vi "Actor Core.vi"(8 "error in":errorcluster, 11 "DataLogger in":refnum<class "DataLogger.lvclass">) -> (0 "error out":errorcluster, 3 "Actor out":refnum<class "Actor.lvclass">)   [LabVIEW 2019, in "DataLogger.lvclass"]
doc: "(<B>Filename</B>: Actor Framework.lvlib:Actor.lvclass:Actor Core.vi)\n\nReceives messages to the actor, reacts to them, and initiates any error handling that may shut the actor down.\n\nDescendant classes may override this VI to append parallel tasks for the actor to complete while it handles messages. Overrides use the Call Parent Method node."
uses:
  DataLogger.lvclass
  <vilib>/ActorFramework/Actor/Actor.lvclass
  <vilib>/drjdpowell/SQLite Library/SQL Connection/Execute SQL (No results).vi
  <vilib>/drjdpowell/SQLite Library/SQL Connection/Connection.lvclass
  <vilib>/drjdpowell/SQLite Library/SQL Connection/Open (path).vi
  <vilib>/ActorFramework/Message Enqueuer/Message Enqueuer.lvclass
  <vilib>/vision/Image Controls.llb/IMAQ Image.ctl
  Common/Controls/AllPartInfo.ctl
  Controls/LocalData_DL.ctl
  <vilib>/Utility/file.llb/Write Delimited Spreadsheet (string).vi
  C:/Program Files/National Instruments/LabVIEW 2019/vi.lib/ActorFramework/Actor/Actor.lvclass
  Controls/LocalData_Measurements_DL.ctl
panel:
  in  "PartDetails":T1
  in  "Cluster":T2={"Core"={"Current VI Reference"=refnum, "Close Panel on Exit?"=FALSE}, "AllPartInfoArray"=[{"PartName"="", "NumberOfRacks"=0, "MeasurementIDsArray"=[], "MeasurementNamesArray"=[], "SpecValuesArray"=[]}], "PartDetails"={"PartName"="", "OperatorName"="", "Initialize"=TRUE, "MeasurementEnable/DisableArray"=[], "NumberOfMeasurements"=0}, "BatchID"="", "MeasurementInfo"={"MeasurementDate"="", "MeasurementTime"="", "MeasurementResult"="", "MeasurementValueArray"=[]}, "MachineStatus"="", "CurrentState"="", "StateMessage"="", "MeasurementDetails"={"Array(2D)"=[], "IndexCounter"=0}, "RecordsInExcelCounter"=0, "ExcelSheetCounterPerReel"=0, "ReelCounterPerPart"=0, "WriteMeasurementData"=FALSE, "MeasurementExcelPath"=path "", "StripPath"=FALSE, "MasterSampleInfo"={"MSPartName"="", "MSDate"="", "MSTime"="", "MSMeasurementValueArray"=[], "MSResult"="", "NumberOfMeasurements"=0}, "MasterSampleDetails"={"Array(2D)"=[], "IndexCounter"=0}, "Stamping Mc Details"={"Customer Name"="", "Location"="", "StampingMcID"=""}}
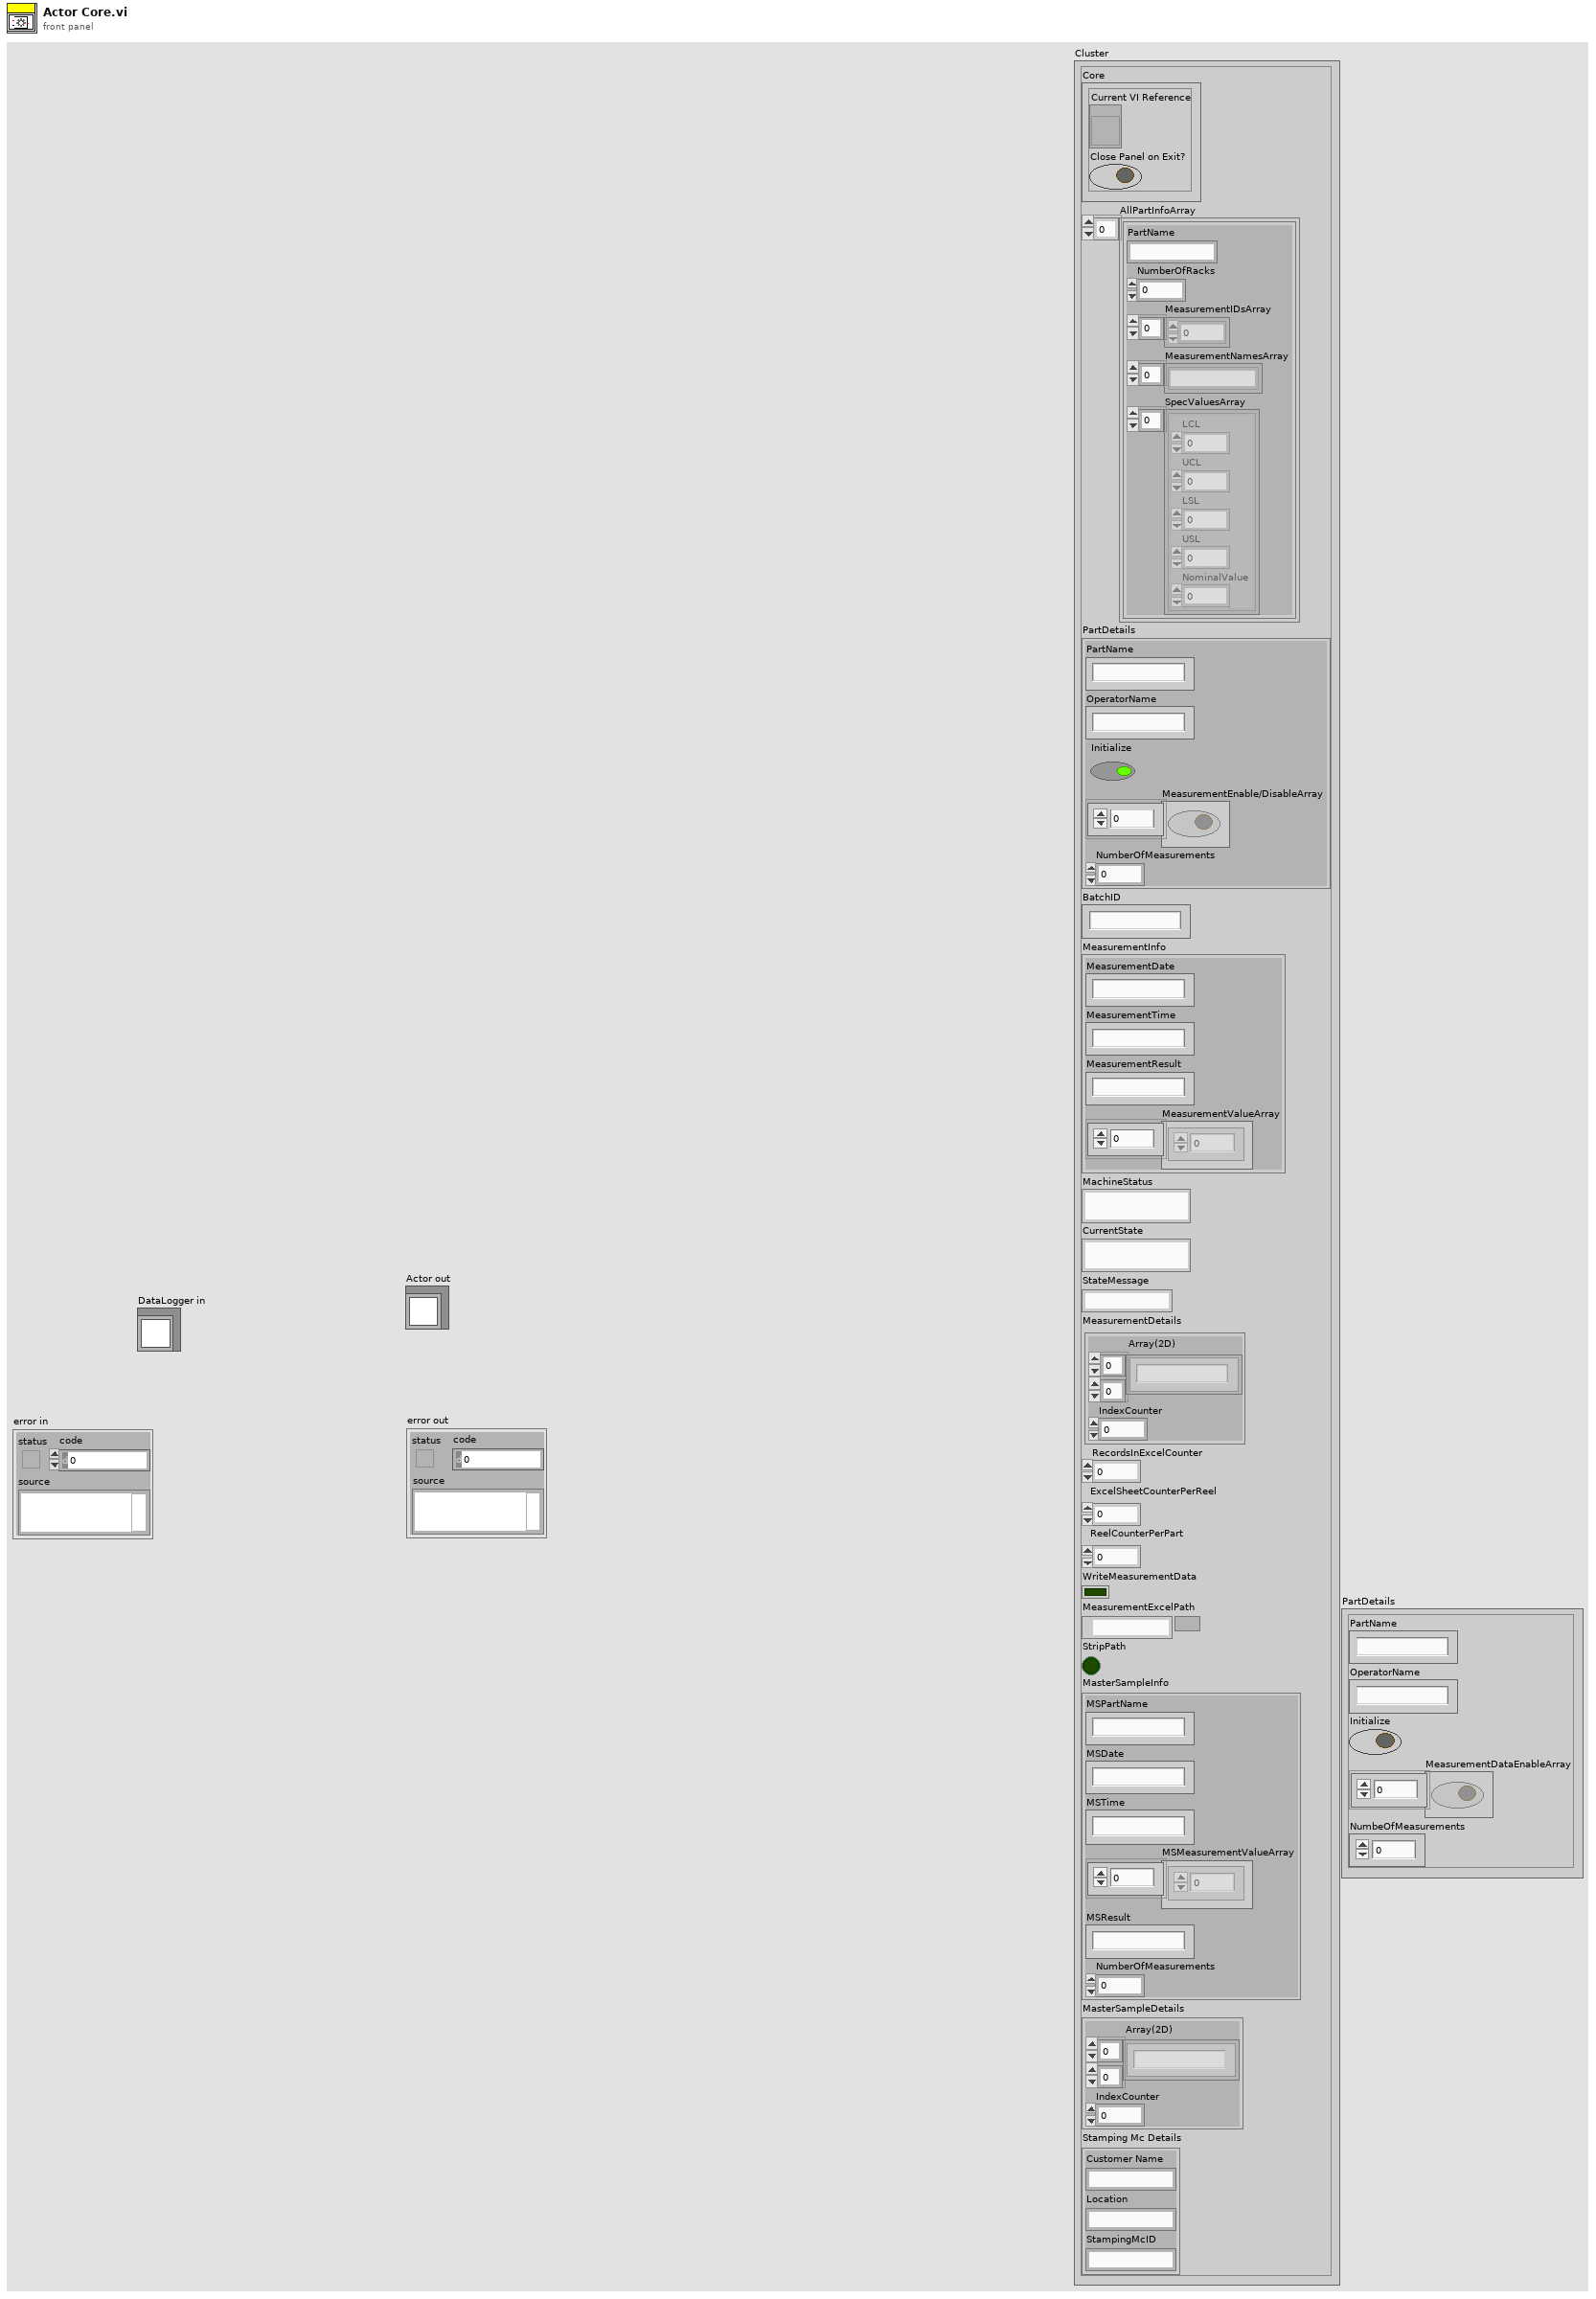
[diagram p1: front panel]
types:
  T1 = cluster{"PartName":string, "OperatorName":string, "Initialize":bool, "MeasurementDataEnableArray":bool[], "NumbeOfMeasurements":i32}
  T2 = typedef "DataLogger.lvclass/LocalData_Measurements_DL.ctl" = cluster{"Core":cluster{"Current VI Reference":refnum<vi>, "Close Panel on Exit?":bool}, "AllPartInfoArray":T3, "PartDetails":cluster{"PartName":string, "OperatorName":string, "Initialize":bool, "MeasurementEnable/DisableArray":bool[], "NumberOfMeasurements":i32}, "BatchID":string, "MeasurementInfo":cluster{"MeasurementDate":string, "MeasurementTime":string, "MeasurementResult":string, "MeasurementValueArray":dbl[]}, "MachineStatus":string, "CurrentState":string, "StateMessage":string, "MeasurementDetails":cluster{"Array(2D)":string[][], "IndexCounter":i32}, "RecordsInExcelCounter":i32, "ExcelSheetCounterPerReel":i32, "ReelCounterPerPart":i32, "WriteMeasurementData":bool, "MeasurementExcelPath":path, "StripPath":bool, "MasterSampleInfo":cluster{"MSPartName":string, "MSDate":string, "MSTime":string, "MSMeasurementValueArray":dbl[], "MSResult":string, "NumberOfMeasurements":i32}, "MasterSampleDetails":cluster{"Array(2D)":string[][], "IndexCounter":i32}, "Stamping Mc Details":cluster{"Customer Name":string, "Location":string, "StampingMcID":string}}
  T3 = typedef "AllPartInfo.ctl" = cluster{"PartName":string, "NumberOfRacks":u8, "MeasurementIDsArray":u16[], "MeasurementNamesArray":string[], "SpecValuesArray":cluster{"LCL":dbl, "UCL":dbl, "LSL":dbl, "USL":dbl, "NominalValue":dbl}[]}[]
  T4 = enum32{"invalid app kind", "Development System", "Run Time System", "Student Edition", "Embedded LabVIEW", "Evaluation", "Custom"}
  T5 = enum32{"Invalid", "Standard", "Closed", "Hidden", "Minimized", "Maximized"}
  T6 = cluster{"Current VI Reference":refnum<vi>, "Close Panel on Exit?":bool}
  T7 = cluster{"CreateNewEventsExcel":bool, "CreateNewFailExcel":bool, "CreateNewStatisticalExcel":bool, "CreateNewReelExcel":bool}
  T8 = cluster{"EventsSheetCounter":u32, "FailSheetCounter":u32, "StatisticalSheetCounter":u32, "ReelSheetCounter":u32}
  T9 = typedef "DataLogger.lvclass/LocalData_DL.ctl" = cluster{"Core":cluster{"Current VI Reference":refnum<vi>, "Close Panel on Exit?":bool}, "System Info":cluster{"System Name":string, "System ID":string, "Version":string, "Year":string, "Customer Details":cluster{"Customer Name":string, "Customer ID":string, "Location":string, "No of Shifts":u8, "Shift Details Array":cluster{"Name":string, "Timing":string}[]}, "Software Features":cluster{"IoT Enable":bool, "Datalogging Features":cluster{"Event Data":bool, "Measurement Data":bool, "Statistical Data":bool, "Reel Data":bool, "Failed Measurement Data":bool, "Failed Images":bool}, "IoT":cluster{"SMS Alert Enable":bool, "Email Alert Enable":bool}, "Popup Enable?":cluster{"Fail":bool, "Pause":bool, "Stop":bool}}}, "Part Info":cluster{"Part Name":string, "Rack ID":u8, "Initialize":bool, "StampingMc No":u64, "Operator Name":string, "ReelCount":u64, "TotalCount":u64, "Measurement Names Array":string[], "Measurement ID Array":u16[], "Spec Values Array":cluster{"LCL":dbl, "UCL":dbl, "LSL":dbl, "USL":dbl, "Nominal Value":dbl}[], "Camera Name Array":string[], "Measurement Enable/Disable Array":bool[], "Number of Measurements":i32}, "Fail Counter(For Event Details)":i32, "Event Details":cluster{"Event Name":string, "Event Time":string, "Event Reason":string, "Previous Event Name":string, "Previous Event Time":string}, "StatisticalInfo":string[][], "BatchInfo":cluster{"BatchPassCount":u64, "BatchFailCount":u64}, "Failure Details":cluster{"Fail Time Stamp":u64, "ControlPFArray":bool[], "SpecificationPFArray":dbl[], "Rack ID":u8, "Failed Image Array":T10[], "Fail Date":string, "Fail Time":string, "Fail Reason":string}, "SaveFailedImageCounter":i32, "AllPartInfoArray":T3, "Status":bool, "SpecValues(ForUpdate)":cluster{"LCL":dbl, "UCL":dbl, "LSL":dbl, "USL":dbl, "Nominal Value":dbl}, "AddSuccessfull":bool, "CurrentStateMessage":string, "IoTDetailsCounter":bool, "InitialUpdate":bool, "ResetUpdate":bool, "SetCounter":cluster{"MeasurementDetailsSetCounter":i32, "BatchDetailsSetCounter":i32, "FailureDetailsSetCounter":i32, "EventDetailsSetCounter":i32}, "IndexCounter":cluster{"MeasurementDetailsIndexCounter":i32, "BatchDetailsIndexCounter":i32, "FailureDetailsIndexCounter":i32, "EventDetailsIndexCounter":i32}, "Details2D":cluster{"MeasurementDetails(2D)":string[][], "BatchDetails(2D)":string[][], "FailureDetails(2D)":string[][], "EventDetails(2D)":string[][]}, "IDs":cluster{"Stamping McID":string, "Inspection McID":string, "BatchID":string, "FailID":string}, "Reel Info":cluster{"Reel No":u64, "Reel Start Time Stamp":u64}, "ExcelData":cluster{"StripPath":bool, "ReelCounterPerPart":i32, "FilePaths":cluster{"EventsFilePath":path, "FailFilePath":path, "ReelFilePath":path, "StatisticalFilePath":path}, "ExcelSheetCounterPerReel":cluster{"EventsSheetCounter":u32, "FailSheetCounter":u32, "StatisticalSheetCounter":u32, "ReelSheetCounter":u32}, "CreateNewExcel":cluster{"CreateNewEventsExcel":bool, "CreateNewFailExcel":bool, "CreateNewStatisticalExcel":bool, "CreateNewReelExcel":bool}, "RecordsInExcelCounter":cluster{"EventsRecordsCounter":u32, "FailRecordsCounter":u32, "ReelRecordsCounter":u32, "StatisticalRecordsCounter":u32}}, "SaveAck":cluster{"Loop1":bool, "Loop2":bool}, "Shift Statistical Info":cluster{"Shift Name":string, "Shift Timing":string, "Shift End Date":string, "Statistical Shift Data":cluster{"PartName":string, "MeasurementNames":string[], "Statistical Parameters":string[][]}[]}}
  T10 = typedef "IMAQ Image.ctl" = refnum<image>
  T11 = cluster{"Customer Name":string, "Customer ID":string, "Location":string, "No of Shifts":u8, "Shift Details Array":cluster{"Name":string, "Timing":string}[]}
  T12 = cluster{"IoT Enable":bool, "Datalogging Features":cluster{"Event Data":bool, "Measurement Data":bool, "Statistical Data":bool, "Reel Data":bool, "Failed Measurement Data":bool, "Failed Images":bool}, "IoT":cluster{"SMS Alert Enable":bool, "Email Alert Enable":bool}, "Popup Enable?":cluster{"Fail":bool, "Pause":bool, "Stop":bool}}
  T13 = cluster{"LCL":dbl, "UCL":dbl, "LSL":dbl, "USL":dbl, "Nominal Value":dbl}[]
  T14 = cluster{"PartName":string, "MeasurementNames":string[], "Statistical Parameters":string[][]}[]
  T15 = cluster{"EventsRecordCounter":u32, "FailRecordCounter":u32, "ReelRecordCounter":u32, "StatisticalRecordCounter":u32}
  T16 = cluster{"Acknowledgement":cluster{"Enqueuer":refnum<class "Message Enqueuer.lvclass">, "VIReference":refnum<vi>, "VIName":string}, "ErrorMessage":string}
  T17 = cluster{"Customer ID":string, "Customer Name":string, "Location":string, "No of Shifts":u8, "Inspection McID":string, "Shift Details Array":cluster{"Name":string, "Timing":string}[], "IoT Enable":bool, "SMS Alert Enable":bool, "Email Alert Enable":bool, "FailPopupEnable":bool, "PausePopupEnable":bool, "StopPopupEnable":bool}
  T18 = cluster{"LCL":dbl, "UCL":dbl, "LSL":dbl, "USL":dbl, "NominalValue":dbl}[]
  T19 = cluster{"Inspection McID":string, "PartName":string, "MeasurementNamesArray":string[], "SpecValuesArray":cluster{"LCL":dbl, "UCL":dbl, "LSL":dbl, "USL":dbl, "NominalValue":dbl}[]}
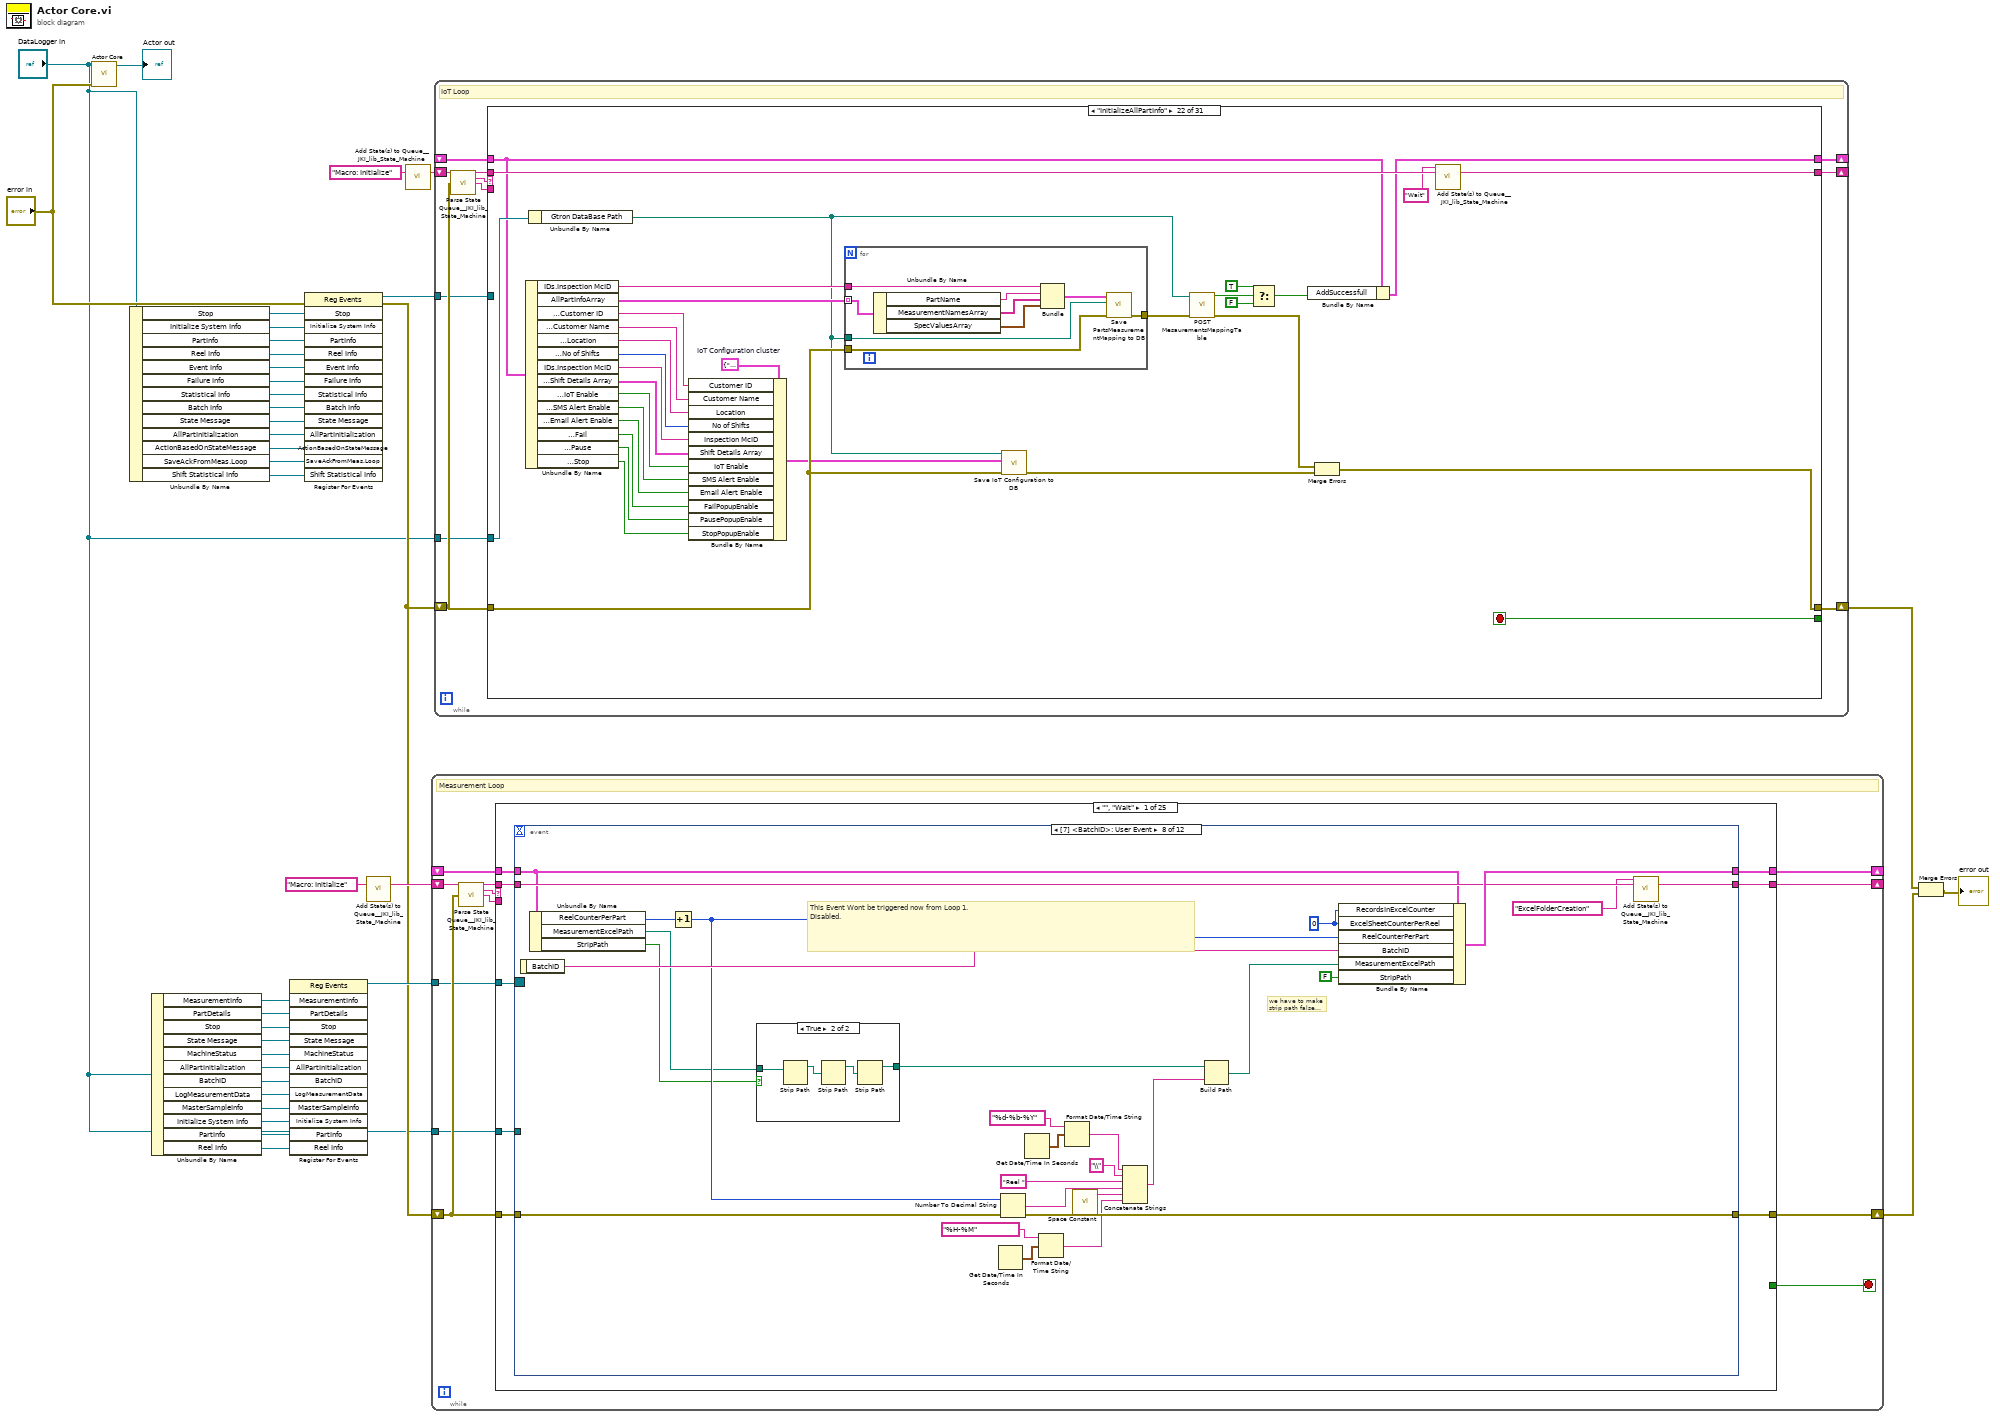
[diagram p0: block diagram]
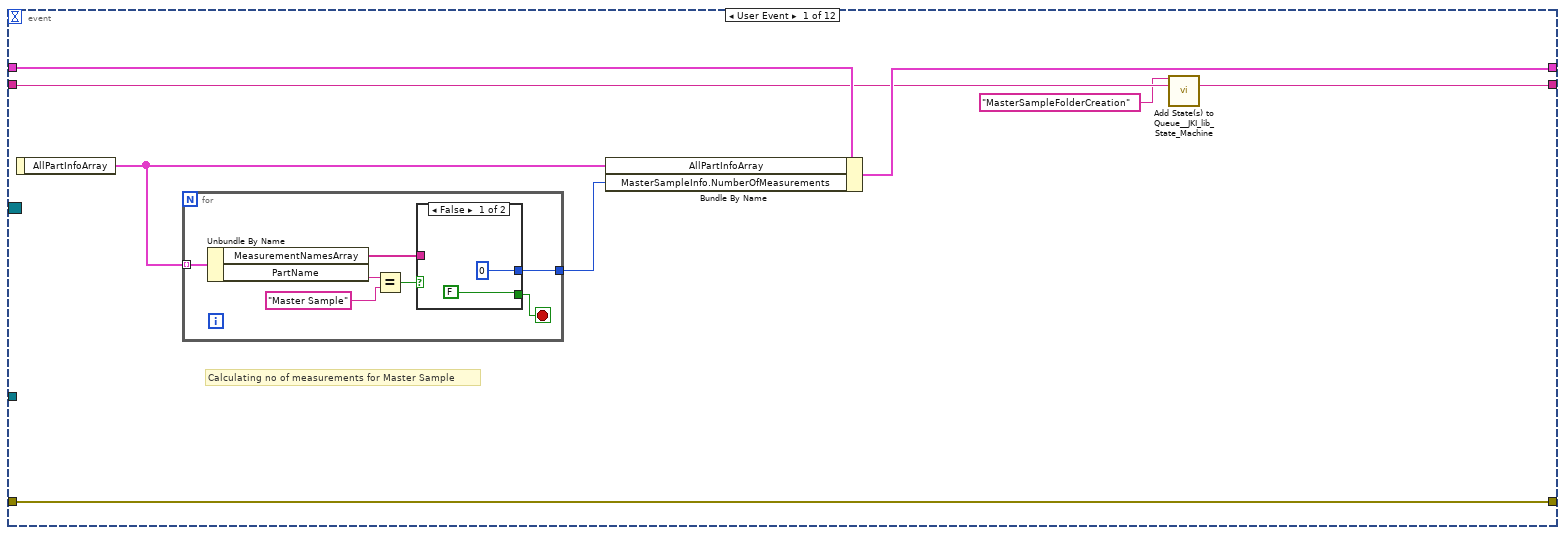
[diagram p2: hidden frame]
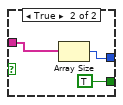
[diagram p3: hidden frame]
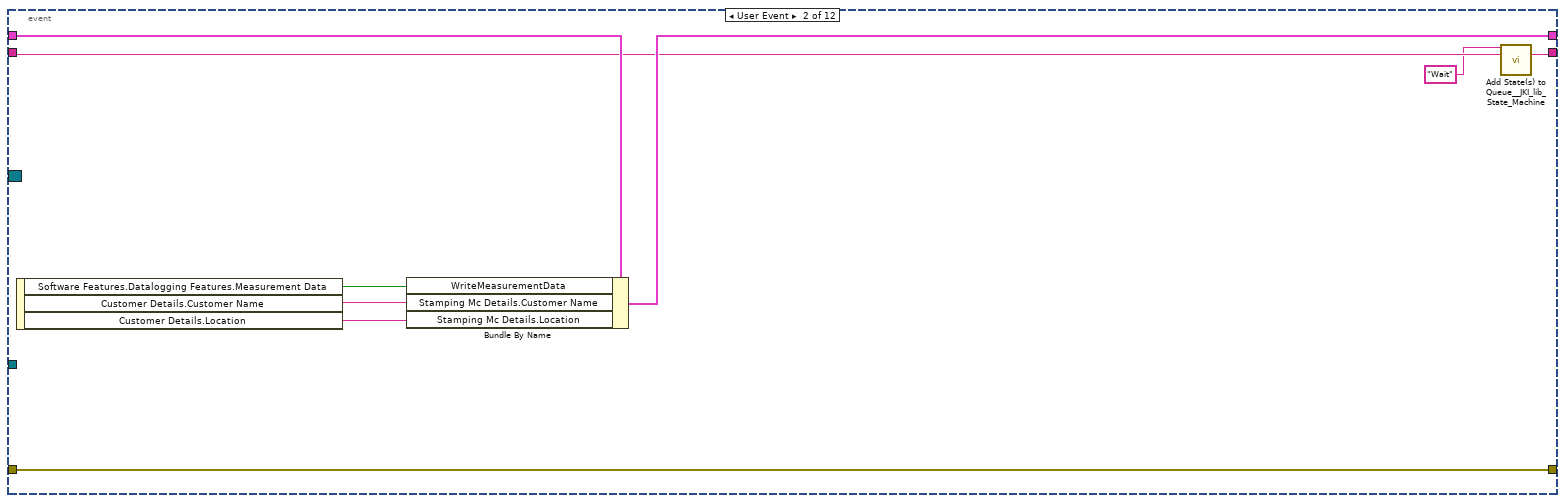
[diagram p4: hidden frame]
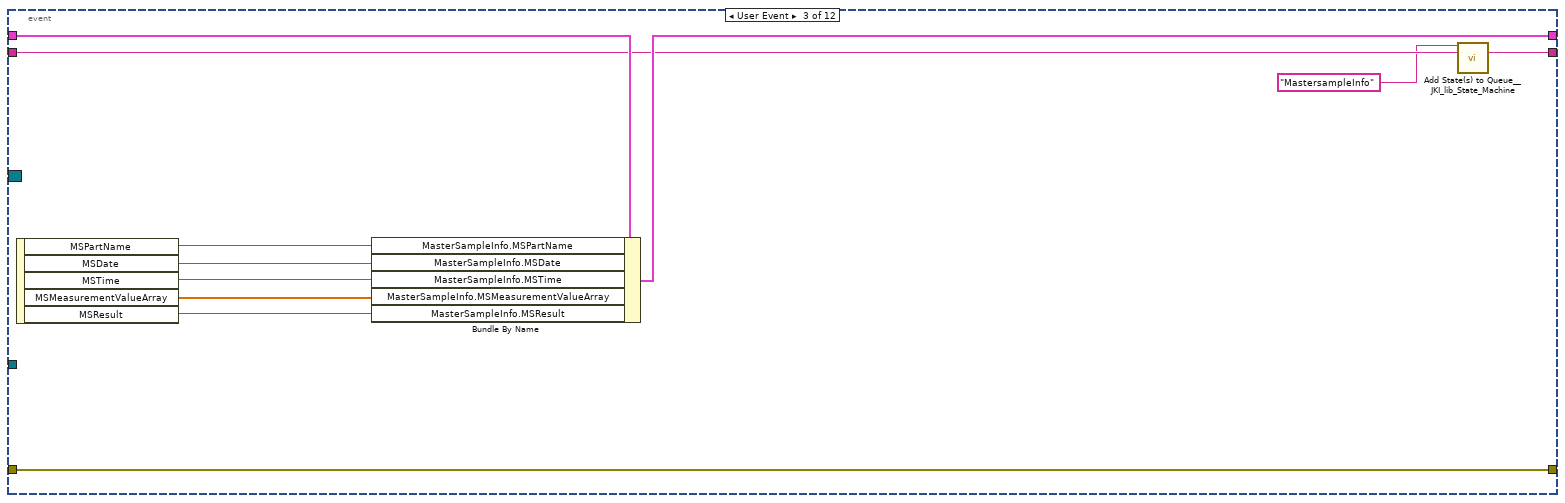
[diagram p5: hidden frame]
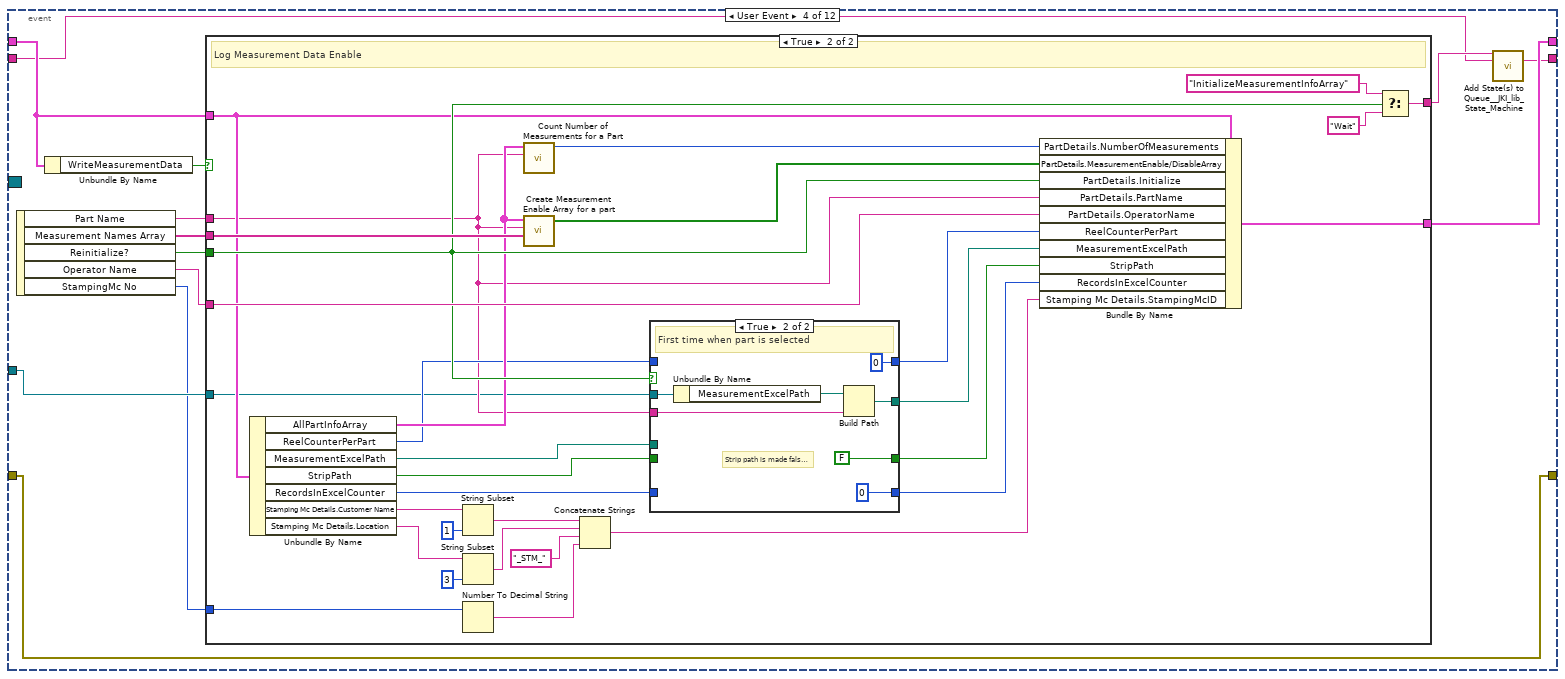
[diagram p6: hidden frame]
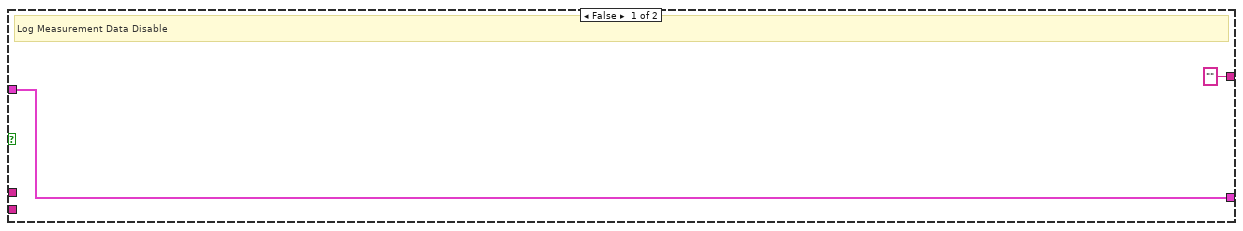
[diagram p7: hidden frame]
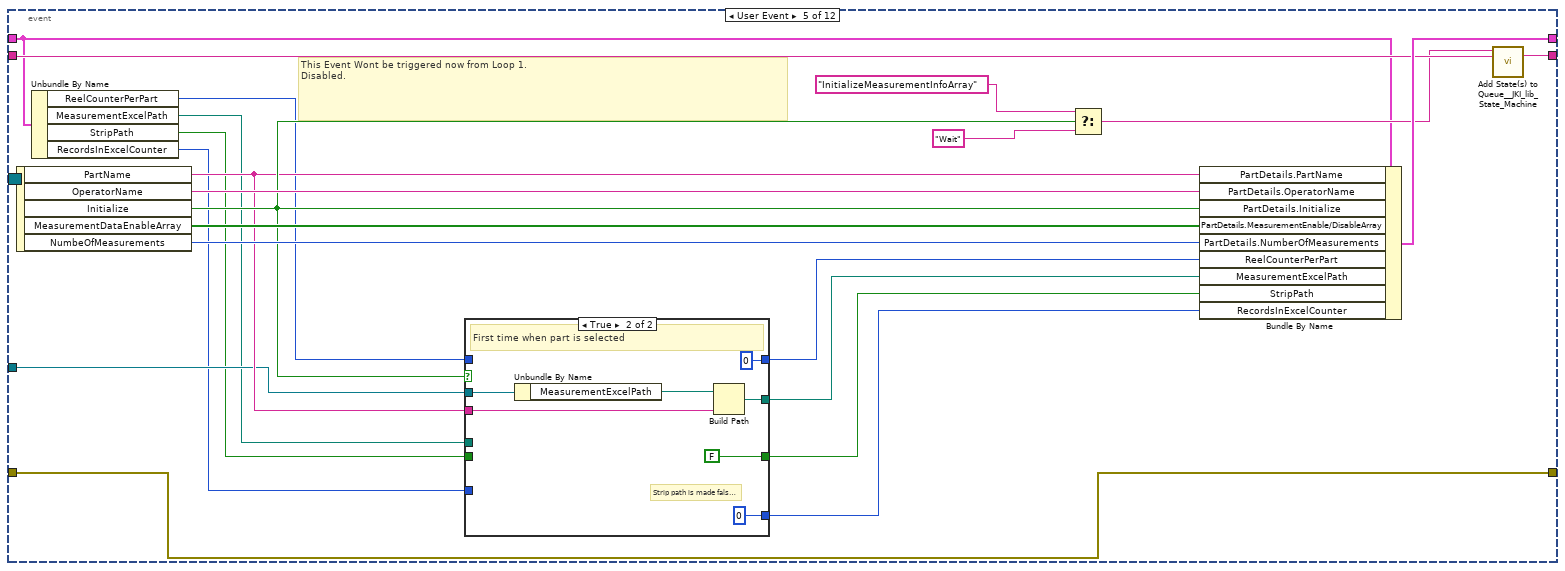
[diagram p9: hidden frame]
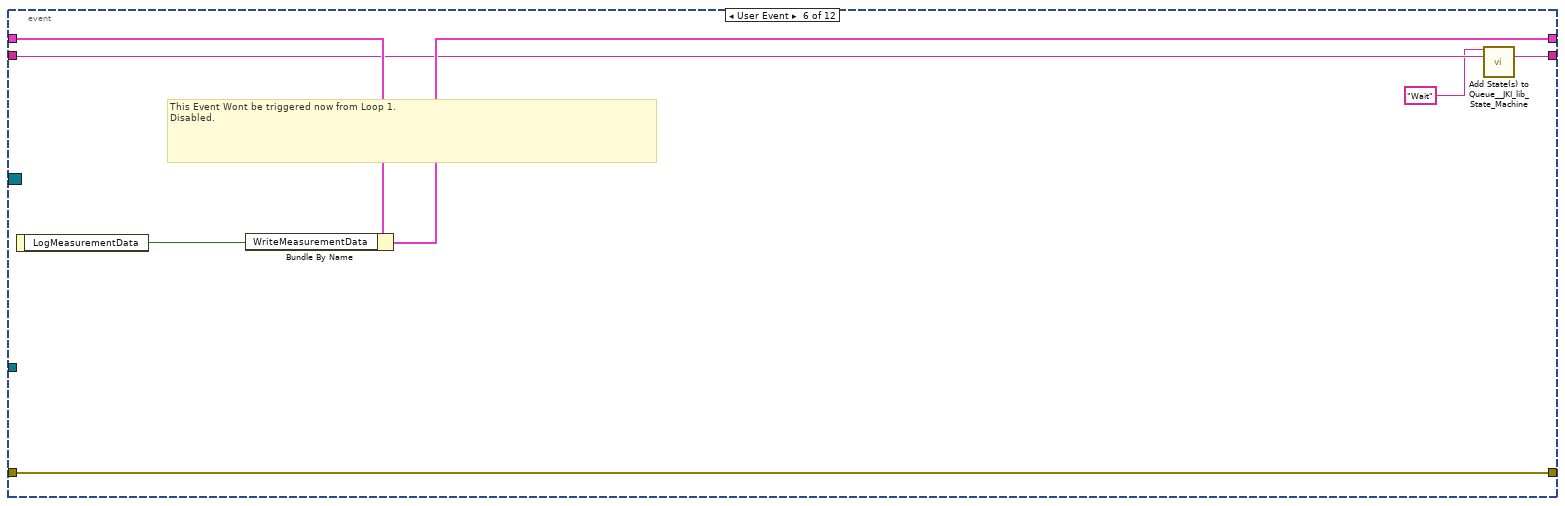
[diagram p11: hidden frame]
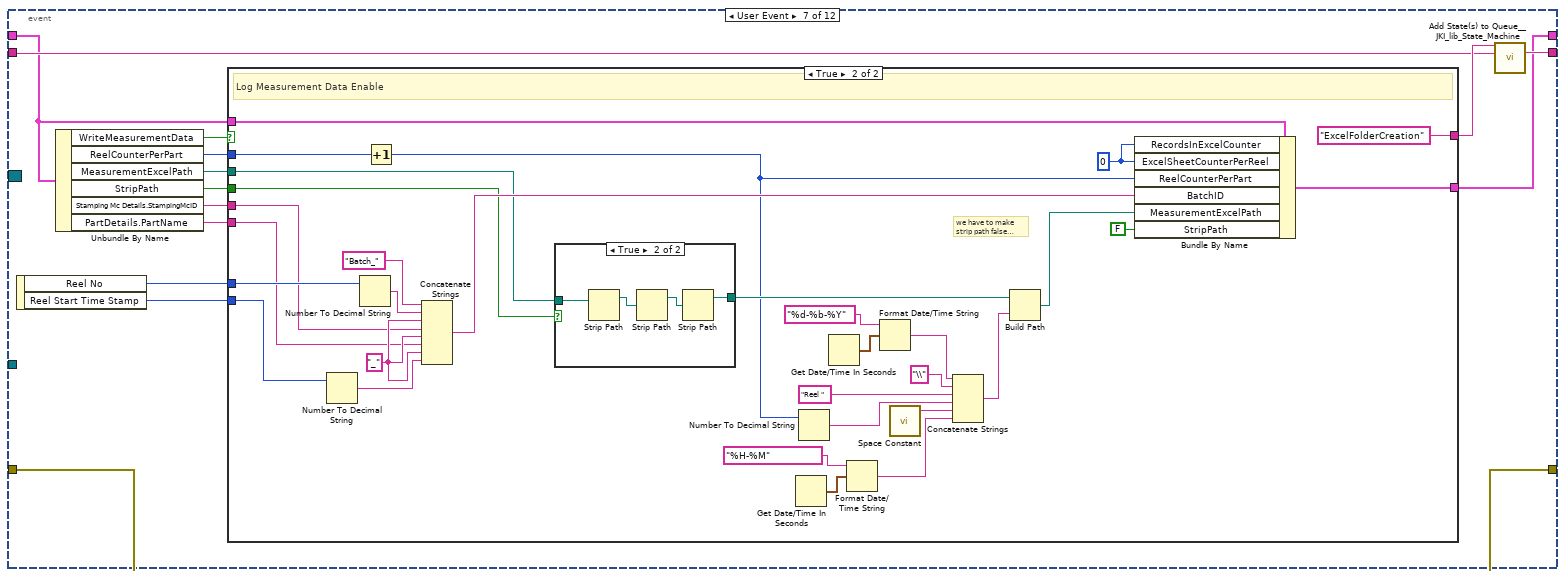
[diagram p12: hidden frame]
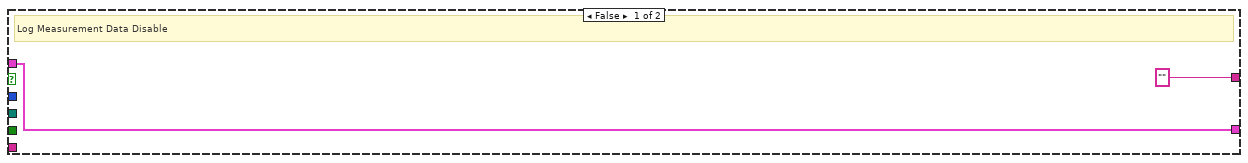
[diagram p13: hidden frame]
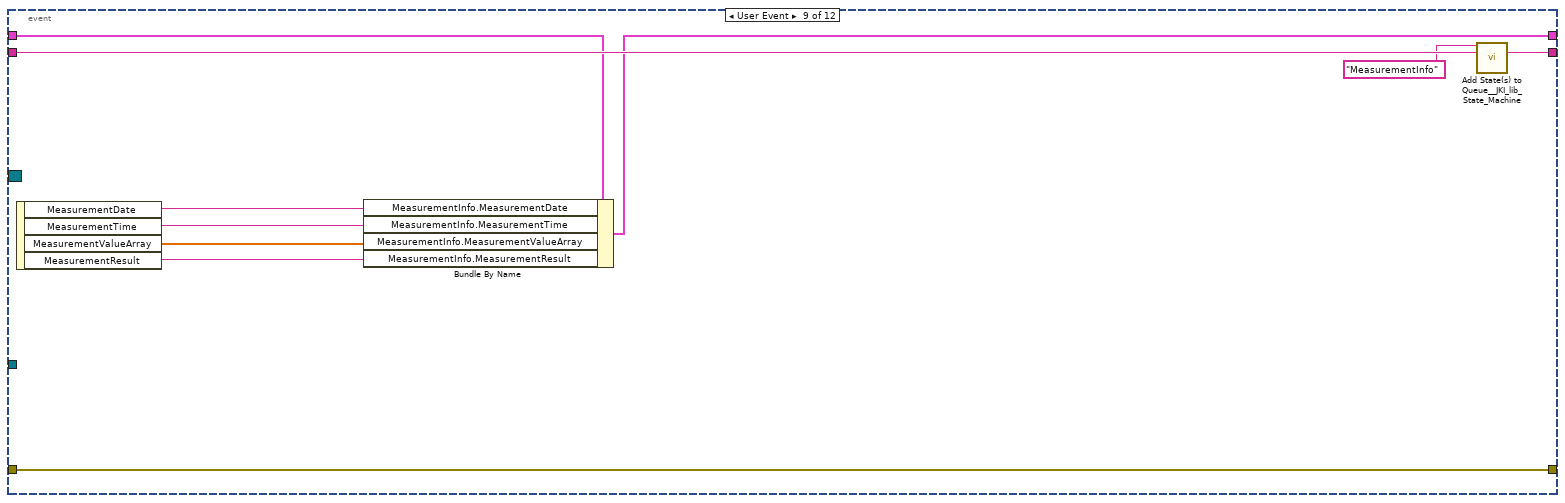
[diagram p16: hidden frame]
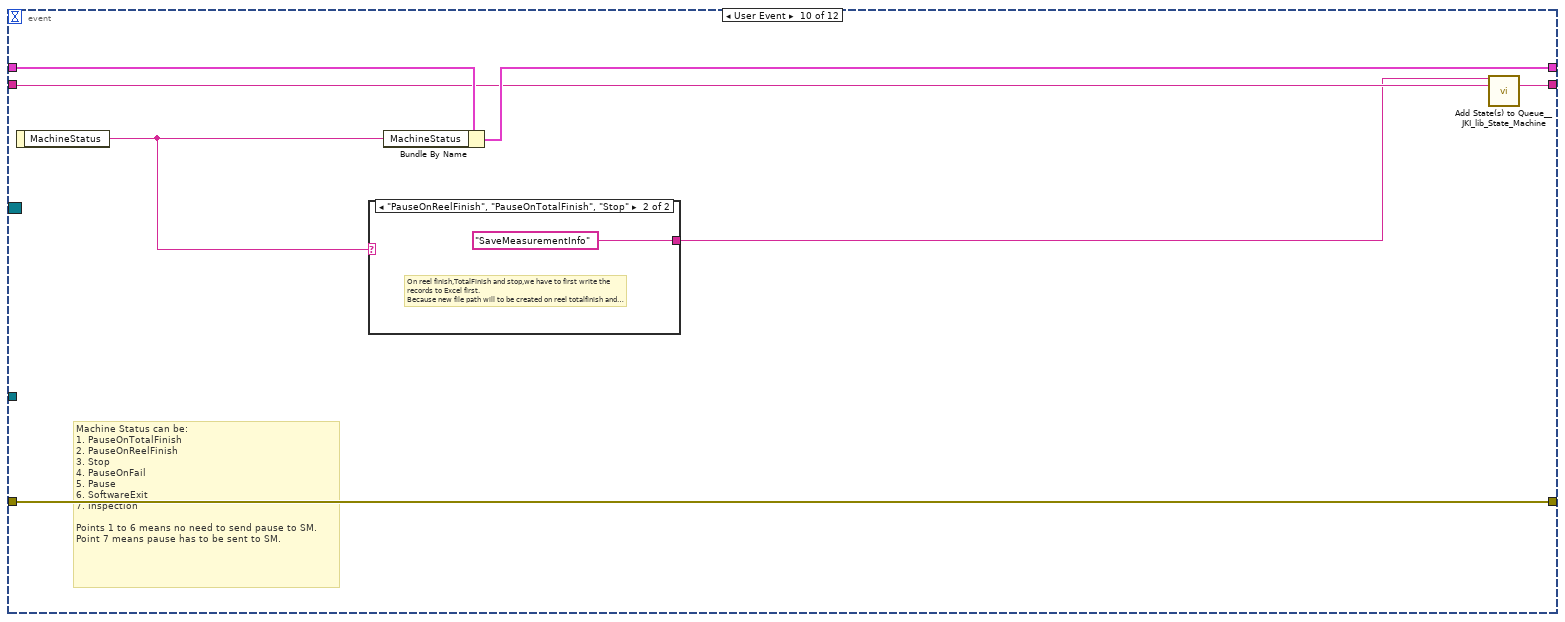
[diagram p17: hidden frame]
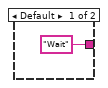
[diagram p18: hidden frame]
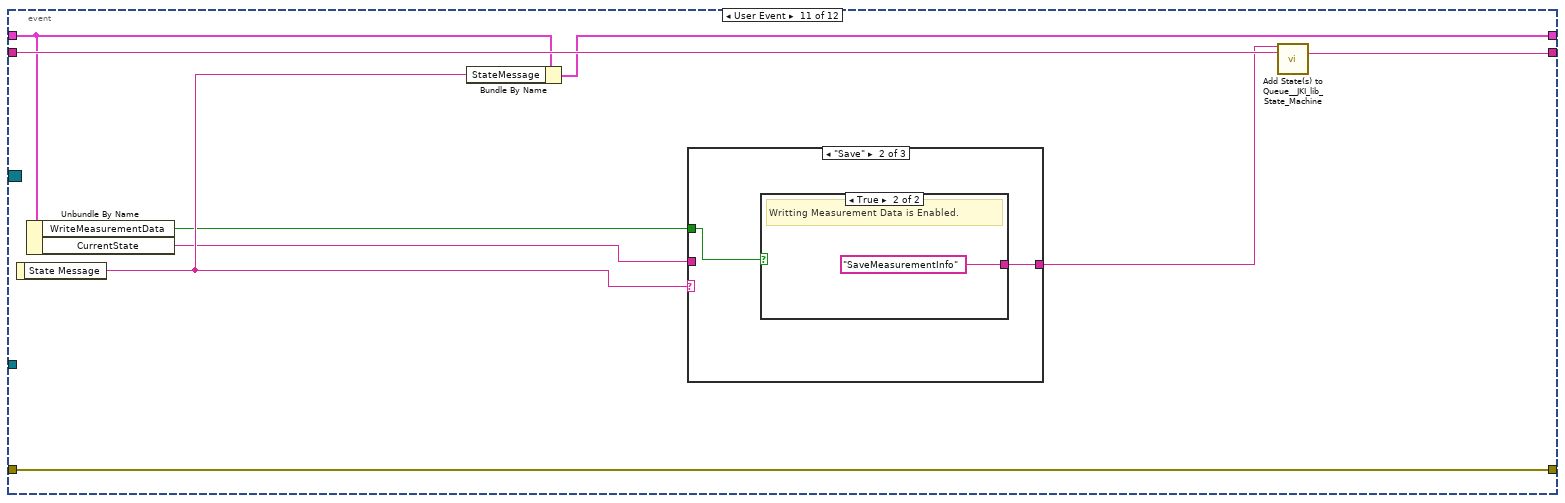
[diagram p19: hidden frame]
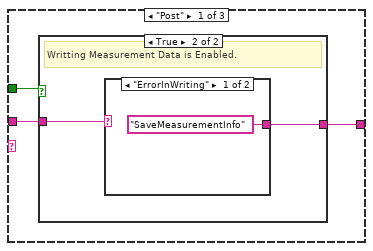
[diagram p20: hidden frame]
diagram:
  n1 = call-parent "Actor Core.vi"("error in"="error in", "Actor in"="DataLogger in") -> ("Actor out"=→"Actor out":refnum<class "Actor.lvclass">)  [unwired: 8 in, 1 out]
  n2 = Unbundle By Name("DataLogger in") -> ("Stop"=w35:refnum<user-event>, "Initialize System Info"=w33:refnum<user-event>, "PartInfo"=w32:refnum<user-event>, "Reel Info"=w31:refnum<user-event>, "Event Info"=w30:refnum<user-event>, "Failure Info"=w29:refnum<user-event>, "Statistical Info"=w28:refnum<user-event>, "Batch Info"=w27:refnum<user-event>, "State Message"=w26:refnum<user-event>, "AllPartInitialization"=w24:refnum<user-event>, "ActionBasedOnStateMessage"=w23:refnum<user-event>, "SaveAckFromMeas.Loop"=w7:refnum<user-event>, "Shift Statistical Info"=w4:refnum<user-event>)
  n3 = Unbundle By Name("DataLogger in") -> ("MeasurementInfo"=w20:refnum<user-event>, "PartDetails"=w18:refnum<user-event>, "Stop"=w13:refnum<user-event>, "State Message"=w12:refnum<user-event>, "MachineStatus"=w11:refnum<user-event>, "AllPartInitialization"=w10:refnum<user-event>, "BatchID"=w9:refnum<user-event>, "LogMeasurementData"=w6:refnum<user-event>, "MasterSampleInfo"=w5:refnum<user-event>, "Initialize System Info"=w3:refnum<user-event>, "PartInfo"=w2:refnum<user-event>, "Reel Info"=w1:refnum<user-event>)
  n4 = register-events(w20, w18, w13, w12, w11, w10, w9, w6, w5, w3, w2, w1) -> (reference out=w19:refnum<event-registration>)  [unwired: 2 in, 1 out]
  n5 = register-events(error in="error in", w35, w33, w32, w31, w30, w29, w28, w27, w26, w24, w23, w7, w4) -> (reference out=w34:refnum<event-registration>, error out=w17:errorcluster)  [unwired: 1 in]
  n6 = call <vilib>:"Add State(s) to Queue__JKI_lib_State_Machine.vi"("State(s) in (\"\")"="Macro: Initialize") -> ("States Out"=w22:string)  [unwired: 14 in]
  n7 = call <vilib>:"Add State(s) to Queue__JKI_lib_State_Machine.vi"("State(s) in (\"\")"="Macro: Initialize") -> ("States Out"=w37:string)  [unwired: 14 in]
  n8 = while "JKI - String-Based Queued State Machine (Basic) v1.0" {
    shift-right: [w43] -> _
    shift-left: _ -> [w42]
    shift-right: [w46] -> w14
    shift-left: w17 -> [w41]
    shift-right: [w45] -> _
    shift-left: w22 -> [w47]
    tunnel: w19 -> [w40]
    tunnel: "DataLogger in" -> [w39]
    stop <- w44 stop-if-true
    # "Measurement Loop"
    n9 = call <vilib>:"Parse State Queue__JKI_lib_State_Machine.vi"("State Queue"=w47, "Error In (no error)"=w41) -> ("Remaining States"=w49:string, "Current State"=w50:string, "Arguments"=w48:string)  [unwired: 11 in]
    n10 = case shown="\"\", \"Wait\"" w50 {
      selector: w50 -> [_ _ w329 _ _ _ _ _ _ _ _ _ _ _ _ _ _ _ _ _ _ _ _ _ _]
      tunnel: w49 -> [w58 w328 w333 w351 w356 w361 w365 w376 w406 w410 w414 w420 w431 w457 w462 w467 w471 w496 w510 w551 w555 w592 w620 w636 w694]
      tunnel: w48 -> [_ _ _ _ _ _ _ _ _ _ _ w415 w425 _ _ _ _ _ _ _ _ _ _ _ _]
      tunnel: w42 -> [w56 w325 w331 w342 w353 w359 w362 _ w402 w407 w412 w418 w427 w454 w459 w464 w468 w479 w512 w540 w552 w580 w614 w633 w688]
      tunnel: [w55 w326 w335 w348 errorcluster {"status"=FALSE, "code"=0, "source"=""} ("error out") w358 w363 w374 w384 w408 w411 w416 w428 w455 w460 w465 w469 w481 w508 w549 w553 w568 w618 w634 w682] -> w46
      tunnel: w41 -> [w54 w326 w334 w348 _ w358 w363 w374 w403 w408 w411 w417 w429 w455 w460 w465 w469 w482 w508 w549 w553 w588 w618 w634 w684]
      tunnel: [w57 w327 w332 w350 w355 w360 w364 w375 w405 w409 w413 w419 w430 w456 w461 w466 w470 w495 w513 w550 w554 w591 w619 w635 w693] -> w45
      tunnel: [_ _ _ _ _ TRUE _ _ _ _ _ _ _ _ _ _ _ _ _ _ _ _ _ _ _] -> w44
      tunnel: [w53 w325 w331 w349 w353 w359 w362 w371 w402 w407 w412 w418 w427 w454 w459 w464 w468 w478 w511 w539 w552 w579 w617 w632 w689] -> w43
      tunnel: w40 -> [w52 _ _ _ _ _ _ _ w385 _ _ _ _ _ _ _ _ _ _ _ _ _ _ _ _]
      tunnel: w39 -> [w51 _ _ _ _ _ _ _ w386 _ _ _ _ _ _ _ _ w487 _ w542 _ _ _ _ w683]
      frame "", "Wait" {
        n11 = event shown="[7] <BatchID>: User Event" {
          selector: w52 -> [_ _ _ _ _ _ _ _ _ _ _ _]
          dyn-events: _ -> [_ _ _ _ _ _ _ _ _ _ _ _]
          timeout: _ -> [_ _ _ _ _ _ _ _ _ _ _ _]
          tunnel: w58 -> [w63 w82 w89 w100 w172 w191 w202 w270 w287 w292 w305 w323]
          tunnel: [w64 w83 w90 w102 w173 w192 w201 w271 w288 w293 w306 w324] -> w57
          tunnel: w56 -> [w66 w86 w97 w106 w164 w194 w200 w267 w285 w295 w303 w320]
          tunnel: [w61 w87 w98 w111 w168 w195 w209 w268 w286 w291 w304 w321] -> w55
          tunnel: w54 -> [w61 w87 w98 w111 w168 w195 w209 w268 w286 w291 w304 w321]
          tunnel: [w65 w84 w91 w108 w177 w193 w199 w273 w284 w294 w302 w320] -> w53
          tunnel: w51 -> [_ _ _ w103 w165 _ _ _ _ _ _ _]
          event User Event {
            # "Calculating no of measurements for Master Sample"
            n12 = event-data() -> ("AllPartInfoArray"=w60:T3)  [unwired: 1 in]
            n13 = for {
              tunnel: w60 -> [w73] mode=indexing
              tunnel: [w69] -> w59
              stop <- w68 stop-if-true
              n14 = Unbundle By Name(w73) -> ("MeasurementNamesArray"=w70:string[], "PartName"=w72:string)
              n15 = Equal?(x=w72, y="Master Sample") -> (x = y?=w71:bool)
              n16 = case shown="False" w71 {
                tunnel: w70 -> [_ w78]
                tunnel: [0 w77] -> w69
                tunnel: [FALSE TRUE] -> w68
                frame False {
                }
                frame True {
                  n17 = Array Size(array=w78) -> (size(s)=w77:i32)
                }
              }
            }
            n18 = Bundle By Name(cluster=w66, "AllPartInfoArray"=w60, "MasterSampleInfo.NumberOfMeasurements"=w59) -> (w65:T2)
            n19 = call <vilib>:"Add State(s) to Queue__JKI_lib_State_Machine.vi"("State(s) in Front (\"\")"="MasterSampleFolderCreation" ("State(s) in Front (\"\")"), "State(s) in (\"\")"=w63) -> ("States Out"=w64:string)  [unwired: 13 in]
          }
          event User Event {
            n20 = event-data() -> ("Software Features.Datalogging Features.Measurement Data"=w85:bool, "Customer Details.Customer Name"=w79:string, "Customer Details.Location"=w80:string)  [unwired: 1 in]
            n21 = Bundle By Name(cluster=w86, "WriteMeasurementData"=w85, "Stamping Mc Details.Customer Name"=w79, "Stamping Mc Details.Location"=w80) -> (w84:T2)
            n22 = call <vilib>:"Add State(s) to Queue__JKI_lib_State_Machine.vi"("State(s) in Front (\"\")"="Wait" ("State(s) in Front (\"\")"), "State(s) in (\"\")"=w82) -> ("States Out"=w83:string)  [unwired: 13 in]
          }
          event User Event {
            n23 = event-data() -> ("MSPartName"=w92:string, "MSDate"=w93:string, "MSTime"=w94:string, "MSMeasurementValueArray"=w95:dbl[], "MSResult"=w96:string)  [unwired: 1 in]
            n24 = Bundle By Name(cluster=w97, "MasterSampleInfo.MSPartName"=w92, "MasterSampleInfo.MSDate"=w93, "MasterSampleInfo.MSTime"=w94, "MasterSampleInfo.MSMeasurementValueArray"=w95, "MasterSampleInfo.MSResult"=w96) -> (w91:T2)
            n25 = call <vilib>:"Add State(s) to Queue__JKI_lib_State_Machine.vi"("State(s) in Front (\"\")"="MastersampleInfo" ("State(s) in Front (\"\")"), "State(s) in (\"\")"=w89) -> ("States Out"=w90:string)  [unwired: 13 in]
          }
          event User Event {
            n26 = event-data() -> ("Part Name"=w110:string, "Measurement Names Array"=w109:string[], "Reinitialize?"=w107:bool, "Operator Name"=w104:string, "StampingMc No"=w99:u64)  [unwired: 1 in]
            n27 = Unbundle By Name(w106) -> ("WriteMeasurementData"=w105:bool)
            n28 = case shown="True" w105 {
              tunnel: w110 -> [_ w129]
              tunnel: w109 -> [_ w144]
              tunnel: [w113 w143] -> w108
              tunnel: ["" ("State(s) in Front (\"\")") w140] -> w101
              tunnel: w107 -> [_ w136]
              tunnel: w106 -> [w113 w135]
              tunnel: w104 -> [_ w137]
              tunnel: w103 -> [_ w125]
              tunnel: w99 -> [_ w117]
              frame False {
                # "Log Measurement Data Disable"
              }
              frame True {
                # "Log Measurement Data Enable"
                n29 = Unbundle By Name(w135) -> ("AllPartInfoArray"=w134:T3, "ReelCounterPerPart"=w133:i32, "MeasurementExcelPath"=w132:path, "StripPath"=w131:bool, "RecordsInExcelCounter"=w130:i32, "Stamping Mc Details.Customer Name"=w116:string, "Stamping Mc Details.Location"=w115:string)
                n30 = String Subset(string=w116, length (rest)=1 ("length (rest)")) -> (substring=w121:string)  [unwired: 1 in]
                n31 = String Subset(string=w115, length (rest)=3 ("length (rest)")) -> (substring=w120:string)  [unwired: 1 in]
                n32 = Number To Decimal String(number=w117) -> (decimal integer string=w118:string)  [unwired: 1 in]
                n33 = call "Count Number of Measurements for a Part.vi"("Part Name"=w129, "AllPartInfoArray"=w134) -> ("Number of Measurements"=w139:i32)  [unwired: 9 in]
                n34 = call "Create Measurement Enable Array for a part.vi"("Measurement Names Array"=w144, "Part Name"=w129, "AllPartInfoArray"=w134) -> ("Measurement Enable Array"=w138:bool[])  [unwired: 8 in]
                n35 = Concatenate Strings(w121, w120, "_STM_" ("string"), w118) -> (w114:string)
                n36 = case shown="True" w136 {
                  tunnel: w125 -> [_ w155]
                  tunnel: w129 -> [_ w154]
                  tunnel: [w147 w153] -> w127
                  tunnel: w133 -> [w148 _]
                  tunnel: [w148 0 ("ReelCounterPerPart")] -> w128
                  tunnel: w132 -> [w147 _]
                  tunnel: [w146 FALSE ("StripPath")] -> w126
                  tunnel: w131 -> [w146 _]
                  tunnel: w130 -> [w145 _]
                  tunnel: [w145 0 ("ReelCounterPerPart")] -> w124
                  frame False {
                    # "During update"
                  }
                  frame True {
                    # "Strip path is made false as file is being built from starting"
                    # "First time when part is selected"
                    n37 = Unbundle By Name(w155) -> ("MeasurementExcelPath"=w151:path)
                    n38 = Build Path(base path=w151, name or relative path=w154) -> (appended path=w153:path)
                  }
                }
                n39 = Bundle By Name(cluster=w135, "PartDetails.NumberOfMeasurements"=w139, "PartDetails.MeasurementEnable/DisableArray"=w138, "PartDetails.Initialize"=w136, "PartDetails.PartName"=w129, "PartDetails.OperatorName"=w137, "ReelCounterPerPart"=w128, "MeasurementExcelPath"=w127, "StripPath"=w126, "RecordsInExcelCounter"=w124, "Stamping Mc Details.StampingMcID"=w114) -> (w143:T2)
                n40 = Select(t="InitializeMeasurementInfoArray" ("State(s) in Front (\"\")"), s=w136, f="Wait" ("State(s) in Front (\"\")")) -> (s? t:f=w140:string)
              }
            }
            n41 = call <vilib>:"Add State(s) to Queue__JKI_lib_State_Machine.vi"("State(s) in Front (\"\")"=w101, "State(s) in (\"\")"=w100) -> ("States Out"=w102:string)  [unwired: 13 in]
          }
          event User Event {
            # "This Event Wont be triggered now from Loop 1.\nDisabled."
            n42 = event-data() -> ("PartName"=w166:string, "OperatorName"=w174:string, "Initialize"=w167:bool, "MeasurementDataEnableArray"=w175:bool[], "NumbeOfMeasurements"=w176:i32)  [unwired: 1 in]
            n43 = Unbundle By Name(w164) -> ("ReelCounterPerPart"=w163:i32, "MeasurementExcelPath"=w160:path, "StripPath"=w159:bool, "RecordsInExcelCounter"=w158:i32)
            n44 = case shown="True" w167 {
              tunnel: w165 -> [_ w188]
              tunnel: w166 -> [_ w187]
              tunnel: [w180 w186] -> w161
              tunnel: w163 -> [w181 _]
              tunnel: [w181 0 ("ReelCounterPerPart")] -> w162
              tunnel: w160 -> [w180 _]
              tunnel: [w179 FALSE ("StripPath")] -> w156
              tunnel: w159 -> [w179 _]
              tunnel: w158 -> [w178 _]
              tunnel: [w178 0 ("ReelCounterPerPart")] -> w157
              frame False {
                # "During update"
              }
              frame True {
                # "Strip path is made false as file is being built from starting"
                # "First time when part is selected"
                n45 = Unbundle By Name(w188) -> ("MeasurementExcelPath"=w184:path)
                n46 = Build Path(base path=w184, name or relative path=w187) -> (appended path=w186:path)
              }
            }
            n47 = Select(t="InitializeMeasurementInfoArray" ("State(s) in Front (\"\")"), s=w167, f="Wait" ("State(s) in Front (\"\")")) -> (s? t:f=w170:string)
            n48 = Bundle By Name(cluster=w164, "PartDetails.PartName"=w166, "PartDetails.OperatorName"=w174, "PartDetails.Initialize"=w167, "PartDetails.MeasurementEnable/DisableArray"=w175, "PartDetails.NumberOfMeasurements"=w176, "ReelCounterPerPart"=w162, "MeasurementExcelPath"=w161, "StripPath"=w156, "RecordsInExcelCounter"=w157) -> (w177:T2)
            n49 = call <vilib>:"Add State(s) to Queue__JKI_lib_State_Machine.vi"("State(s) in Front (\"\")"=w170, "State(s) in (\"\")"=w172) -> ("States Out"=w173:string)  [unwired: 13 in]
          }
          event User Event {
            # "This Event Wont be triggered now from Loop 1.\nDisabled."
            n50 = event-data() -> ("LogMeasurementData"=w189:bool)  [unwired: 1 in]
            n51 = Bundle By Name(cluster=w194, "WriteMeasurementData"=w189) -> (w193:T2)
            n52 = call <vilib>:"Add State(s) to Queue__JKI_lib_State_Machine.vi"("State(s) in Front (\"\")"="Wait" ("State(s) in Front (\"\")"), "State(s) in (\"\")"=w191) -> ("States Out"=w192:string)  [unwired: 13 in]
          }
          event User Event {
            n53 = event-data() -> ("Reel No"=w208:u64, "Reel Start Time Stamp"=w206:u64)  [unwired: 1 in]
            n54 = Unbundle By Name(w200) -> ("WriteMeasurementData"=w207:bool, "ReelCounterPerPart"=w196:i32, "MeasurementExcelPath"=w197:path, "StripPath"=w198:bool, "Stamping Mc Details.StampingMcID"=w204:string, "PartDetails.PartName"=w205:string)
            n55 = case shown="True" w207 {
              tunnel: w208 -> [_ w238]
              tunnel: w206 -> [_ w224]
              tunnel: w205 -> [_ w223]
              tunnel: w204 -> [_ w222]
              tunnel: ["" ("State(s) in (\"\")") "ExcelFolderCreation" ("State(s) in (\"\")")] -> w203
              tunnel: w200 -> [w210 w219]
              tunnel: [w210 w218] -> w199
              tunnel: w198 -> [_ w215]
              tunnel: w197 -> [_ w214]
              tunnel: w196 -> [_ w213]
              frame False {
                # "Log Measurement Data Disable"
              }
              frame True {
                w239 = 0 ("ExcelSheetCounterPerReel")
                w225 = "_" ("string")
                # "we have to make strip path false otherwise path will again be stripped(which we dont want)\nin ExcelFoldercreation state."
                # "Log Measurement Data Enable"
                n56 = Number To Decimal String(number=w224) -> (decimal integer string=w242:string)  [unwired: 1 in]
                n57 = Number To Decimal String(number=w238) -> (decimal integer string=w241:string)  [unwired: 1 in]
                n58 = Increment(x=w213) -> (x+1=w212:i32)
                n59 = Concatenate Strings("Batch_" ("string"), w241, w225, w222, w225, w223, w225, w242) -> (w221:string)
                n60 = case shown="True" w215 {
                  tunnel: w214 -> [w243 w247]
                  tunnel: [w243 w245] -> w216
                  frame False {
                  }
                  frame True {
                    n61 = Strip Path(path=w247) -> (stripped path=w246:path)  [unwired: 1 out]
                    n62 = Strip Path(path=w246) -> (stripped path=w244:path)  [unwired: 1 out]
                    n63 = Strip Path(path=w244) -> (stripped path=w245:path)  [unwired: 1 out]
                  }
                }
                n64 = Get Date/Time In Seconds() -> (seconds since 1Jan1904=w233:timestamp)
                n65 = Number To Decimal String(number=w212) -> (decimal integer string=w234:string)  [unwired: 1 in]
                n66 = Get Date/Time In Seconds() -> (seconds since 1Jan1904=w229:timestamp)
                n67 = Format Date/Time String(time format string (%c)="%H-%M", seconds (now)=w233) -> (date/time string=w230:string)  [unwired: 1 in]
                n68 = Format Date/Time String(time format string (%c)="%d-%b-%Y", seconds (now)=w229) -> (date/time string=w227:string)  [unwired: 1 in]
                n69 = call <vilib>:"Space Constant.vi"() -> ("String"=w231:string)
                n70 = Concatenate Strings(w227, "\\" ("string"), "Reel ", w234, w231, w230) -> (w236:string)
                n71 = Build Path(base path=w216, name or relative path=w236) -> (appended path=w217:path)
                n72 = Bundle By Name(cluster=w219, "RecordsInExcelCounter"=w239, "ExcelSheetCounterPerReel"=w239, "ReelCounterPerPart"=w212, "BatchID"=w221, "MeasurementExcelPath"=w217, "StripPath"=FALSE) -> (w218:T2)
              }
            }
            n73 = call <vilib>:"Add State(s) to Queue__JKI_lib_State_Machine.vi"("State(s) in Front (\"\")"=w203, "State(s) in (\"\")"=w202) -> ("States Out"=w201:string)  [unwired: 13 in]
          }
          event User Event {
            w249 = 0 ("ExcelSheetCounterPerReel")
            # "This Event Wont be triggered now from Loop 1.\nDisabled."
            # "we have to make strip path false otherwise path will again be stripped(which we dont want)\nin ExcelFoldercreation state."
            n74 = event-data() -> ("BatchID"=w272:string)  [unwired: 1 in]
            n75 = Unbundle By Name(w267) -> ("ReelCounterPerPart"=w266:i32, "MeasurementExcelPath"=w256:path, "StripPath"=w248:bool)
            n76 = Increment(x=w266) -> (x+1=w257:i32)
            n77 = case shown="True" w248 {
              tunnel: w256 -> [w274 w278]
              tunnel: [w274 w276] -> w255
              frame False {
              }
              frame True {
                n78 = Strip Path(path=w278) -> (stripped path=w277:path)  [unwired: 1 out]
                n79 = Strip Path(path=w277) -> (stripped path=w275:path)  [unwired: 1 out]
                n80 = Strip Path(path=w275) -> (stripped path=w276:path)  [unwired: 1 out]
              }
            }
            n81 = Get Date/Time In Seconds() -> (seconds since 1Jan1904=w262:timestamp)
            n82 = Number To Decimal String(number=w257) -> (decimal integer string=w263:string)  [unwired: 1 in]
            n83 = Get Date/Time In Seconds() -> (seconds since 1Jan1904=w254:timestamp)
            n84 = Format Date/Time String(time format string (%c)="%H-%M", seconds (now)=w262) -> (date/time string=w259:string)  [unwired: 1 in]
            n85 = Format Date/Time String(time format string (%c)="%d-%b-%Y", seconds (now)=w254) -> (date/time string=w252:string)  [unwired: 1 in]
            n86 = call <vilib>:"Space Constant.vi"() -> ("String"=w260:string)
            n87 = Concatenate Strings(w252, "\\" ("string"), "Reel ", w263, w260, w259) -> (w265:string)
            n88 = Build Path(base path=w255, name or relative path=w265) -> (appended path=w258:path)
            n89 = Bundle By Name(cluster=w267, "RecordsInExcelCounter"=w249, "ExcelSheetCounterPerReel"=w249, "ReelCounterPerPart"=w257, "BatchID"=w272, "MeasurementExcelPath"=w258, "StripPath"=FALSE) -> (w273:T2)
            n90 = call <vilib>:"Add State(s) to Queue__JKI_lib_State_Machine.vi"("State(s) in Front (\"\")"="ExcelFolderCreation" ("State(s) in (\"\")"), "State(s) in (\"\")"=w270) -> ("States Out"=w271:string)  [unwired: 13 in]
          }
          event User Event {
            n91 = event-data() -> ("MeasurementDate"=w281:string, "MeasurementTime"=w282:string, "MeasurementValueArray"=w280:dbl[], "MeasurementResult"=w283:string)  [unwired: 1 in]
            n92 = Bundle By Name(cluster=w285, "MeasurementInfo.MeasurementDate"=w281, "MeasurementInfo.MeasurementTime"=w282, "MeasurementInfo.MeasurementValueArray"=w280, "MeasurementInfo.MeasurementResult"=w283) -> (w284:T2)
            n93 = call <vilib>:"Add State(s) to Queue__JKI_lib_State_Machine.vi"("State(s) in Front (\"\")"="MeasurementInfo" ("State(s) in Front (\"\")"), "State(s) in (\"\")"=w287) -> ("States Out"=w288:string)  [unwired: 13 in]
          }
          event User Event {
            # "Machine Status can be:\n1. PauseOnTotalFinish\n2. PauseOnReelFinish\n3. Stop\n4. PauseOnFail\n5. Pause\n6. SoftwareExit\n7. Inspection\n\nPoints 1 to 6 means no need to send pause to SM.\nPoint 7 means pause has to be sent to SM."
            n94 = event-data() -> ("MachineStatus"=w290:string)  [unwired: 1 in]
            n95 = case shown="\"PauseOnReelFinish\", \"PauseOnTotalFinish\", \"Stop\"" w290 {
              tunnel: ["Wait" ("State(s) in Front (\"\")") "SaveMeasurementInfo" ("State(s) in Front (\"\")")] -> w289
              frame Default {
              }
              frame "PauseOnReelFinish", "PauseOnTotalFinish", "Stop" {
                # "On reel finish,TotalFinish and stop,we have to first write the records to Excel first.\nBecause new file path will to be created on reel totalfinish and stop inspection and old data will also be saved to the new path that will be created."
              }
            }
            n96 = Bundle By Name(cluster=w295, "MachineStatus"=w290) -> (w294:T2)
            n97 = call <vilib>:"Add State(s) to Queue__JKI_lib_State_Machine.vi"("State(s) in Front (\"\")"=w289, "State(s) in (\"\")"=w292) -> ("States Out"=w293:string)  [unwired: 13 in]
          }
          event User Event {
            n98 = event-data() -> ("State Message"=w300:string)  [unwired: 1 in]
            n99 = Unbundle By Name(w303) -> ("WriteMeasurementData"=w298:bool, "CurrentState"=w299:string)
            n100 = Bundle By Name(cluster=w303, "StateMessage"=w300) -> (w302:T2)
            n101 = case shown="\"Save\"" w300 {
              tunnel: [w309 w316 "Wait"] -> w301
              tunnel: w299 -> [w308 _ _]
              tunnel: w298 -> [w307 w315 _]
              frame "Post" {
                n102 = case shown="True" w307 {
                  tunnel: ["Wait" w312] -> w309
                  tunnel: w308 -> [_ w311]
                  frame False {
                    # "Writting Measurement Data is Disabled."
                  }
                  frame True {
                    # "Writting Measurement Data is Enabled."
                    n103 = case shown="\"ErrorInWriting\"" w311 {
                      tunnel: ["SaveMeasurementInfo" "Wait"] -> w312
                      frame "ErrorInWriting" {
                      }
                      frame "NoErrorInWriting", Default {
                      }
                    }
                  }
                }
              }
              frame "Save" {
                n104 = case shown="True" w315 {
                  tunnel: ["Wait" "SaveMeasurementInfo"] -> w316
                  frame False {
                    # "Writting Measurement Data is Disabled."
                  }
                  frame True {
                    # "Writting Measurement Data is Enabled."
                  }
                }
              }
              frame "Stop Post", Default {
              }
            }
            n105 = call <vilib>:"Add State(s) to Queue__JKI_lib_State_Machine.vi"("State(s) in Front (\"\")"=w301, "State(s) in (\"\")"=w305) -> ("States Out"=w306:string)  [unwired: 13 in]
          }
          event User Event {
            n106 = event-data() -> ()  [unwired: 1 in, 1 out]
            n107 = call <vilib>:"Add State(s) to Queue__JKI_lib_State_Machine.vi"("State(s) in Front (\"\")"="Macro: Exit", "State(s) in (\"\")"=w323) -> ("States Out"=w324:string)  [unwired: 13 in]
          }
        }
      }
      frame "---------- Core ----------" {
        # "Do not put any code in this frame.\n(it is a separator no-op)"
        n108 = call <vilib>:"Add State(s) to Queue__JKI_lib_State_Machine.vi"("State(s) in (\"\")"=w328) -> ("States Out"=w327:string)  [unwired: 14 in]
      }
      frame Default {
        w338 = 42 items=["No error", "Argument error", "Memory is full", "Out of zone", "End of file", "File already open", "Generic file I/O error", "File not found", "File permission error", "Disk is full", "Duplicate path", "Too many files open", "System feature not enabled", "Resource file not found", "Cannot add resource", "Resource not found", "Image not found", "Image memory error", "Pen does not exist", "Config type invalid", "Config token not found", "Config parse error", "Config memory error", "Bad external code format", "Bad external code offset", "External code not present", "Null window", "Destroy window error", "Null menu", "Print aborted", "Bad print record", "Print driver error", "Windows error during printing", "Memory error during printing", "Print dialog error", "Generic print error", "Invalid device refnum", "Device not found", "Device parameter error", "Device unit error", "Cannot open device", "Device call aborted", "Generic error", "Cancelled by user", "Object ID too low", "Object ID too high", "Object not in heap", "Unknown heap", "Unknown object (invalid DefProc)", "Unknown object (DefProc not in table)", "Message out of range", "Invalid (null) method", "Unknown message", "Manager call not supported", "Bad address", "Network operation in progress", "Network operation timed out", "Connection is busy", "Network attribute not supported", "Network error", "Address in use", "System out of memory", "Connection aborted", "Connection refused", "Not connected", "Already connected", "Connection closed", "Initialization error (interapplication manager)", "Bad occurrence", "Wait on unbound occurrence handler", "Occurrence queue overflow", "Datalog type conflict", "Unused", "Unrecognized type (interapplication manager)", "Memory corrupt", "Failed to make temporary DLL", "Old CIN version", "Drag socket not found", "Failed to load drop-object", "Failed to register OLE object", "Failed to release OLE object", "Format specifier type mismatch", "Unknown format specifier", "Too few format specifiers", "Too many format specifiers", "Scan failed", "Newer CIN version", "Error converting to variant", "Runtime menu error", "Password tampered", "Variant attribute not found", "Incompatible variant data type", "Event data is not available", "Event Store is not present", "Occurrence is not found", "Event Queue is not created", "Event info is not available", "Refnum passed is NULL", "Error retrieving Class GUID", "Error retrieving CoClass GUID", "Error retrieving TypeLib GUID.", "Bad built application magic bytes.", "Specific driver is different from the specific driver associated with the Logical Name.", "There is no session opened to the class driver.", "Max Error", "MAX - Error with config objects", "MAX - Error loading configuration", "MAX - Group not supported"]
        # "Current State"
        # "Do not delete, rename, or modify this frame.\n(this is used to capture unhandled states and typos)"
        # "Handle mistyped state name (developer tool)"
        n109 = Format Into String(format string="Software Exception: Unhandled State \"%s\"." ("message"), error in=w334, w329) -> (resulting string=w337:string, error out=w336:errorcluster)  [unwired: 1 in]
        n110 = call <vilib>:"Error Cluster From Error Code.vi"("show call chain? (False)"=TRUE, "error in (no error)"=w336, "error message (\"\")"=w337, "error code (0)"=w338) -> ("error out"=w335:errorcluster)  [unwired: 5 in]
        n111 = call <vilib>:"Add State(s) to Queue__JKI_lib_State_Machine.vi"("State(s) in (\"\")"=w333) -> ("States Out"=w332:string)  [unwired: 14 in]
      }
      frame "Initialize Core Data" {
        # "Do not delete, rename, or modify this frame.\n(this is used to determine panel behavior on exit)"
        # "originally closed?"
        # "exe?"
        # "If panel starts closed or is an EXE, then close it when we exit"
        n112 = property class="VI"() -> ("Front Panel.Open"=w347:bool)  [unwired: 2 in, 2 out]
        n113 = property class="App"() -> ("App.Kind"=w346:T4)  [unwired: 2 in, 2 out]
        n114 = control-ref of="Current VI Reference"() -> (w340:refnum<vi>)
        n115 = Not(x=w347) -> (.not. x?=w344:bool)
        n116 = Equal?(x=w346, y=T4."Run Time System" ("Application:Kind")) -> (x = y?=w343:bool)
        n117 = Or(x=w344, y=w343) -> (x .or. y?=w341:bool)
        n118 = Bundle By Name(cluster=w342, "Core.Current VI Reference"=w340, "Core.Close Panel on Exit?"=w341) -> (w349:T2)
        n119 = call <vilib>:"Add State(s) to Queue__JKI_lib_State_Machine.vi"("State(s) in (\"\")"=w351) -> ("States Out"=w350:string)  [unwired: 14 in]
      }
      frame "Error Handler" {
        # "Handle any errors here.\nYou can also output any states to clean-up after errors occur"
        # "Clear error"
        n120 = call <vilib>:"Add State(s) to Queue__JKI_lib_State_Machine.vi"("State(s) in Front (\"\")"="/* Post Error States", "State(s) in (\"\")"=w356) -> ("States Out"=w355:string)  [unwired: 13 in]
      }
      frame "Exit" {
        n121 = call <vilib>:"Add State(s) to Queue__JKI_lib_State_Machine.vi"("State(s) in (\"\")"=w361) -> ("States Out"=w360:string)  [unwired: 14 in]
      }
      frame "---------- Data ----------" {
        # "Do not put any code in this frame.\n(It is a separator no-op. You can make a copy of this frame to create a new Data frame)"
        n122 = call <vilib>:"Add State(s) to Queue__JKI_lib_State_Machine.vi"("State(s) in (\"\")"=w365) -> ("States Out"=w364:string)  [unwired: 14 in]
      }
      frame "Data: Initialize" {
        w366 = FALSE  # StripPath
        w367 = 0  # ReelCounterPerPart
        w368 = 1  # ExcelSheetCounterPerReel
        w369 = 0  # RecordsInExcelCounter
        w370 = FALSE  # WriteMeasurementData
        w372 = T6 {"Current VI Reference"=refnum, "Close Panel on Exit?"=FALSE}  # Core
        # "StripPath :\nThis boolean tells us whether a path is already built or not.\nIt can either be true or false\nTrue: A portion of the already built path has to be stripped to make the new current path.\nFalse: No path is existing.So no part of the path has to be stripped to make the new current path."
        # "Counts the no of reel inspected per part\nGets reinitialized to 0 on part details when initialize is true."
        # "Counts the no of sheets created for one reel"
        # "Counts the no of records that are there in one excel"
        # "Tells whether Measurement data to be logged or not"
        # "Initialize the shift-register data, here.\n(data names are defined by what you wire into the bundle function)"
        n123 = call <vilib>:"Add State(s) to Queue__JKI_lib_State_Machine.vi"("State(s) in (\"\")"=w376) -> ("States Out"=w375:string)  [unwired: 14 in]
        n124 = Bundle By Name(cluster="Cluster", "Core"=w372, "WriteMeasurementData"=w370, "RecordsInExcelCounter"=w369, "ExcelSheetCounterPerReel"=w368, "ReelCounterPerPart"=w367, "StripPath"=w366) -> (w371:T2)
      }
      frame "Data: Cleanup" {
        # "Cleanup any data and references, here.\n(this is called automatically, by the Macro: Exit)"
        n125 = Unbundle By Name(w402) -> ("Core.Current VI Reference"=w404:refnum<vi>)
        n126 = Close Reference(reference=w404, error in (no error)=w403) -> (error out=w387:errorcluster)
        n127 = Unbundle By Name(w386) -> ("MasterSampleInfo"=w377:refnum<user-event>, "MeasurementInfo"=w383:refnum<user-event>, "PartDetails"=w382:refnum<user-event>, "Stop"=w399:refnum<user-event>, "State Message"=w398:refnum<user-event>, "MachineStatus"=w397:refnum<user-event>, "AllPartInitialization"=w396:refnum<user-event>, "BatchID"=w395:refnum<user-event>, "LogMeasurementData"=w394:refnum<user-event>)
        n128 = Flush Event Queue(0:w385, 3:w387) -> (8:w400:refnum<event-registration>, 11:w401:errorcluster)  [unwired: 4 in, 1 out]
        n129 = call <vilib>:"Add State(s) to Queue__JKI_lib_State_Machine.vi"("State(s) in (\"\")"=w406) -> ("States Out"=w405:string)  [unwired: 14 in]
        n130 = Unregister For Events(event registration refnum=w400, error in=w401) -> (error out=w378:errorcluster)
        n131 = Destroy User Event(user event=w377, error in=w378) -> (error out=w379:errorcluster)
        n132 = Destroy User Event(user event=w383, error in=w378) -> (error out=w381:errorcluster)
        n133 = Destroy User Event(user event=w382, error in=w378) -> (error out=w380:errorcluster)
        n134 = Destroy User Event(user event=w399, error in=w378) -> (error out=w393:errorcluster)
        n135 = Destroy User Event(user event=w398, error in=w378) -> (error out=w392:errorcluster)
        n136 = Destroy User Event(user event=w397, error in=w378) -> (error out=w391:errorcluster)
        n137 = Destroy User Event(user event=w396, error in=w378) -> (error out=w390:errorcluster)
        n138 = Destroy User Event(user event=w395, error in=w378) -> (error out=w389:errorcluster)
        n139 = Destroy User Event(user event=w394, error in=w378) -> (error out=w388:errorcluster)
        n140 = Merge Errors(w379, w381, w380, w393, w392, w391, w390, w389, w388) -> (w384:errorcluster)
      }
      frame "---------- UI ----------" {
        # "Do not put any code in this frame.\n(It is a separator no-op. You can make a copy of this frame to create a new UI frame)"
        n141 = call <vilib>:"Add State(s) to Queue__JKI_lib_State_Machine.vi"("State(s) in (\"\")"=w410) -> ("States Out"=w409:string)  [unwired: 14 in]
      }
      frame "UI: Initialize" {
        # "Initialize the User Interface, here.\n(this is called automatically, by the Macro: Init)"
        n142 = call <vilib>:"Add State(s) to Queue__JKI_lib_State_Machine.vi"("State(s) in (\"\")"=w414) -> ("States Out"=w413:string)  [unwired: 14 in]
      }
      frame "UI: Cursor Set" {
        # "Argument"
        # "Set and Unset Cursor Busy.\n(Usage: \"UI: Cursor Set >> Busy|Idle\")"
        n143 = case shown="\"Idle\", Default" w415 {
          tunnel: w417 -> [w422 w424]
          tunnel: [w421 w423] -> w416
          frame "Idle", Default {
            n144 = call <vilib>:"Unset Busy.vi"("error in (no error)"=w422) -> ("error out"=w421:errorcluster)  [unwired: 10 in]
          }
          frame "Busy" {
            n145 = call <vilib>:"Set Busy.vi"("error in (no error)"=w424) -> ("error out"=w423:errorcluster)  [unwired: 9 in, 1 out]
          }
        }
        n146 = call <vilib>:"Add State(s) to Queue__JKI_lib_State_Machine.vi"("State(s) in (\"\")"=w420) -> ("States Out"=w419:string)  [unwired: 14 in]
      }
      frame "UI: Front Panel State" {
        # "Argument"
        # "Set Front Panel Open or Closed\n(Usage: \"UI: Front Panel State >> Open|Close\")"
        n147 = Unbundle By Name(w427) -> ("Core.Current VI Reference"=w426:refnum<vi>)
        n148 = case shown="\"Open\", Default" w425 {
          tunnel: w429 -> [w435 w448]
          tunnel: [w437 w449] -> w428
          tunnel: w426 -> [w436 w446]
          frame "Open", Default {
            n149 = property class="VI"(reference=w436, error in=w435) -> (reference out=w433:refnum<vi>, error out=w434:errorcluster, "Front Panel.Open"=w432:bool)
            n150 = case shown="False" w432 {
              tunnel: [w440 w443] -> w437
              tunnel: w434 -> [w439 w443]
              tunnel: w433 -> [w438 _]
              frame False {
                n151 = invoke class="VI" method="FP.Open"(reference=w438, error in=w439, "Activate"=TRUE, "State"=T5."Standard") -> (error out=w440:errorcluster)  [unwired: 1 in, 4 out]
              }
              frame True {
              }
            }
          }
          frame "Close" {
            n152 = property class="VI"(reference=w446, error in=w448) -> (reference out=w445:refnum<vi>, error out=w447:errorcluster, "Front Panel.Open"=w444:bool)
            n153 = case shown="True" w444 {
              tunnel: [w450 w453] -> w449
              tunnel: w447 -> [w450 w452]
              tunnel: w445 -> [_ w451]
              frame False {
              }
              frame True {
                n154 = invoke class="VI" method="FP.Close"(reference=w451, error in=w452) -> (error out=w453:errorcluster)  [unwired: 1 in, 2 out]
              }
            }
          }
        }
        n155 = call <vilib>:"Add State(s) to Queue__JKI_lib_State_Machine.vi"("State(s) in (\"\")"=w431) -> ("States Out"=w430:string)  [unwired: 14 in]
      }
      frame "---------- Macro ----------" {
        # "Do not put any code in this frame.\n(It is a separator no-op. You can make a copy of this frame to create a new Macro frame)"
        n156 = call <vilib>:"Add State(s) to Queue__JKI_lib_State_Machine.vi"("State(s) in (\"\")"=w457) -> ("States Out"=w456:string)  [unwired: 14 in]
      }
      frame "Macro: Initialize" {
        # "Initialization Macro\n(This is called once, when the VI starts)"
        n157 = call <vilib>:"Add State(s) to Queue__JKI_lib_State_Machine.vi"("State(s) in Front (\"\")"="Data: Initialize\nInitialize Core Data\nUI: Initialize", "State(s) in (\"\")"=w462) -> ("States Out"=w461:string)  [unwired: 13 in]
      }
      frame "Macro: Exit" {
        # "Exit Macro\n(This is called once, when the VI exits)"
        n158 = call <vilib>:"Add State(s) to Queue__JKI_lib_State_Machine.vi"("State(s) in Front (\"\")"="Data: Cleanup\nExit", "State(s) in (\"\")"=w467) -> ("States Out"=w466:string)  [unwired: 13 in]
      }
      frame "---------- Master Sample----------" {
        # "Template Separator\n(You can make a copy of, or modify, this frame)"
        n159 = call <vilib>:"Add State(s) to Queue__JKI_lib_State_Machine.vi"("State(s) in (\"\")"=w471) -> ("States Out"=w470:string)  [unwired: 14 in]
      }
      frame "MasterSampleFolderCreation" {
        n160 = Unbundle By Name(w487) -> ("MasterSampleExcelPath"=w484:path)
        n161 = Unbundle By Name(w479) -> ("MasterSampleInfo.NumberOfMeasurements"=w472:i32, "AllPartInfoArray"=w480:T3)
        n162 = Strip Path(path=w484) -> (stripped path=w483:path)  [unwired: 1 out]
        n163 = call <vilib>:"Check if File or Folder Exists.vi"("error in (no error)"=w482, "path"=w483) -> ("error out"=w492:errorcluster, "file or folder exists?"=w494:bool, "dup path"=w493:path)  [unwired: 7 in]
        n164 = case shown="False" w494 {
          tunnel: w493 -> [_ w507]
          tunnel: [w504 w506] -> w491
          tunnel: w492 -> [w504 w505]
          frame True {
          }
          frame False {
            n165 = Create Folder(path (use dialog)=w507, error in=w505) -> (error out=w506:errorcluster)  [unwired: 1 in, 2 out]
          }
        }
        n166 = call "ExcelLabelCreation.vi"("NumberOfMeasurements"=w472, "AllPartInfoArray"=w480, "TableName"="MasterSample") -> ("Labels"=w486:string[][])  [unwired: 7 in, 1 out]
        n167 = call <vilib>:"Check if File or Folder Exists.vi"("error in (no error)"=w491, "path"=w484) -> ("error out"=w489:errorcluster, "file or folder exists?"=w488:bool, "dup path"=w490:path)  [unwired: 7 in]
        n168 = case shown="False" w488 {
          tunnel: [w501 w503] -> w481
          tunnel: w489 -> [w500 w503]
          tunnel: w490 -> [w499 _]
          tunnel: w486 -> [w497 _]
          frame False {
            n169 = call-poly <vilib>:"Write Delimited Spreadsheet.vi"("file path (dialog if empty)"=w499, "2D data"=w497, "append to file? (new file:F)"=TRUE ("append to file? (F)"), "error in (no error)"=w500, "delimiter (\\t)"=",\t" ("delimiter (\\t)")) -> ("error out"=w501:errorcluster)  [unwired: 9 in, 1 out]
          }
          frame True {
          }
        }
        n170 = Add(x=w472, y=4) -> (x+y=w475:i32)
        n171 = Initialize Array("", 10 ("dimension size"), w475) -> (w473:string[][])
        n172 = Bundle By Name(cluster=w479, "MasterSampleDetails.Array(2D)"=w473) -> (w478:T2)
        n173 = call <vilib>:"Add State(s) to Queue__JKI_lib_State_Machine.vi"("State(s) in (\"\")"=w496) -> ("States Out"=w495:string)  [unwired: 14 in]
      }
      frame "MastersampleInfo" {
        n174 = in-place {
          n175 = in-place-cluster #1(w512) -> ("MasterSampleInfo.MSPartName"=w514:string, "MasterSampleInfo.MSDate"=w515:string, "MasterSampleInfo.MSTime"=w516:string, "MasterSampleInfo.MSMeasurementValueArray"=w517:dbl[], "MasterSampleInfo.MSResult"=w518:string, "MasterSampleDetails.IndexCounter"=w520:i32, "MasterSampleDetails.Array(2D)"=w522:string[][])
          n176 = Replace Array Subset(array=w522, new element #1=w514, index (row) #1=w520, index (col) #1=0 ("index (col)"), new element #2=w515, index (row) #2=w520, index (col) #2=1 ("index (col)"), new element #3=w516, index (row) #3=w520, index (col) #3=2 ("index (col)")) -> (w526:string[][])
          n177 = for {
            shift-right: [w534] -> w524
            shift-left: w526 -> [w537]
            shift-right: [w536] -> w523
            shift-left: 3 ("index (col)") -> [w535]
            tunnel: w517 -> [w530] mode=indexing
            tunnel: w520 -> [w531]
            n178 = Increment(x=w535) -> (x+1=w536:i32)
            n179 = Number To Fractional String(number=w530, precision (6)=3 ("disabled index (col)")) -> (F-format string=w533:string)  [unwired: 2 in]
            n180 = Replace Array Subset(array=w537, new element=w533, index (row)=w531, index (col)=w535) -> (w534:string[][])
          }
          n181 = Replace Array Subset(array=w524, new element=w518, index (row)=w520, index (col)=w523) -> (w519:string[][])
          n182 = Increment(x=w520) -> (x+1=w521:i32)
          n183 = in-place-cluster #1("MasterSampleInfo.MSPartName"=w514, "MasterSampleInfo.MSDate"=w515, "MasterSampleInfo.MSTime"=w516, "MasterSampleInfo.MSMeasurementValueArray"=w517, "MasterSampleInfo.MSResult"=w518, "MasterSampleDetails.IndexCounter"=w521, "MasterSampleDetails.Array(2D)"=w519) -> (w511:T2)
        }
        n184 = call <vilib>:"Add State(s) to Queue__JKI_lib_State_Machine.vi"("State(s) in Front (\"\")"="SaveMasterSampleInfo" ("State(s) in Front (\"\")"), "State(s) in (\"\")"=w510) -> ("States Out"=w513:string)  [unwired: 13 in]
      }
      frame "SaveMasterSampleInfo" {
        n185 = Unbundle By Name(w542) -> ("MasterSampleExcelPath"=w541:path)
        n186 = Unbundle By Name(w540) -> ("MasterSampleDetails.Array(2D)"=w545:string[][], "MasterSampleDetails.IndexCounter"=w544:i32)  [unwired: 1 out]
        n187 = Array Subset(array=w545, index (row)=0 ("index"), length (row)=w544) -> (w543:string[][])  [unwired: 2 in]
        n188 = call-poly <vilib>:"Write Delimited Spreadsheet.vi"("file path (dialog if empty)"=w541, "2D data"=w543, "append to file? (new file:F)"=TRUE ("append to file? (F)"), "delimiter (\\t)"="," ("delimiter (\\t)")) -> ()  [unwired: 10 in, 2 out]
        n189 = Bundle By Name(cluster=w540, "MasterSampleDetails.IndexCounter"=0) -> (w539:T2)
        n190 = call <vilib>:"Add State(s) to Queue__JKI_lib_State_Machine.vi"("State(s) in (\"\")"=w551) -> ("States Out"=w550:string)  [unwired: 14 in]
      }
      frame "----------All Measurement----------" {
        n191 = call <vilib>:"Add State(s) to Queue__JKI_lib_State_Machine.vi"("State(s) in (\"\")"=w555) -> ("States Out"=w554:string)  [unwired: 14 in]
      }
      frame "ExcelFolderCreation" {
        # "Reinitialized to 0"
        # "Strip path is made true implies that now a path exists.Now if a new path is to be \nbuilt,some portion of the already existing file path has to be stripped."
        # "File path for excel inside folders"
        n192 = Unbundle By Name(w580) -> ("PartDetails.NumberOfMeasurements"=w556:i32, "AllPartInfoArray"=w558:T3, "PartDetails.PartName"=w557:string, "StripPath"=w565:bool, "MeasurementExcelPath"=w564:path, "ExcelSheetCounterPerReel"=w577:i32)
        n193 = case shown="True" w565 {
          tunnel: w564 -> [w593 w595]
          tunnel: [w593 w594] -> w563
          frame False {
          }
          frame True {
            n194 = Strip Path(path=w595) -> (stripped path=w594:path)  [unwired: 1 out]
          }
        }
        n195 = call "ExcelLabelCreation.vi"("NumberOfMeasurements"=w556, "Part Name"=w557, "AllPartInfoArray"=w558, "TableName"="Measurement") -> ("Labels"=w560:string[][])  [unwired: 6 in, 1 out]
        n196 = Increment(x=w577) -> (x+1=w576:i32)
        n197 = call <vilib>:"Check if File or Folder Exists.vi"("error in (no error)"=w588, "path"=w563) -> ("error out"=w587:errorcluster, "file or folder exists?"=w590:bool, "dup path"=w589:path)  [unwired: 7 in]
        n198 = Strip Path(path=w563) -> (stripped path=w585:path, name=w582:string)
        n199 = case shown="False" w590 {
          tunnel: w589 -> [_ w608]
          tunnel: [w605 w607] -> w574
          tunnel: w587 -> [w605 w606]
          frame True {
          }
          frame False {
            n200 = Create Folder(path (use dialog)=w608, error in=w606) -> (error out=w607:errorcluster)  [unwired: 1 in, 2 out]
          }
        }
        n201 = Strip Path(path=w585) -> (stripped path=w586:path, name=w583:string)
        n202 = Number To Decimal String(number=w576) -> (decimal integer string=w578:string)  [unwired: 1 in]
        n203 = Strip Path(path=w586) -> (name=w584:string)  [unwired: 1 out]
        n204 = call <vilib>:"Space Constant.vi"() -> ("String"=w561:string)
        n205 = Concatenate Strings(w584, w561, w583, w561, w582, w561, "(Sheet " ("string"), w578, ").csv" ("string")) -> (w573:string)
        n206 = Build Path(base path=w563, name or relative path=w573) -> (appended path=w572:path)
        n207 = call <vilib>:"Check if File or Folder Exists.vi"("error in (no error)"=w574, "path"=w572) -> ("error out"=w570:errorcluster, "file or folder exists?"=w569:bool, "dup path"=w571:path)  [unwired: 7 in]
        n208 = case shown="False" w569 {
          tunnel: [w601 w604] -> w568
          tunnel: w570 -> [w600 w604]
          tunnel: w571 -> [w599 w603]
          tunnel: [w597 w603] -> w567
          tunnel: w560 -> [w596 _]
          frame False {
            n209 = call-poly <vilib>:"Write Delimited Spreadsheet.vi"("file path (dialog if empty)"=w599, "2D data"=w596, "append to file? (new file:F)"=TRUE ("append to file? (F)"), "error in (no error)"=w600, "delimiter (\\t)"=",\t" ("delimiter (\\t)")) -> ("new file path (Not A Path if cancelled)"=w597:path, "error out"=w601:errorcluster)  [unwired: 9 in]
          }
          frame True {
          }
        }
        n210 = Bundle By Name(cluster=w580, "StripPath"=TRUE, "MeasurementExcelPath"=w567, "ExcelSheetCounterPerReel"=w576, "RecordsInExcelCounter"=0) -> (w579:T2)
        n211 = call <vilib>:"Add State(s) to Queue__JKI_lib_State_Machine.vi"("State(s) in (\"\")"=w592) -> ("States Out"=w591:string)  [unwired: 14 in]
      }
      frame "InitializeMeasurementInfoArray" {
        n212 = Unbundle By Name(w614) -> ("PartDetails.NumberOfMeasurements"=w613:i32)
        n213 = Add(x=w613, y=6) -> (x+y=w612:i32)
        n214 = Initialize Array("", 1000 ("dimension size"), w612) -> (w610:string[][])
        n215 = Bundle By Name(cluster=w614, "MeasurementDetails.Array(2D)"=w610) -> (w617:T2)
        n216 = call <vilib>:"Add State(s) to Queue__JKI_lib_State_Machine.vi"("State(s) in Front (\"\")"="Wait" ("State(s) in Front (\"\")"), "State(s) in (\"\")"=w620) -> ("States Out"=w619:string)  [unwired: 13 in]
      }
      frame "MeasurementInfo" {
        n217 = in-place {
          n218 = in-place-cluster #2(w633) -> ("PartDetails.PartName"=w658:string, "BatchID"=w656:string, "PartDetails.OperatorName"=w655:string, "MeasurementInfo.MeasurementDate"=w653:string, "MeasurementInfo.MeasurementTime"=w650:string, "PartDetails.MeasurementEnable/DisableArray"=w647:bool[], "MeasurementInfo.MeasurementValueArray"=w645:dbl[], "MeasurementInfo.MeasurementResult"=w639:string, "RecordsInExcelCounter"=w638:i32, "MeasurementDetails.IndexCounter"=w641:i32, "MeasurementDetails.Array(2D)"=w659:string[][])
          n219 = Replace Array Subset(array=w659, new element #1=w658, index (row) #1=w641, index (col) #1=0 ("index (col)"), new element #2=w656, index (row) #2=w641, index (col) #2=1 ("index (col)"), new element #3=w655, index (row) #3=w641, index (col) #3=2 ("index (col)"), new element #4=w653, index (row) #4=w641, index (col) #4=3 ("index (col)"), new element #5=w650, index (row) #5=w641, index (col) #5=4 ("index (col)")) -> (w649:string[][])
          n220 = for {
            shift-right: [w666] -> w644
            shift-left: w649 -> [w670]
            tunnel: w641 -> [w669]
            shift-right: [w668] -> w640
            shift-left: 5 ("index (col)") -> [w667]
            tunnel: w647 -> [w665] mode=indexing
            shift-right: [w662] -> _
            shift-left: 0 ("index (col)") -> [w664]
            tunnel: w645 -> [w663]
            n221 = case shown="True" w665 {
              tunnel: w664 -> [w672 w677]
              tunnel: w663 -> [_ w678]
              tunnel: [w672 w676] -> w662
              tunnel: ["Disabled" w673] -> w661
              frame False {
              }
              frame True {
                n222 = Index Array(array=w678, index=w677) -> (element=w675:dbl)
                n223 = Increment(x=w677) -> (x+1=w676:i32)
                n224 = Number To Fractional String(number=w675, precision (6)=3 ("disabled index (col)")) -> (F-format string=w673:string)  [unwired: 2 in]
              }
            }
            n225 = Increment(x=w667) -> (x+1=w668:i32)
            n226 = Replace Array Subset(array=w670, new element=w661, index (row)=w669, index (col)=w667) -> (w666:string[][])
          }
          n227 = Increment(x=w638) -> (x+1=w637:i32)
          n228 = Replace Array Subset(array=w644, new element=w639, index (row)=w641, index (col)=w640) -> (w643:string[][])
          n229 = Increment(x=w641) -> (x+1=w642:i32)
          n230 = in-place-cluster #2("PartDetails.PartName"=w658, "BatchID"=w656, "PartDetails.OperatorName"=w655, "MeasurementInfo.MeasurementDate"=w653, "MeasurementInfo.MeasurementTime"=w650, "PartDetails.MeasurementEnable/DisableArray"=w647, "MeasurementInfo.MeasurementValueArray"=w645, "MeasurementInfo.MeasurementResult"=w639, "RecordsInExcelCounter"=w637, "MeasurementDetails.IndexCounter"=w642, "MeasurementDetails.Array(2D)"=w643) -> (w632:T2)
        }
        n231 = Unbundle By Name(w632) -> ("RecordsInExcelCounter"=w625:i32, "MeasurementDetails.IndexCounter"=w631:i32)
        n232 = Equal?(x=w631, y=100) -> (x = y?=w629:bool)
        n233 = Less?(x=w625, y=10001) -> (x < y?=w623:bool)
        n234 = Select(t="SaveMeasurementInfo", s=w623, f="ExcelFolderCreation\nSaveMeasurementInfo") -> (s? t:f=w626:string)
        n235 = Select(t=w626, s=w629, f="Wait") -> (s? t:f=w628:string)
        n236 = call <vilib>:"Add State(s) to Queue__JKI_lib_State_Machine.vi"("State(s) in Front (\"\")"=w628, "State(s) in (\"\")"=w636) -> ("States Out"=w635:string)  [unwired: 13 in]
      }
      frame "SaveMeasurementInfo" {
        n237 = Unbundle By Name(w688) -> ("MeasurementExcelPath"=w679:path, "StateMessage"=w680:string, "MachineStatus"=w685:string, "MeasurementDetails.Array(2D)"=w691:string[][], "MeasurementDetails.IndexCounter"=w690:i32, "WriteMeasurementData"=w692:bool)
        n238 = case shown="True" w692 {
          tunnel: w691 -> [_ w709]
          tunnel: w690 -> [_ w699]
          tunnel: [0 ("IndexCounter") w708] -> w687
          tunnel: ["NoErrorInWriting" w707] -> w686
          tunnel: w685 -> [_ w706]
          tunnel: w684 -> [w695 w705]
          tunnel: w683 -> [_ w704]
          tunnel: [w695 w703] -> w682
          tunnel: w680 -> [_ w702]
          tunnel: w679 -> [_ w701]
          frame False {
            # "Don't Write Measurement Data"
          }
          frame True {
            # "Write Measurement Data"
            n239 = Equal?(x=w699, y=0) -> (x = y?=w700:bool)
            n240 = case shown="False" w700 {
              tunnel: w709 -> [w722 _]
              tunnel: w699 -> [w720 _]
              tunnel: [w719 0 ("IndexCounter")] -> w708
              tunnel: [w718 "NoErrorInWriting"] -> w707
              tunnel: w706 -> [w717 _]
              tunnel: w705 -> [w716 w764]
              tunnel: w704 -> [w715 w765]
              tunnel: [w714 w763] -> w703
              tunnel: w702 -> [w713 w766]
              tunnel: w701 -> [w712 _]
              frame False {
                # "Data available for writting"
                n241 = Array Subset(array=w722, index (row)=0 ("index"), length (row)=w720) -> (w723:string[][])  [unwired: 2 in]
                n242 = call-poly <vilib>:"Write Delimited Spreadsheet.vi"("file path (dialog if empty)"=w712, "2D data"=w723, "append to file? (new file:F)"=TRUE ("append to file? (F)"), "error in (no error)"=w716, "delimiter (\\t)"="," ("delimiter (\\t)")) -> ("error out"=w721:errorcluster)  [unwired: 9 in, 1 out]
                n243 = case shown="No Error" w721 {
                  selector: w721 -> [w726 _]
                  tunnel: [0 ("IndexCounter") w741] -> w719
                  tunnel: w720 -> [_ w741]
                  tunnel: ["NoErrorInWriting" "ErrorInWriting"] -> w718
                  tunnel: w717 -> [_ w739]
                  tunnel: w715 -> [w727 w738]
                  tunnel: [w725 w737] -> w714
                  tunnel: w713 -> [w728 _]
                  frame No Error {
                    n244 = case shown="\"Save\"" w728 {
                      tunnel: w727 -> [_ w735]
                      tunnel: w726 -> [w731 w734]
                      tunnel: [w731 w733] -> w725
                      frame Default {
                      }
                      frame "Save" {
                        n245 = Unbundle By Name(w735) -> ("SaveAckFromMeas.Loop"=w736:refnum<user-event>)
                        n246 = Generate User Event(user event=w736, event data cluster=TRUE ("event data"), error in=w734) -> (error out=w733:errorcluster)  [unwired: 1 in, 1 out]
                      }
                    }
                  }
                  frame Error {
                    n247 = case shown="Default" w739 {
                      tunnel: w738 -> [w746 w761]
                      tunnel: [w747 w759] -> w737
                      frame "Inspection" {
                        n248 = flat-sequence {
                          tunnel: [w751] -> w745
                          tunnel: w746 -> [w751]
                          tunnel: [w750] -> w743
                          tunnel: w745 -> [w754]
                          tunnel: [w754] -> w744
                          tunnel: w743 -> [w753]
                          tunnel: [w753] -> w742
                          tunnel: [w757] -> w747
                          tunnel: w744 -> [w756]
                          tunnel: w742 -> [w755]
                          frame #0 {
                            n249 = call "Output_DL.vi"("Private Data"=w751, "error in (no error)"=errorcluster {"status"=FALSE, "code"=0, "source"=""}, "State"="Pause") -> ("error out"=w750:errorcluster)  [unwired: 8 in]
                          }
                          frame #1 {
                            n250 = Wait (ms)(milliseconds to wait=u32 100) -> ()  [unwired: 1 out]
                          }
                          frame #2 {
                            n251 = call "Output_DL.vi"("Private Data"=w756, "error in (no error)"=w755, "State"="ErrorPopUp") -> ("error out"=w757:errorcluster)  [unwired: 8 in]
                          }
                        }
                      }
                      frame Default {
                        n252 = call "Output_DL.vi"("Private Data"=w761, "error in (no error)"=errorcluster {"status"=FALSE, "code"=0, "source"=""}, "State"="ErrorPopUp") -> ("error out"=w759:errorcluster)  [unwired: 8 in]
                      }
                    }
                  }
                }
              }
              frame True {
                # "No data available to write"
                n253 = case shown="\"Save\"" w766 {
                  tunnel: w765 -> [_ w773]
                  tunnel: w764 -> [w769 w772]
                  tunnel: [w769 w771] -> w763
                  frame Default {
                  }
                  frame "Save" {
                    n254 = Unbundle By Name(w773) -> ("SaveAckFromMeas.Loop"=w774:refnum<user-event>)
                    n255 = Generate User Event(user event=w774, event data cluster=TRUE ("event data"), error in=w772) -> (error out=w771:errorcluster)  [unwired: 1 in, 1 out]
                  }
                }
              }
            }
          }
        }
        n256 = Bundle By Name(cluster=w688, "CurrentState"=w686, "MeasurementDetails.IndexCounter"=w687) -> (w689:T2)
        n257 = call <vilib>:"Add State(s) to Queue__JKI_lib_State_Machine.vi"("State(s) in Front (\"\")"="Wait", "State(s) in (\"\")"=w694) -> ("States Out"=w693:string)  [unwired: 13 in]
      }
    }
  }
  n258 = while "JKI - String-Based Queued State Machine (Basic) v1.0" {
    shift-right: [w775] -> _
    shift-left: _ -> [w780]
    shift-right: [w776] -> w16
    shift-left: w17 -> [w779]
    shift-right: [w782] -> _
    shift-left: w37 -> [w783]
    tunnel: "DataLogger in" -> [w778]
    tunnel: w34 -> [w777]
    stop <- w781 stop-if-true
    # "IoT Loop"
    n259 = call <vilib>:"Parse State Queue__JKI_lib_State_Machine.vi"("State Queue"=w783, "Error In (no error)"=w779) -> ("Remaining States"=w785:string, "Current State"=w786:string, "Arguments"=w784:string)  [unwired: 11 in]
    n260 = case shown="\"InitializeAllPartInfo\"" w786 {
      selector: w786 -> [_ _ w1050 _ _ _ _ _ _ _ _ _ _ _ _ _ _ _ _ _ _ _ _ _ _ _ _ _ _ _ _]
      tunnel: w785 -> [w794 w1048 w1053 w1071 w1076 w1081 w1085 w1103 w1133 w1137 w1141 w1148 w1174 w1180 w1190 w1194 w1207 w1222 w1277 w1282 w1295 w1327 w1360 w1396 w1454 w1572 w1756 w1771 w1825 w1911 w1939]
      tunnel: w784 -> [_ _ _ _ _ _ _ _ _ _ _ w1142 _ _ _ _ _ _ _ w1289 _ _ _ _ _ _ _ _ _ _ _]
      tunnel: w780 -> [w792 w1045 w1049 w1063 w1072 w1077 w1082 _ w1130 w1134 w1138 w1144 w1171 w1175 w1187 w1191 w1205 w1214 w1225 w1287 w1292 w1318 w1358 w1394 w1452 w1570 w1754 w1769 w1814 w1906 w1924]
      tunnel: w779 -> [w790 w1046 w1054 w1069 _ w1079 w1083 w1101 w1131 w1135 w1139 w1146 w1172 w1178 w1188 w1192 w1201 w1219 w1226 w1285 w1294 w1321 w1340 w1395 w1453 w1571 w1734 w1770 w1827 w1909 w1936]
      tunnel: [w793 w1047 w1052 w1070 w1075 w1080 w1084 w1102 w1132 w1136 w1140 w1147 w1173 w1179 w1189 w1193 w1206 w1221 w1276 w1283 w1296 w1328 w1361 w1397 w1455 w1573 w1757 w1772 w1848 w1912 w1940] -> w782
      tunnel: [_ _ _ _ _ TRUE _ _ _ _ _ _ _ _ _ _ _ _ _ _ _ _ _ _ _ _ _ _ _ _ _] -> w781
      tunnel: w778 -> [w788 _ _ _ _ _ _ _ w1125 _ _ _ _ _ _ _ w1203 _ w1274 w1288 _ w1323 w1341 _ _ _ w1755 _ w1828 w1905 w1928]
      tunnel: w777 -> [w789 _ _ _ _ _ _ _ w1127 _ _ _ _ _ _ _ _ _ _ _ _ _ _ _ _ _ _ _ _ _ _]
      tunnel: [w791 w1046 w1055 w1069 errorcluster {"status"=FALSE, "code"=0, "source"=""} ("error out") w1079 w1083 w1101 w1108 w1135 w1139 w1145 w1172 w1178 w1188 w1192 w1200 w1219 w1244 w1284 w1291 w1319 w1339 w1395 w1453 w1571 w1735 w1770 w1815 w1908 w1929] -> w776
      tunnel: [w787 w1045 w1049 w1060 w1072 w1077 w1082 w1095 w1130 w1134 w1138 w1144 w1171 w1175 w1187 w1191 w1205 w1213 w1225 w1286 w1293 w1316 w1342 w1390 w1447 w1565 w1754 w1765 w1813 w1907 w1923] -> w775
      frame "", "Wait" {
        n261 = event shown="[3] <Reel Info>: User Event" {
          selector: w789 -> [_ _ _ _ _ _ _ _ _ w971 _ _ _]
          dyn-events: _ -> [_ _ _ _ _ _ _ _ _ _ _ _ _]
          timeout: _ -> [_ _ _ _ _ _ _ _ _ _ _ _ _]
          tunnel: w794 -> [w812 w831 w871 w903 w926 w939 w947 w954 w966 w978 w1018 w1022 w1042]
          tunnel: [w813 w830 w872 w904 w925 w940 w946 w955 w967 w979 w1019 w1024 w1043] -> w793
          tunnel: w792 -> [w816 w829 w870 w895 w921 w938 w945 w953 w964 w969 w1016 w1029 w1044]
          tunnel: [w795 w828 w875 w889 w928 w942 w949 w957 w958 w972 w1017 w1027 w1040] -> w791
          tunnel: w790 -> [w796 w828 w875 w890 w928 w942 w949 w957 w958 w973 w1017 w1026 w1040]
          tunnel: [w814 w825 w846 w888 w920 w934 w944 w950 w963 w970 w1016 w1028 w1044] -> w787
          tunnel: w788 -> [w798 _ _ w891 _ _ _ _ _ w974 _ w1025 _]
          event User Event {
            w804 = "_" ("string")
            # "Create new excel for only events boolean will be true.\nOther booleans will be false.\nIt is considered only  if IoT is disabled."
            # "Creates EventPath"
            # "Creating Inspection McID"
            # "Initialize System Info"
            n262 = event-data() -> ("Customer Details"=w815:T11, "Software Features"=w805:T12, "System Name"=w811:string, "Version"=w810:string, "Customer Details.Customer Name"=w809:string, "System ID"=w808:string, "Year"=w807:string, "Software Features.IoT Enable"=w803:bool, "Software Features.Datalogging Features.Measurement Data"=w797:bool)  [unwired: 1 in]
            n263 = disable-structure shown="Enabled" {
              disable-tunnel: w798 -> [w820 _]
              disable-tunnel: w797 -> [w819 _]
              disable-tunnel: w796 -> [w818 w822]
              disable-tunnel: [w817 w822] -> w795
              frame Disabled {
                n264 = Unbundle By Name(w820) -> ("LogMeasurementData"=w821:refnum<user-event>)
                n265 = Generate User Event(user event=w821, event data cluster=w819, error in=w818) -> (error out=w817:errorcluster)  [unwired: 1 in, 1 out]
              }
              frame Enabled {
              }
            }
            n266 = Concatenate Strings(w811, w804, w810, w804, w809, w804, w808, w804, w807) -> (w806:string)
            n267 = Select(t="DBTableCreation" ("State(s) in Front (\"\")"), s=w803, f="FilePathCreation>>EventPath\nExcelFolderCreation" ("State(s) in Front (\"\")")) -> (s? t:f=w801:string)
            n268 = Bundle By Name(cluster=w816, "System Info.Customer Details"=w815, "System Info.Software Features"=w805, "IDs.Inspection McID"=w806, "ExcelData.CreateNewExcel"=T7 {"CreateNewEventsExcel"=TRUE, "CreateNewFailExcel"=FALSE, "CreateNewStatisticalExcel"=FALSE, "CreateNewReelExcel"=FALSE}) -> (w814:T9)
            n269 = call <vilib>:"Add State(s) to Queue__JKI_lib_State_Machine.vi"("State(s) in Front (\"\")"=w801, "State(s) in (\"\")"=w812) -> ("States Out"=w813:string)  [unwired: 13 in]
          }
          event User Event {
            # "Removig master sample from AllPartInfo"
            # "All Part Initialization"
            n270 = event-data() -> ("AllPartInfoArray"=w824:T3)  [unwired: 1 in]
            n271 = for {
              tunnel: w824 -> [w833] mode=indexing
              tunnel: [w833] -> w823 mode=indexing if=w832
              n272 = Unbundle By Name(w833) -> ("PartName"=w835:string)
              n273 = Not Equal?(x=w835, y="Master Sample") -> (x != y?=w832:bool)
            }
            n274 = Bundle By Name(cluster=w829, "AllPartInfoArray"=w823) -> (w825:T9)
            n275 = Unbundle By Name(w825) -> ("System Info.Software Features.IoT Enable"=w827:bool)
            n276 = case shown="False" w827 {
              tunnel: ["Wait" ("State(s) in Front (\"\")") "InitializeAllPartInfo" ("State(s) in Front (\"\")")] -> w826
              frame False {
              }
              frame True {
              }
            }
            n277 = call <vilib>:"Add State(s) to Queue__JKI_lib_State_Machine.vi"("State(s) in Front (\"\")"=w826, "State(s) in (\"\")"=w831) -> ("States Out"=w830:string)  [unwired: 13 in]
          }
          event User Event {
            # "Strip path is made false as file is being built from starting"
            # "Reinitialize will be True during first time PartInfo.\nFrom next time onwards it will come as False(PartInfo sent during update)."
            # "Creating the StampingMcID"
            # "Initialize Part Info."
            n278 = event-data() -> ("StampingMc No"=w852:u64, "Part Name"=w874:string, "Reinitialize?"=w843:bool, "Operator Name"=w873:string, "TotalCount"=w861:u64, "ReelCount"=w848:u64, "Measurement Names Array"=w858:string[], "Measurement ID Array"=w859:u16[], "Spec Values Array"=w860:T13, "Camera Name Array"=w857:string[])  [unwired: 1 in]
            n279 = Unbundle By Name(w870) -> ("System Info.Software Features.IoT Enable"=w845:bool, "System Info.Customer Details.Customer Name"=w869:string, "System Info.Customer Details.Location"=w867:string, "ExcelData.StripPath"=w842:bool, "ExcelData.ReelCounterPerPart"=w839:i32)
            n280 = String Subset(string=w869, length (rest)=1 ("length (rest)")) -> (substring=w865:string)  [unwired: 1 in]
            n281 = String Subset(string=w867, length (rest)=3 ("length (rest)")) -> (substring=w864:string)  [unwired: 1 in]
            n282 = Number To Decimal String(number=w852) -> (decimal integer string=w862:string)  [unwired: 1 in]
            n283 = Concatenate Strings(w865, w864, "_STM_" ("string"), w862) -> (w856:string)
            n284 = Select(t=FALSE, s=w843, f=TRUE) -> (s? t:f=w849:bool)
            n285 = Select(t=FALSE, s=w843, f=w842) -> (s? t:f=w844:bool)
            n286 = Select(t=0 ("ExcelData.ReelCounterPerPart"), s=w843, f=w839) -> (s? t:f=w838:i32)
            n287 = Select(t=TRUE, s=w843, f=FALSE) -> (s? t:f=w853:bool)
            n288 = Bundle By Name(cluster=w870, "IDs.Stamping McID"=w856, "Part Info.Part Name"=w874, "Part Info.Initialize"=w843, "InitialUpdate"=w853, "ResetUpdate"=w849, "Part Info.Operator Name"=w873, "Part Info.TotalCount"=w861, "Part Info.ReelCount"=w848, "Part Info.Measurement Names Array"=w858, "Part Info.Measurement ID Array"=w859, "Part Info.Spec Values Array"=w860, "Part Info.Camera Name Array"=w857, "ExcelData.StripPath"=w844, "ExcelData.ReelCounterPerPart"=w838) -> (w846:T9)
            n289 = case shown="False" w845 {
              tunnel: [w879 "InitializeMeasAndFailArray" ("State(s) in Front (\"\")")] -> w847
              tunnel: w843 -> [w876 _]
              frame False {
                n290 = Select(t="FilePathCreation>>PartInfo\nInitializeMeasAndFailArray" ("State(s) in Front (\"\")"), s=w876, f="InitializeMeasAndFailArray" ("State(s) in Front (\"\")")) -> (s? t:f=w879:string)
              }
              frame True {
              }
            }
            n291 = call <vilib>:"Add State(s) to Queue__JKI_lib_State_Machine.vi"("State(s) in Front (\"\")"=w847, "State(s) in (\"\")"=w871) -> ("States Out"=w872:string)  [unwired: 13 in]
          }
          event User Event {
            # "For Fail,Statistical and reel, create new excel boolean should be true.\nFor events boolean will be false beacause we are creating events part from other place."
            # "Reinitialize all Excel counters to 0"
            # "Reel Info"
            n292 = event-data() -> ("Reel No"=w892:u64, "Reel Start Time Stamp"=w893:u64)  [unwired: 1 in]
            n293 = Unbundle By Name(w895) -> ("System Info.Software Features.IoT Enable"=w886:bool, "ExcelData.ReelCounterPerPart"=w884:i32, "Part Info.Part Name"=w898:string, "IDs.Stamping McID"=w900:string, "System Info.Software Features.Datalogging Features.Measurement Data"=w882:bool)
            n294 = Increment(x=w884) -> (x+1=w883:i32)
            n295 = Number To Decimal String(number=w892) -> (decimal integer string=w901:string)  [unwired: 1 in]
            n296 = Number To Decimal String(number=w893) -> (decimal integer string=w896:string)  [unwired: 1 in]
            n297 = Concatenate Strings("Batch_" ("string"), w901, "_" ("string"), w900, "_" ("string"), w898, "_" ("string"), w896) -> (w887:string)
            n298 = disable-structure shown="Disabled" {
              disable-tunnel: w891 -> [w910 _]
              disable-tunnel: w890 -> [w909 w917]
              disable-tunnel: [w908 w917] -> w889
              disable-tunnel: w887 -> [w907 _]
              disable-tunnel: w882 -> [w906 _]
              frame Disabled {
                n299 = case shown="True" w906 {
                  tunnel: w910 -> [_ w916]
                  tunnel: w909 -> [w911 w914]
                  tunnel: [w911 w913] -> w908
                  tunnel: w907 -> [_ w912]
                  frame False {
                    # "Writting Measurement Data is Disabled."
                  }
                  frame True {
                    # "Writting Measurement Data is Enabled."
                    n300 = Unbundle By Name(w916) -> ("BatchID"=w915:refnum<user-event>)
                    n301 = Generate User Event(user event=w915, event data cluster=w912, error in=w914) -> (error out=w913:errorcluster)  [unwired: 1 in, 1 out]
                  }
                }
              }
              frame Enabled {
              }
            }
            n302 = Bundle By Name(cluster=w895, "ExcelData.ReelCounterPerPart"=w883, "Reel Info.Reel No"=w892, "IDs.BatchID"=w887, "Reel Info.Reel Start Time Stamp"=w893, "ExcelData.ExcelSheetCounterPerReel"=T8 {"EventsSheetCounter"=0, "FailSheetCounter"=0, "StatisticalSheetCounter"=0, "ReelSheetCounter"=0}, "ExcelData.CreateNewExcel"=T7 {"CreateNewEventsExcel"=FALSE, "CreateNewFailExcel"=TRUE, "CreateNewStatisticalExcel"=TRUE, "CreateNewReelExcel"=TRUE}) -> (w888:T9)
            n303 = case shown="False" w886 {
              tunnel: ["FilePathCreation>>ReelInfo\nExcelFolderCreation" "Wait"] -> w905
              frame False {
              }
              frame True {
              }
            }
            n304 = call <vilib>:"Add State(s) to Queue__JKI_lib_State_Machine.vi"("State(s) in Front (\"\")"=w905, "State(s) in (\"\")"=w903) -> ("States Out"=w904:string)  [unwired: 13 in]
          }
          event User Event {
            # "Event Info"
            n305 = event-data() -> ("Event Name"=w924:string, "Event Time"=w923:string, "Event Reason"=w922:string)  [unwired: 1 in]
            n306 = Bundle By Name(cluster=w921, "Event Details.Event Name"=w924, "Event Details.Event Time"=w923, "Event Details.Event Reason"=w922) -> (w920:T9)
            n307 = call <vilib>:"Add State(s) to Queue__JKI_lib_State_Machine.vi"("State(s) in Front (\"\")"="Event Info", "State(s) in (\"\")"=w926) -> ("States Out"=w925:string)  [unwired: 13 in]
          }
          event User Event {
            # "Failure Info"
            n308 = event-data() -> ("FailTimeStamp"=w935:u64, "ControlPFArray"=w932:bool[], "SpecificationPFArray"=w936:dbl[], "RackID"=w937:u8, "FailedImageArray"=w933:T10[], "Fail Date"=w931:string, "Fail Time"=w930:string, "Fail Reason"=w929:string)  [unwired: 1 in]
            n309 = Bundle By Name(cluster=w938, "Failure Details.Fail Time Stamp"=w935, "Failure Details.ControlPFArray"=w932, "Failure Details.SpecificationPFArray"=w936, "Failure Details.Rack ID"=w937, "Failure Details.Failed Image Array"=w933, "Failure Details.Fail Date"=w931, "Failure Details.Fail Time"=w930, "Failure Details.Fail Reason"=w929) -> (w934:T9)
            n310 = call <vilib>:"Add State(s) to Queue__JKI_lib_State_Machine.vi"("State(s) in Front (\"\")"="Failure Info", "State(s) in (\"\")"=w939) -> ("States Out"=w940:string)  [unwired: 13 in]
          }
          event User Event {
            # "Statistical Info"
            n311 = event-data() -> ("Statistical Info Array"=w943:string[][])  [unwired: 1 in]
            n312 = Bundle By Name(cluster=w945, "StatisticalInfo"=w943) -> (w944:T9)
            n313 = call <vilib>:"Add State(s) to Queue__JKI_lib_State_Machine.vi"("State(s) in Front (\"\")"="MeasurementInfo", "State(s) in (\"\")"=w947) -> ("States Out"=w946:string)  [unwired: 13 in]
          }
          event User Event {
            # "Batch Info"
            n314 = event-data() -> ("Batch Pass Count"=w952:u64, "Batch Fail Count"=w951:u64)  [unwired: 1 in]
            n315 = Bundle By Name(cluster=w953, "BatchInfo.BatchPassCount"=w952, "BatchInfo.BatchFailCount"=w951) -> (w950:T9)
            n316 = call <vilib>:"Add State(s) to Queue__JKI_lib_State_Machine.vi"("State(s) in Front (\"\")"="BatchInfo", "State(s) in (\"\")"=w954) -> ("States Out"=w955:string)  [unwired: 13 in]
          }
          event User Event {
            n317 = event-data() -> ("Shift Name"=w961:string, "Shift Timing"=w962:string, "Shift End Date"=w960:string, "Statistical Shift Data"=w959:T14)  [unwired: 1 in]
            n318 = Bundle By Name(cluster=w964, "Shift Statistical Info.Shift Name"=w961, "Shift Statistical Info.Shift Timing"=w962, "Shift Statistical Info.Shift End Date"=w960, "Shift Statistical Info.Statistical Shift Data"=w959) -> (w963:T9)
            n319 = call <vilib>:"Add State(s) to Queue__JKI_lib_State_Machine.vi"("State(s) in Front (\"\")"="ShiftStatisticalInfo" ("State(s) in Front (\"\")"), "State(s) in (\"\")"=w966) -> ("States Out"=w967:string)  [unwired: 13 in]
          }
          event User Event {
            # "State Message"
            n320 = event-data() -> ("State Message"=w977:string)  [unwired: 1 in]
            n321 = Unbundle By Name(w969) -> ("System Info.Software Features.IoT Enable"=w968:bool)
            n322 = case shown="\"Save\"" w977 {
              tunnel: ["Post" "Save" "StopPost"] -> w976
              tunnel: w974 -> [w984 w993 _]
              tunnel: w973 -> [w982 w988 w1012]
              tunnel: [w981 w990 w1012] -> w972
              tunnel: w971 -> [_ _ _]
              tunnel: w968 -> [_ w986 _]
              frame "Post" {
                n323 = Unbundle By Name(w984) -> ("ActionBasedOnStateMessage"=w983:refnum<user-event>)
                n324 = Generate User Event(user event=w983, event data cluster="" ("event data"), error in=w982) -> (error out=w981:errorcluster)  [unwired: 1 in, 1 out]
              }
              frame "Save" {
                n325 = Unbundle By Name(w993) -> ("Gtron DataBase Path"=w989:path, "ActionBasedOnStateMessage"=w994:refnum<user-event>)
                n326 = case shown="True" w986 {
                  tunnel: w989 -> [_ w1002]
                  tunnel: w988 -> [w996 w1000]
                  tunnel: [w996 w997] -> w987
                  frame False {
                    # "IoT Disable"
                  }
                  frame True {
                    # "deletes all records in the PartsMeasurementMappingTable.Data might be present if internet is not there."
                    # "IoT Enable"
                    n327 = call-poly <vilib>:"Open.vi"("error in (no error)"=w1000, "db file"=w1002) -> ("error out"=w1003:errorcluster, "SQLite Connection"=w1004:refnum<class "Connection.lvclass">)  [unwired: 8 in]
                    n328 = call-poly <vilib>:"Open.vi"("error in (no error)"=w1000, "db file"=w1002) -> ("error out"=w1007:errorcluster, "SQLite Connection"=w1008:refnum<class "Connection.lvclass">)  [unwired: 8 in]
                    n329 = call-poly <vilib>:"Execute SQL (Poly).vi"("error in (no error)"=w1003, "SQL"="delete from IoTConfigDetails", "SQLite Connection in"=w1004) -> ("error out"=w1006:errorcluster, "SQLite Connection"=w1005:refnum<class "Connection.lvclass">)  [unwired: 7 in]
                    n330 = call-poly <vilib>:"Execute SQL (Poly).vi"("error in (no error)"=w1007, "SQL"="delete from PartsMeasurementMapping", "SQLite Connection in"=w1008) -> ("error out"=w1010:errorcluster, "SQLite Connection"=w1009:refnum<class "Connection.lvclass">)  [unwired: 7 in]
                    n331 = call-dynamic "Close.vi"("error in (no error)"=w1006, "SQLite Connection in"=w1005) -> ("error out"=w999:errorcluster)  [unwired: 9 in]
                    n332 = call-dynamic "Close.vi"("error in (no error)"=w1010, "SQLite Connection in"=w1009) -> ("error out"=w998:errorcluster)  [unwired: 9 in]
                    n333 = Merge Errors(w999, w998) -> (w997:errorcluster)
                  }
                }
                n334 = Generate User Event(user event=w994, event data cluster="" ("event data"), error in=w988) -> (error out=w991:errorcluster)  [unwired: 1 in, 1 out]
                n335 = Merge Errors(w987, w991) -> (w990:errorcluster)
              }
              frame "Stop Post", Default {
              }
            }
            n336 = Bundle By Name(cluster=w969, "CurrentStateMessage"=w976) -> (w970:T9)
            n337 = call <vilib>:"Add State(s) to Queue__JKI_lib_State_Machine.vi"("State(s) in Front (\"\")"="Wait" ("State(s) in Front (\"\")"), "State(s) in (\"\")"=w978) -> ("States Out"=w979:string)  [unwired: 13 in]
          }
          event User Event {
            # "Action based on State Message"
            n338 = event-data() -> ()  [unwired: 1 in, 1 out]
            n339 = Unbundle By Name(w1016) -> ("CurrentStateMessage"=w1015:string)
            n340 = case shown="Default" w1015 {
              tunnel: ["ActionBasedOnStateMessage" "Wait"] -> w1014
              frame Default {
              }
              frame "StopPost" {
              }
            }
            n341 = call <vilib>:"Add State(s) to Queue__JKI_lib_State_Machine.vi"("State(s) in Front (\"\")"=w1014, "State(s) in (\"\")"=w1018) -> ("States Out"=w1019:string)  [unwired: 13 in]
          }
          event User Event {
            n342 = event-data() -> ()  [unwired: 1 in, 1 out]
            n343 = Unbundle By Name(w1029) -> ("SaveAck.Loop1"=w1030:bool)
            n344 = case shown="True" w1030 {
              tunnel: w1026 -> [w1031 w1038]
              tunnel: [w1033 w1036] -> w1028
              tunnel: w1025 -> [_ w1035]
              tunnel: w1029 -> [w1034 w1036]
              tunnel: [w1031 w1037] -> w1027
              frame False {
                n345 = Bundle By Name(cluster=w1034, "SaveAck.Loop2"=TRUE ("SaveAck")) -> (w1033:T9)
              }
              frame True {
                n346 = call "Output_DL.vi"("Private Data"=w1035, "error in (no error)"=w1038, "State"="SaveACK") -> ("error out"=w1037:errorcluster)  [unwired: 8 in]
              }
            }
            n347 = call <vilib>:"Add State(s) to Queue__JKI_lib_State_Machine.vi"("State(s) in Front (\"\")"="Wait", "State(s) in (\"\")"=w1022) -> ("States Out"=w1024:string)  [unwired: 13 in]
          }
          event User Event {
            # "Stop DL"
            n348 = event-data() -> ()  [unwired: 1 in, 1 out]
            n349 = call <vilib>:"Add State(s) to Queue__JKI_lib_State_Machine.vi"("State(s) in Front (\"\")"="Macro: Exit", "State(s) in (\"\")"=w1042) -> ("States Out"=w1043:string)  [unwired: 13 in]
          }
        }
      }
      frame "---------- Core ----------" {
        n350 = call <vilib>:"Add State(s) to Queue__JKI_lib_State_Machine.vi"("State(s) in (\"\")"=w1048) -> ("States Out"=w1047:string)  [unwired: 14 in]
      }
      frame Default {
        w1058 = 42 items=["No error", "Argument error", "Memory is full", "Out of zone", "End of file", "File already open", "Generic file I/O error", "File not found", "File permission error", "Disk is full", "Duplicate path", "Too many files open", "System feature not enabled", "Resource file not found", "Cannot add resource", "Resource not found", "Image not found", "Image memory error", "Pen does not exist", "Config type invalid", "Config token not found", "Config parse error", "Config memory error", "Bad external code format", "Bad external code offset", "External code not present", "Null window", "Destroy window error", "Null menu", "Print aborted", "Bad print record", "Print driver error", "Windows error during printing", "Memory error during printing", "Print dialog error", "Generic print error", "Invalid device refnum", "Device not found", "Device parameter error", "Device unit error", "Cannot open device", "Device call aborted", "Generic error", "Cancelled by user", "Object ID too low", "Object ID too high", "Object not in heap", "Unknown heap", "Unknown object (invalid DefProc)", "Unknown object (DefProc not in table)", "Message out of range", "Invalid (null) method", "Unknown message", "Manager call not supported", "Bad address", "Network operation in progress", "Network operation timed out", "Connection is busy", "Network attribute not supported", "Network error", "Address in use", "System out of memory", "Connection aborted", "Connection refused", "Not connected", "Already connected", "Connection closed", "Initialization error (interapplication manager)", "Bad occurrence", "Wait on unbound occurrence handler", "Occurrence queue overflow", "Datalog type conflict", "Unused", "Unrecognized type (interapplication manager)", "Memory corrupt", "Failed to make temporary DLL", "Old CIN version", "Drag socket not found", "Failed to load drop-object", "Failed to register OLE object", "Failed to release OLE object", "Format specifier type mismatch", "Unknown format specifier", "Too few format specifiers", "Too many format specifiers", "Scan failed", "Newer CIN version", "Error converting to variant", "Runtime menu error", "Password tampered", "Variant attribute not found", "Incompatible variant data type", "Event data is not available", "Event Store is not present", "Occurrence is not found", "Event Queue is not created", "Event info is not available", "Refnum passed is NULL", "Error retrieving Class GUID", "Error retrieving CoClass GUID", "Error retrieving TypeLib GUID.", "Bad built application magic bytes.", "Specific driver is different from the specific driver associated with the Logical Name.", "There is no session opened to the class driver.", "Max Error", "MAX - Error with config objects", "MAX - Error loading configuration", "MAX - Group not supported"]
        # "Current State"
        # "Do not delete, rename, or modify this frame.\n(this is used to capture unhandled states and typos)"
        # "Handle mistyped state name (developer tool)"
        n351 = Format Into String(format string="Software Exception: Unhandled State \"%s\"." ("message"), error in=w1054, w1050) -> (resulting string=w1057:string, error out=w1056:errorcluster)  [unwired: 1 in]
        n352 = call <vilib>:"Error Cluster From Error Code.vi"("show call chain? (False)"=TRUE, "error in (no error)"=w1056, "error message (\"\")"=w1057, "error code (0)"=w1058) -> ("error out"=w1055:errorcluster)  [unwired: 5 in]
        n353 = call <vilib>:"Add State(s) to Queue__JKI_lib_State_Machine.vi"("State(s) in (\"\")"=w1053) -> ("States Out"=w1052:string)  [unwired: 14 in]
      }
      frame "Initialize Core Data" {
        # "Do not delete, rename, or modify this frame.\n(this is used to determine panel behavior on exit)"
        # "originally closed?"
        # "exe?"
        # "If panel starts closed or is an EXE, then close it when we exit"
        n354 = property class="VI"() -> ("Front Panel.Open"=w1068:bool)  [unwired: 2 in, 2 out]
        n355 = Not(x=w1068) -> (.not. x?=w1065:bool)
        n356 = property class="App"() -> ("App.Kind"=w1067:T4)  [unwired: 2 in, 2 out]
        n357 = Equal?(x=w1067, y=T4."Run Time System" ("Application:Kind")) -> (x = y?=w1064:bool)
        n358 = control-ref of="Current VI Reference"() -> (w1061:refnum<vi>)
        n359 = Or(x=w1065, y=w1064) -> (x .or. y?=w1062:bool)
        n360 = Bundle By Name(cluster=w1063, "Core.Current VI Reference"=w1061, "Core.Close Panel on Exit?"=w1062) -> (w1060:T9)
        n361 = call <vilib>:"Add State(s) to Queue__JKI_lib_State_Machine.vi"("State(s) in (\"\")"=w1071) -> ("States Out"=w1070:string)  [unwired: 14 in]
      }
      frame "Error Handler" {
        n362 = call <vilib>:"Add State(s) to Queue__JKI_lib_State_Machine.vi"("State(s) in Front (\"\")"="/* Post Error States", "State(s) in (\"\")"=w1076) -> ("States Out"=w1075:string)  [unwired: 13 in]
      }
      frame "Exit" {
        n363 = call <vilib>:"Add State(s) to Queue__JKI_lib_State_Machine.vi"("State(s) in (\"\")"=w1081) -> ("States Out"=w1080:string)  [unwired: 14 in]
      }
      frame "---------- Data ----------" {
        n364 = call <vilib>:"Add State(s) to Queue__JKI_lib_State_Machine.vi"("State(s) in (\"\")"=w1085) -> ("States Out"=w1084:string)  [unwired: 14 in]
      }
      frame "Data: Initialize" {
        w1087 = T15 {"EventsRecordCounter"=0, "FailRecordCounter"=0, "ReelRecordCounter"=0, "StatisticalRecordCounter"=0}  # RecordsInExcelCounter
        w1088 = T7 {"CreateNewEventsExcel"=FALSE, "CreateNewFailExcel"=FALSE, "CreateNewStatisticalExcel"=FALSE, "CreateNewReelExcel"=FALSE}  # CreateNewExcel
        w1089 = T8 {"EventsSheetCounter"=0, "FailSheetCounter"=0, "StatisticalSheetCounter"=0, "ReelSheetCounter"=0}  # ExcelSheetCounterPerReel
        w1090 = 0  # ReelCounterPerPart
        w1091 = FALSE  # StripPath
        w1092 = bool[] []  # Measurement Enable/Disable Array
        w1096 = 0  # SaveFailedImageCounter
        w1097 = FALSE  # ResetUpdate
        w1099 = TRUE  # InitialUpdate
        w1100 = TRUE  # IoTDetailsCounter
        w1098 = FALSE  # AddSuccessfull
        w1094 = TRUE  # Initialize
        # "Loop 1:Main IoT loop.\nLoop 2:Measurement Loop.\nDuring software exit,save will be sent to both the DL loops.\nNow when anyone of the SaveAck(either from loop 1 or 2) comes first,at that time make SaveAck boolean true.Now when the other SaveAck comes(either from loop 1 or 2),\nsend SaveAck to StateMachine."
        # "Counts the no of records that are there in one excel"
        # "For example:\nStatisticalExcel is completely filled.So a new statistical excel has to be created.We will make CreateNewStatisticalExcel as true.CreateNewExcel(Events,Fail<reel) will be false.So when we go to  \nExcelFolderCreation state,we check that which CreateNewExcel(Reel,Fail,Reel,Statistical) booean is/are true.On that basis we will create new excel.\nReinitialize all to"
        # "Counts the no of sheets created for one reel"
        # "Counts the no of reel inspected per part\nGets reinitialized to 0 on part details when initialize is true."
        # "StripPath :\nThis boolean tells us whether a path is already built or not.\nIt can either be true or false\nTrue: A portion of the already built path has to be stripped to make the new current path.\nFalse: No path is existing.So no part of the path has to be stripped to make the new current path."
        # "Measurement Enable/Disable array contains which all\nmeasurements of the selected part is/are enabled and which all is/are disabled.\nTrue=Meas. Enabled for the selected part.\nFalse=Meas. Disabled for the selected part."
        # "true=Successfull\nfalse=Not..."
        # "True=Not updated initially\nFalse=Updated"
        # "True=Post.\nFalse=Already Posted."
        # "False=Add\nTrue=Added"
        # "1=SaveImages(Images are there to be saved.This counter is made 1 from FailureInfo State.)\n0=Images not available."
        n365 = Bundle By Name(cluster=T9 {"Core"={"Current VI Reference"=refnum, "Close Panel on Exit?"=FALSE}, "System Info"={"System Name"="", "System ID"="", "Version"="", "Year"="", "Customer Details"={"Customer Name"="", "Customer ID"="", "Location"="", "No of Shifts"=0, "Shift Details Array"=[]}, "Software Features"={"IoT Enable"=FALSE, "Datalogging Features"={"Event Data"=FALSE, "Measurement Data"=FALSE, "Statistical Data"=FALSE, "Reel Data"=FALSE, "Failed Measurement Data"=FALSE, "Failed Images"=FALSE}, "IoT"={"SMS Alert Enable"=FALSE, "Email Alert Enable"=FALSE}, "Popup Enable?"={"Fail"=FALSE, "Pause"=FALSE, "Stop"=FALSE}}}, "Part Info"={"Part Name"="", "Rack ID"=0, "Initialize"=FALSE, "StampingMc No"=0, "Operator Name"="", "ReelCount"=0, "TotalCount"=0, "Measurement Names Array"=[], "Measurement ID Array"=[], "Spec Values Array"=[], "Camera Name Array"=[], "Measurement Enable/Disable Array"=[], "Number of Measurements"=0}, "Fail Counter(For Event Details)"=0, "Event Details"={"Event Name"="", "Event Time"="", "Event Reason"="", "Previous Event Name"="", "Previous Event Time"=""}, "StatisticalInfo"=[], "BatchInfo"={"BatchPassCount"=0, "BatchFailCount"=0}, "Failure Details"={"Fail Time Stamp"=0, "ControlPFArray"=[], "SpecificationPFArray"=[], "Rack ID"=0, "Failed Image Array"=[], "Fail Date"="", "Fail Time"="", "Fail Reason"=""}, "SaveFailedImageCounter"=0, "AllPartInfoArray"=[], "Status"=FALSE, "SpecValues(ForUpdate)"={"LCL"=0.0, "UCL"=0.0, "LSL"=0.0, "USL"=0.0, "Nominal Value"=0.0}, "AddSuccessfull"=FALSE, "CurrentStateMessage"="", "IoTDetailsCounter"=FALSE, "InitialUpdate"=FALSE, "ResetUpdate"=FALSE, "SetCounter"={"MeasurementDetailsSetCounter"=0, "BatchDetailsSetCounter"=0, "FailureDetailsSetCounter"=0, "EventDetailsSetCounter"=0}, "IndexCounter"={"MeasurementDetailsIndexCounter"=0, "BatchDetailsIndexCounter"=0, "FailureDetailsIndexCounter"=0, "EventDetailsIndexCounter"=0}, "Details2D"={"MeasurementDetails(2D)"=[], "BatchDetails(2D)"=[], "FailureDetails(2D)"=[], "EventDetails(2D)"=[]}, "IDs"={"Stamping McID"="", "Inspection McID"="", "BatchID"="", "FailID"=""}, "Reel Info"={"Reel No"=0, "Reel Start Time Stamp"=0}, "ExcelData"={"StripPath"=FALSE, "ReelCounterPerPart"=0, "FilePaths"={"EventsFilePath"=path "", "FailFilePath"=path "", "ReelFilePath"=path "", "StatisticalFilePath"=path ""}, "ExcelSheetCounterPerReel"={"EventsSheetCounter"=0, "FailSheetCounter"=0, "StatisticalSheetCounter"=0, "ReelSheetCounter"=0}, "CreateNewExcel"={"CreateNewEventsExcel"=FALSE, "CreateNewFailExcel"=FALSE, "CreateNewStatisticalExcel"=FALSE, "CreateNewReelExcel"=FALSE}, "RecordsInExcelCounter"={"EventsRecordsCounter"=0, "FailRecordsCounter"=0, "ReelRecordsCounter"=0, "StatisticalRecordsCounter"=0}}, "SaveAck"={"Loop1"=FALSE, "Loop2"=FALSE}, "Shift Statistical Info"={"Shift Name"="", "Shift Timing"="", "Shift End Date"="", "Statistical Shift Data"=[]}}, "Part Info.Initialize"=w1094, "IoTDetailsCounter"=w1100, "InitialUpdate"=w1099, "AddSuccessfull"=w1098, "ResetUpdate"=w1097, "SaveFailedImageCounter"=w1096, "Part Info.Measurement Enable/Disable Array"=w1092, "ExcelData.StripPath"=w1091, "ExcelData.ReelCounterPerPart"=w1090, "ExcelData.ExcelSheetCounterPerReel"=w1089, "ExcelData.CreateNewExcel"=w1088, "ExcelData.RecordsInExcelCounter"=w1087, "SaveAck"=cluster{"Loop1":bool, "Loop2":bool} {"Loop1"=FALSE, "Loop2"=FALSE}) -> (w1095:T9)
        n366 = call <vilib>:"Add State(s) to Queue__JKI_lib_State_Machine.vi"("State(s) in (\"\")"=w1103) -> ("States Out"=w1102:string)  [unwired: 14 in]
      }
      frame "Data: Cleanup" {
        n367 = Unbundle By Name(w1130) -> ("Core.Current VI Reference"=w1104:refnum<vi>)
        n368 = Close Reference(reference=w1104, error in (no error)=w1131) -> (error out=w1129:errorcluster)
        n369 = Unbundle By Name(w1125) -> ("Initialize System Info"=w1124:refnum<user-event>, "PartInfo"=w1123:refnum<user-event>, "Reel Info"=w1122:refnum<user-event>, "Event Info"=w1121:refnum<user-event>, "Failure Info"=w1120:refnum<user-event>, "Statistical Info"=w1119:refnum<user-event>, "Batch Info"=w1118:refnum<user-event>, "ActionBasedOnStateMessage"=w1117:refnum<user-event>, "SaveAckFromMeas.Loop"=w1106:refnum<user-event>)
        n370 = Flush Event Queue(0:w1127, 3:w1129) -> (8:w1126:refnum<event-registration>, 11:w1128:errorcluster)  [unwired: 4 in, 1 out]
        n371 = Unregister For Events(event registration refnum=w1126, error in=w1128) -> (error out=w1105:errorcluster)
        n372 = Destroy User Event(user event=w1124, error in=w1105) -> (error out=w1116:errorcluster)
        n373 = Destroy User Event(user event=w1123, error in=w1105) -> (error out=w1115:errorcluster)
        n374 = Destroy User Event(user event=w1122, error in=w1105) -> (error out=w1114:errorcluster)
        n375 = Destroy User Event(user event=w1121, error in=w1105) -> (error out=w1113:errorcluster)
        n376 = Destroy User Event(user event=w1120, error in=w1105) -> (error out=w1112:errorcluster)
        n377 = Destroy User Event(user event=w1119, error in=w1105) -> (error out=w1111:errorcluster)
        n378 = Destroy User Event(user event=w1118, error in=w1105) -> (error out=w1110:errorcluster)
        n379 = Destroy User Event(user event=w1117, error in=w1105) -> (error out=w1109:errorcluster)
        n380 = Destroy User Event(user event=w1106, error in=w1105) -> (error out=w1107:errorcluster)
        n381 = Merge Errors(w1116, w1115, w1114, w1113, w1112, w1111, w1110, w1109, w1107) -> (w1108:errorcluster)
        n382 = call <vilib>:"Add State(s) to Queue__JKI_lib_State_Machine.vi"("State(s) in (\"\")"=w1133) -> ("States Out"=w1132:string)  [unwired: 14 in]
      }
      frame "---------- UI ----------" {
        n383 = call <vilib>:"Add State(s) to Queue__JKI_lib_State_Machine.vi"("State(s) in (\"\")"=w1137) -> ("States Out"=w1136:string)  [unwired: 14 in]
      }
      frame "UI: Initialize" {
        n384 = call <vilib>:"Add State(s) to Queue__JKI_lib_State_Machine.vi"("State(s) in (\"\")"=w1141) -> ("States Out"=w1140:string)  [unwired: 14 in]
      }
      frame "UI: Front Panel State" {
        # "Argument"
        n385 = Unbundle By Name(w1144) -> ("Core.Current VI Reference"=w1143:refnum<vi>)
        n386 = case shown="\"Open\", Default" w1142 {
          tunnel: w1146 -> [w1152 w1165]
          tunnel: [w1154 w1166] -> w1145
          tunnel: w1143 -> [w1153 w1163]
          frame "Open", Default {
            n387 = property class="VI"(reference=w1153, error in=w1152) -> (reference out=w1150:refnum<vi>, error out=w1151:errorcluster, "Front Panel.Open"=w1149:bool)
            n388 = case shown="False" w1149 {
              tunnel: [w1157 w1160] -> w1154
              tunnel: w1151 -> [w1156 w1160]
              tunnel: w1150 -> [w1155 _]
              frame False {
                n389 = invoke class="VI" method="FP.Open"(reference=w1155, error in=w1156, "Activate"=TRUE, "State"=T5."Standard") -> (error out=w1157:errorcluster)  [unwired: 1 in, 4 out]
              }
              frame True {
              }
            }
          }
          frame "Close" {
            n390 = property class="VI"(reference=w1163, error in=w1165) -> (reference out=w1162:refnum<vi>, error out=w1164:errorcluster, "Front Panel.Open"=w1161:bool)
            n391 = case shown="True" w1161 {
              tunnel: [w1167 w1170] -> w1166
              tunnel: w1164 -> [w1167 w1169]
              tunnel: w1162 -> [_ w1168]
              frame False {
              }
              frame True {
                n392 = invoke class="VI" method="FP.Close"(reference=w1168, error in=w1169) -> (error out=w1170:errorcluster)  [unwired: 1 in, 2 out]
              }
            }
          }
        }
        n393 = call <vilib>:"Add State(s) to Queue__JKI_lib_State_Machine.vi"("State(s) in (\"\")"=w1148) -> ("States Out"=w1147:string)  [unwired: 14 in]
      }
      frame "---------- Macro ----------" {
        n394 = call <vilib>:"Add State(s) to Queue__JKI_lib_State_Machine.vi"("State(s) in (\"\")"=w1174) -> ("States Out"=w1173:string)  [unwired: 14 in]
      }
      frame "Macro: Initialize" {
        w1177 = "Data: Initialize\nInitialize Core Data\nUI: Initialize\nUI: Front Panel State >> Close"  # Data: Initialize Initialize Core Data UI: Initialize UI: Front Panel State >> Close
        n395 = call <vilib>:"Add State(s) to Queue__JKI_lib_State_Machine.vi"("State(s) in Front (\"\")"=w1177, "State(s) in (\"\")"=w1180, "State(s) at Back (\"\")"="Send Acknowledgement" ("State(s) in Front (\"\")")) -> ("States Out"=w1179:string)  [unwired: 12 in]
      }
      frame "Macro: Exit" {
        n396 = Unbundle By Name(w1187) -> ("Core.Close Panel on Exit?"=w1186:bool)
        n397 = Select(t="UI: Front Panel State >> Close", s=w1186, f="") -> (s? t:f=w1183:string)
        n398 = call <vilib>:"Add State(s) to Queue__JKI_lib_State_Machine.vi"("State(s) in (\"\")"=w1183, "State(s) at Back (\"\")"="Data: Cleanup\nExit") -> ("States Out"=w1181:string)  [unwired: 13 in]
        n399 = call <vilib>:"Add State(s) to Queue__JKI_lib_State_Machine.vi"("State(s) in Front (\"\")"=w1181, "State(s) in (\"\")"=w1190) -> ("States Out"=w1189:string)  [unwired: 13 in]
      }
      frame "---------- New Category ----------" {
        n400 = call <vilib>:"Add State(s) to Queue__JKI_lib_State_Machine.vi"("State(s) in (\"\")"=w1194) -> ("States Out"=w1193:string)  [unwired: 14 in]
      }
      frame "Send Acknowledgement" {
        w1196 = T16 {"Acknowledgement"={"Enqueuer"=refnum, "VIReference"=refnum, "VIName"=""}, "ErrorMessage"=""}  # OutputCluster
        n401 = Unbundle By Name(w1205) -> ("Core.Current VI Reference"=w1198:refnum<vi>)
        n402 = call <vilib>:"Read Self Enqueuer.vi"("Actor"=w1203) -> ("Self Enqueuer"=w1199:refnum<class "Message Enqueuer.lvclass">)  [unwired: 10 in]
        n403 = Bundle By Name(cluster=w1196, "Acknowledgement.Enqueuer"=w1199, "Acknowledgement.VIReference"=w1198, "Acknowledgement.VIName"="Data Logger" ("Name")) -> (w1195:T16)
        n404 = call "Output_DL.vi"("Private Data"=w1203, "error in (no error)"=w1201, "OutputCluster"=w1195, "State"="Launch ACK") -> ("error out"=w1200:errorcluster)  [unwired: 7 in]
        n405 = call <vilib>:"Add State(s) to Queue__JKI_lib_State_Machine.vi"("State(s) in Front (\"\")"="InitializeEventAndBatchArray" ("State(s) in Front (\"\")"), "State(s) in (\"\")"=w1207) -> ("States Out"=w1206:string)  [unwired: 13 in]
      }
      frame "InitializeEventAndBatchArray" {
        # "Create new excel for only events boolean will be true.\nOther booleans will be false."
        n406 = Initialize Array("", 20 ("dimension size"), 7 ("dimension size")) -> (w1215:string[][])
        n407 = Initialize Array("", 10 ("dimension size"), 8 ("dimension size")) -> (w1209:string[][])
        n408 = Bundle By Name(cluster=w1214, "Details2D.EventDetails(2D)"=w1215, "Details2D.BatchDetails(2D)"=w1209, "ExcelData.CreateNewExcel"=T7 {"CreateNewEventsExcel"=TRUE, "CreateNewFailExcel"=FALSE, "CreateNewStatisticalExcel"=FALSE, "CreateNewReelExcel"=FALSE}) -> (w1213:T9)
        n409 = call <vilib>:"Add State(s) to Queue__JKI_lib_State_Machine.vi"("State(s) in Front (\"\")"="Wait" ("State(s) in Front (\"\")"), "State(s) in (\"\")"=w1222) -> ("States Out"=w1221:string)  [unwired: 13 in]
      }
      frame "DBTableCreation" {
        # "Creating PartsMeasurementMapping Table"
        # "Creating MeasurementDetails Table"
        # "Creating IoTConfigDetails Table"
        # "Creating FailureDetails Table"
        # "Creating EventDetails Table"
        # "LabVIEW throws an error if the table  already exists.so clearing the error."
        # "Creating BatchDetails Table"
        n410 = Unbundle By Name(w1274) -> ("Gtron DataBase Path"=w1227:path)
        n411 = Strip Path(path=w1227) -> (stripped path=w1231:path)  [unwired: 1 out]
        n412 = call <vilib>:"Check if File or Folder Exists.vi"("error in (no error)"=w1226, "path"=w1231) -> ("error out"=w1228:errorcluster, "file or folder exists?"=w1230:bool, "dup path"=w1229:path)  [unwired: 7 in]
        n413 = case shown="True" w1230 {
          tunnel: w1229 -> [_ w1281]
          tunnel: [w1278 w1280] -> w1224
          tunnel: w1228 -> [w1278 w1279]
          frame True {
          }
          frame False {
            n414 = Create Folder(path (use dialog)=w1281, error in=w1279) -> (error out=w1280:errorcluster)  [unwired: 1 in, 2 out]
          }
        }
        n415 = call-poly <vilib>:"Open.vi"("error in (no error)"=w1224, "db file"=w1227) -> ("error out"=w1223:errorcluster, "SQLite Connection"=w1271:refnum<class "Connection.lvclass">)  [unwired: 8 in]
        n416 = call-poly <vilib>:"Open.vi"("error in (no error)"=w1224, "db file"=w1227) -> ("error out"=w1239:errorcluster, "SQLite Connection"=w1266:refnum<class "Connection.lvclass">)  [unwired: 8 in]
        n417 = call-poly <vilib>:"Open.vi"("error in (no error)"=w1224, "db file"=w1227) -> ("error out"=w1240:errorcluster, "SQLite Connection"=w1261:refnum<class "Connection.lvclass">)  [unwired: 8 in]
        n418 = call-poly <vilib>:"Open.vi"("error in (no error)"=w1224, "db file"=w1227) -> ("error out"=w1241:errorcluster, "SQLite Connection"=w1257:refnum<class "Connection.lvclass">)  [unwired: 8 in]
        n419 = call-poly <vilib>:"Open.vi"("error in (no error)"=w1224, "db file"=w1227) -> ("error out"=w1242:errorcluster, "SQLite Connection"=w1252:refnum<class "Connection.lvclass">)  [unwired: 8 in]
        n420 = call-poly <vilib>:"Open.vi"("error in (no error)"=w1224, "db file"=w1227) -> ("error out"=w1238:errorcluster, "SQLite Connection"=w1235:refnum<class "Connection.lvclass">)  [unwired: 8 in]
        n421 = call-poly <vilib>:"Execute SQL (Poly).vi"("error in (no error)"=w1223, "SQL"="Create Table BatchDetails(BatchID,PartName,StampingMcId,InspectionMcId,OperatorName,BatchCount,BatchPassCount,BatchFailCount) ", "SQLite Connection in"=w1271) -> ("error out"=w1273:errorcluster, "SQLite Connection"=w1270:refnum<class "Connection.lvclass">)  [unwired: 7 in]
        n422 = call-poly <vilib>:"Execute SQL (Poly).vi"("error in (no error)"=w1239, "SQL"="Create Table EventDetails(BatchId,FailId,InspectionMcId,EventName,EventTime,EventReason,NonUtilisedTime)", "SQLite Connection in"=w1266) -> ("error out"=w1264:errorcluster, "SQLite Connection"=w1267:refnum<class "Connection.lvclass">)  [unwired: 7 in]
        n423 = call-poly <vilib>:"Execute SQL (Poly).vi"("error in (no error)"=w1240, "SQL"="Create table FailureDetails(FailId,BatchId,PartName,MeasurementName,FailedTerminalValues)", "SQLite Connection in"=w1261) -> ("error out"=w1263:errorcluster, "SQLite Connection"=w1260:refnum<class "Connection.lvclass">)  [unwired: 7 in]
        n424 = call-poly <vilib>:"Execute SQL (Poly).vi"("error in (no error)"=w1241, "SQL"="Create Table IoTConfigDetails(ClientId,ClientName,Location,NoOfShifts,RunningShift,ShiftTiming,InspectionMcId,IoTEnable,SMSAlertEnable,EmailAlertEnable,PopupEnable)", "SQLite Connection in"=w1257) -> ("error out"=w1255:errorcluster, "SQLite Connection"=w1258:refnum<class "Connection.lvclass">)  [unwired: 7 in]
        n425 = call-poly <vilib>:"Execute SQL (Poly).vi"("error in (no error)"=w1242, "SQL"="Create Table MeasurementDetails(BatchId,PartName,MeasurementName,LSL,USL,NominalValue,LCL,UCL,Mean,StandardDeviation,Variance,Cp,Cpk)", "SQLite Connection in"=w1252) -> ("error out"=w1254:errorcluster, "SQLite Connection"=w1251:refnum<class "Connection.lvclass">)  [unwired: 7 in]
        n426 = call-poly <vilib>:"Execute SQL (Poly).vi"("error in (no error)"=w1238, "SQL"="Create Table PartsMeasurementMapping(PartName,MeasurementName,LSL,USL,LCL,UCL,InspectionMcId,Status,NominalValue)", "SQLite Connection in"=w1235) -> ("error out"=w1233:errorcluster, "SQLite Connection"=w1236:refnum<class "Connection.lvclass">)  [unwired: 7 in]
        n427 = call <vilib>:"Clear Errors.vi"("error in (no error)"=w1273) -> ("error out"=w1272:errorcluster)  [unwired: 5 in, 1 out]
        n428 = call <vilib>:"Clear Errors.vi"("error in (no error)"=w1264) -> ("error out"=w1265:errorcluster)  [unwired: 5 in, 1 out]
        n429 = call <vilib>:"Clear Errors.vi"("error in (no error)"=w1263) -> ("error out"=w1262:errorcluster)  [unwired: 5 in, 1 out]
        n430 = call <vilib>:"Clear Errors.vi"("error in (no error)"=w1255) -> ("error out"=w1256:errorcluster)  [unwired: 5 in, 1 out]
        n431 = call <vilib>:"Clear Errors.vi"("error in (no error)"=w1254) -> ("error out"=w1253:errorcluster)  [unwired: 5 in, 1 out]
        n432 = call <vilib>:"Clear Errors.vi"("error in (no error)"=w1233) -> ("error out"=w1234:errorcluster)  [unwired: 5 in, 1 out]
        n433 = call-dynamic "Close.vi"("error in (no error)"=w1272, "SQLite Connection in"=w1270) -> ("error out"=w1269:errorcluster)  [unwired: 9 in]
        n434 = call-dynamic "Close.vi"("error in (no error)"=w1265, "SQLite Connection in"=w1267) -> ("error out"=w1248:errorcluster)  [unwired: 9 in]
        n435 = call-dynamic "Close.vi"("error in (no error)"=w1262, "SQLite Connection in"=w1260) -> ("error out"=w1247:errorcluster)  [unwired: 9 in]
        n436 = call-dynamic "Close.vi"("error in (no error)"=w1256, "SQLite Connection in"=w1258) -> ("error out"=w1246:errorcluster)  [unwired: 9 in]
        n437 = call-dynamic "Close.vi"("error in (no error)"=w1253, "SQLite Connection in"=w1251) -> ("error out"=w1245:errorcluster)  [unwired: 9 in]
        n438 = call-dynamic "Close.vi"("error in (no error)"=w1234, "SQLite Connection in"=w1236) -> ("error out"=w1232:errorcluster)  [unwired: 9 in]
        n439 = Merge Errors(w1269, w1248, w1247, w1246, w1245, w1232) -> (w1244:errorcluster)
        n440 = call <vilib>:"Add State(s) to Queue__JKI_lib_State_Machine.vi"("State(s) in Front (\"\")"="Wait" ("State(s) in Front (\"\")"), "State(s) in (\"\")"=w1277) -> ("States Out"=w1276:string)  [unwired: 13 in]
      }
      frame "FilePathCreation" {
        n441 = call "File Path Creation.vi"("ErrorIN"=w1285, "DL PrivateDataIN"=w1288, "State"=w1289, "LocalDataIN"=w1287) -> ("ErrorOUT"=w1284:errorcluster, "LocalDataOUT"=w1286:T9)  [unwired: 6 in]
        n442 = call <vilib>:"Add State(s) to Queue__JKI_lib_State_Machine.vi"("State(s) in (\"\")"=w1282) -> ("States Out"=w1283:string)  [unwired: 14 in]
      }
      frame "ExcelFolderCreation" {
        n443 = call "Excel File and Folder Creation.vi"("ErrorIN"=w1294, "LocalDataIN"=w1292) -> ("error out"=w1291:errorcluster, "LocalDataOUT"=w1293:T9)  [unwired: 8 in]
        n444 = call <vilib>:"Add State(s) to Queue__JKI_lib_State_Machine.vi"("State(s) in Front (\"\")"="Wait" ("State(s) in Front (\"\")"), "State(s) in (\"\")"=w1295) -> ("States Out"=w1296:string)  [unwired: 13 in]
      }
      frame "InitializeAllPartInfo" {
        w1315 = T17 {"Customer ID"="", "Customer Name"="", "Location"="", "No of Shifts"=0, "Inspection McID"="", "Shift Details Array"=[], "IoT Enable"=FALSE, "SMS Alert Enable"=FALSE, "Email Alert Enable"=FALSE, "FailPopupEnable"=FALSE, "PausePopupEnable"=FALSE, "StopPopupEnable"=FALSE}  # IoT Configuration cluster
        n445 = Unbundle By Name(w1318) -> ("IDs.Inspection McID"=w1324:string, "AllPartInfoArray"=w1325:T3, "System Info.Customer Details.Customer ID"=w1314:string, "System Info.Customer Details.Customer Name"=w1303:string, "System Info.Customer Details.Location"=w1304:string, "System Info.Customer Details.No of Shifts"=w1305:u8, "IDs.Inspection McID"=w1306:string, "System Info.Customer Details.Shift Details Array"=w1307:cluster{"Name":string, "Timing":string}[], "System Info.Software Features.IoT Enable"=w1308:bool, "System Info.Software Features.IoT.SMS Alert Enable"=w1309:bool, "System Info.Software Features.IoT.Email Alert Enable"=w1310:bool, "System Info.Software Features.Popup Enable?.Fail"=w1311:bool, "System Info.Software Features.Popup Enable?.Pause"=w1312:bool, "System Info.Software Features.Popup Enable?.Stop"=w1313:bool)
        n446 = Unbundle By Name(w1323) -> ("Gtron DataBase Path"=w1301:path)
        n447 = Bundle By Name(cluster=w1315, "Customer ID"=w1314, "Customer Name"=w1303, "Location"=w1304, "No of Shifts"=w1305, "Inspection McID"=w1306, "Shift Details Array"=w1307, "IoT Enable"=w1308, "SMS Alert Enable"=w1309, "Email Alert Enable"=w1310, "FailPopupEnable"=w1311, "PausePopupEnable"=w1312, "StopPopupEnable"=w1313) -> (w1302:T17)
        n448 = for {
          tunnel: w1325 -> [w1333] mode=indexing
          tunnel: w1321 -> [w1337]
          tunnel: w1324 -> [w1336]
          tunnel: w1301 -> [w1335]
          tunnel: [w1334] -> w1322
          n449 = Unbundle By Name(w1333) -> ("PartName"=w1332:string, "MeasurementNamesArray"=w1331:string[], "SpecValuesArray"=w1330:T18)
          n450 = Bundle("Inspection McID"=w1336, "PartName"=w1332, "MeasurementNamesArray"=w1331, "SpecValuesArray"=w1330) -> (w1329:T19)  [unwired: 1 in]
          n451 = call "Save PartsMeasurementMapping to DB.vi"("error in"=w1337, "GTron DB"=w1335, "output cluster"=w1329) -> ("error out"=w1334:errorcluster)  [unwired: 8 in]
        }
        n452 = call "Save IoT Configuration to DB.vi"("error in"=w1321, "IoT Configuration cluster"=w1302, "GTron DB"=w1301) -> ("error out"=w1320:errorcluster)  [unwired: 7 in]
        n453 = call "POST MesaurementsMappingTable.vi"("error in"=w1322, "GTron in"=w1301) -> ("error out"=w1317:errorcluster, "DB is Empty?"=w1299:bool)  [unwired: 8 in]
        n454 = Select(t=TRUE, s=w1299, f=FALSE) -> (s? t:f=w1300:bool)
        n455 = Bundle By Name(cluster=w1318, "AddSuccessfull"=w1300) -> (w1316:T9)
        n456 = Merge Errors(w1317, w1320) -> (w1319:errorcluster)
        n457 = call <vilib>:"Add State(s) to Queue__JKI_lib_State_Machine.vi"("State(s) in Front (\"\")"="Wait" ("State(s) in Front (\"\")"), "State(s) in (\"\")"=w1327) -> ("States Out"=w1328:string)  [unwired: 13 in]
      }
      frame "InitializeMeasAndFailArray" {
        n458 = Unbundle By Name(w1358) -> ("AllPartInfoArray"=w1345:T3, "Part Info.Part Name"=w1344:string, "Part Info.Measurement Names Array"=w1343:string[], "System Info.Software Features.IoT Enable"=w1350:bool, "System Info.Software Features.Datalogging Features.Measurement Data"=w1338:bool)
        n459 = call "Create Measurement Enable Array for a part.vi"("Measurement Names Array"=w1343, "Part Name"=w1344, "AllPartInfoArray"=w1345) -> ("Measurement Enable Array"=w1346:bool[])  [unwired: 8 in]
        n460 = call "Count Number of Measurements for a Part.vi"("Part Name"=w1344, "AllPartInfoArray"=w1345) -> ("Number of Measurements"=w1347:i32)  [unwired: 9 in]
        n461 = Multiply(x=2 ("dimension size"), y=w1347) -> (x*y=w1355:i32)
        n462 = case shown="False" w1350 {
          tunnel: [w1384 5 ("dimension size")] -> w1349
          tunnel: w1347 -> [w1382 w1386]
          tunnel: [2 w1385] -> w1348
          frame False {
            # "According to the current fail data format.(7+No of meas.)"
            # "IoT Disabled"
            n463 = Add(x=w1382, y=7 ("dimension size")) -> (x+y=w1384:i32)
          }
          frame True {
            # "2 times the size. \nJust for safety."
            # "IoT Enabled"
            n464 = Multiply(x=w1386, y=2 ("x")) -> (x*y=w1385:i32)
          }
        }
        n465 = Initialize Array("", w1355, 13 ("dimension size")) -> (w1353:string[][])
        n466 = Initialize Array("", w1348, w1349) -> (w1352:string[][])
        n467 = Bundle By Name(cluster=w1358, "Part Info.Number of Measurements"=w1347, "Details2D.MeasurementDetails(2D)"=w1353, "Details2D.FailureDetails(2D)"=w1352, "Part Info.Measurement Enable/Disable Array"=w1346) -> (w1342:T9)
        n468 = disable-structure shown="Enabled" {
          disable-tunnel: w1342 -> [w1366 _]
          disable-tunnel: w1341 -> [w1365 _]
          disable-tunnel: w1340 -> [w1364 w1380]
          disable-tunnel: [w1363 w1380] -> w1339
          disable-tunnel: w1338 -> [w1362 _]
          frame Disabled {
            n469 = case "PartDetails sent to loop2" shown="True" w1362 {
              tunnel: w1366 -> [_ w1379]
              tunnel: w1365 -> [_ w1377]
              tunnel: w1364 -> [w1367 w1376]
              tunnel: [w1367 w1375] -> w1363
              frame False {
                # "Writting Measurement Data is Disabled."
              }
              frame True {
                # "Part details sent to measurement loop."
                # "Writting Measurement Data is Enabled."
                n470 = Unbundle By Name(w1379) -> ("Part Info.Part Name"=w1374:string, "Part Info.Operator Name"=w1373:string, "Part Info.Initialize"=w1372:bool, "Part Info.Measurement Enable/Disable Array"=w1371:bool[], "Part Info.Number of Measurements"=w1370:i32)
                n471 = Unbundle By Name(w1377) -> ("PartDetails"=w1378:refnum<user-event>)
                n472 = Bundle By Name(cluster="PartDetails", "PartName"=w1374, "OperatorName"=w1373, "Initialize"=w1372, "MeasurementDataEnableArray"=w1371, "NumbeOfMeasurements"=w1370) -> (w1368:T1)
                n473 = Generate User Event(user event=w1378, event data cluster=w1368, error in=w1376) -> (error out=w1375:errorcluster)  [unwired: 1 in, 1 out]
              }
            }
          }
          frame Enabled {
          }
        }
        n474 = call <vilib>:"Add State(s) to Queue__JKI_lib_State_Machine.vi"("State(s) in Front (\"\")"="Wait" ("State(s) in Front (\"\")"), "State(s) in (\"\")"=w1360) -> ("States Out"=w1361:string)  [unwired: 13 in]
      }
      frame "Event Info" {
        n475 = in-place {
          # "Nonutilised time is the time when the machine is in idle state,i.e no inspection is going on."
          # "FAIL COUNTER(FOR EVENT DETAILS)\nFail Counter can have values 0 or 1.\n0 indicates that the previous event triggered was not Failure user event.NaN will be stored for FailId in the FailId array for that corresponding event name.\n1 indicates that the previous event triggered was Failure user event.Actual generated FailId will be stored in the FailId array for that corresponding event name.The failId will be updated from the failure user event.\nThe counter is reset to 0 every time in this user event."
          # "Event data formation"
          n476 = in-place-cluster #3(w1394) -> ("ExcelData.RecordsInExcelCounter.EventsRecordsCounter"=w1412:u32, "IndexCounter.EventDetailsIndexCounter"=w1438:i32, "IDs.BatchID"=w1421:string, "Fail Counter(For Event Details)"=w1433:i32, "IDs.FailID"=w1432:string, "IDs.Inspection McID"=w1419:string, "Event Details.Event Name"=w1415:string, "Event Details.Event Time"=w1414:string, "Event Details.Event Reason"=w1423:string, "Event Details.Previous Event Name"=w1416:string, "Event Details.Previous Event Time"=w1417:string, "Details2D.EventDetails(2D)"=w1440:string[][])
          n477 = case shown="\"Start\"" w1415 {
            tunnel: [w1442 "None"] -> w1420
            tunnel: w1419 -> [w1442 _]
            frame Default {
            }
            frame "Start" {
            }
          }
          n478 = Increment(x=w1438) -> (x+1=w1441:i32)
          n479 = case shown="\"Exit\", \"Ready\", \"Select\", \"Start\"" w1415 {
            tunnel: [w1444 "None"] -> w1422
            tunnel: w1421 -> [w1444 _]
            frame Default {
            }
            frame "Exit", "Ready", "Select", "Start" {
            }
          }
          n480 = Equal?(x=w1433, y=1) -> (x = y?=w1434:bool)
          n481 = Increment(x=w1412) -> (x+1=w1413:u32)
          n482 = Select(t=w1432, s=w1434, f="None") -> (s? t:f=w1430:string)
          n483 = call "NonUtilisedTime.vi"("Event Name"=w1415, "Previous Event Time"=w1417, "Event Time"=w1414, "Previous Event Name"=w1416) -> ("Non Utilized Time"=w1418:string)  [unwired: 11 in]
          n484 = Replace Array Subset(array=w1440, new element #1=w1422, index (row) #1=w1438, index (col) #1=0 ("disabled index (col)"), new element #2=w1430, index (row) #2=w1438, index (col) #2=1 ("disabled index (col)"), new element #3=w1420, index (row) #3=w1438, index (col) #3=2 ("disabled index (col)"), new element #4=w1415, index (row) #4=w1438, index (col) #4=3 ("disabled index (col)"), new element #5=w1414, index (row) #5=w1438, index (col) #5=4 ("disabled index (col)"), new element #6=w1423, index (row) #6=w1438, index (col) #6=5 ("disabled index (col)"), new element #7=w1418, index (row) #7=w1438, index (col) #7=6 ("disabled index (col)")) -> (w1439:string[][])
          n485 = in-place-cluster #3("ExcelData.RecordsInExcelCounter.EventsRecordsCounter"=w1413, "IndexCounter.EventDetailsIndexCounter"=w1441, "IDs.BatchID"=w1421, "Fail Counter(For Event Details)"=0, "IDs.FailID"=w1432, "IDs.Inspection McID"=w1419, "Event Details.Event Name"=w1415, "Event Details.Event Time"=w1414, "Event Details.Event Reason"=w1423, "Event Details.Previous Event Name"=w1415, "Event Details.Previous Event Time"=w1414, "Details2D.EventDetails(2D)"=w1439) -> (w1391:T9)
        }
        n486 = Unbundle By Name(w1391) -> ("System Info.Software Features.IoT Enable"=w1393:bool, "ExcelData.RecordsInExcelCounter.EventsRecordsCounter"=w1392:u32)
        n487 = case shown="False" w1393 {
          tunnel: [w1398 "Wait"] -> w1389
          tunnel: w1392 -> [w1402 _]
          tunnel: [w1400 w1410] -> w1390
          tunnel: w1391 -> [w1399 w1410]
          frame False {
            # "IoT Disabled"
            n488 = Less?(x=w1402, y=u32 10001) -> (x < y?=w1401:bool)
            n489 = case shown="False" w1401 {
              tunnel: [w1405 w1409] -> w1400
              tunnel: w1399 -> [w1407 w1409]
              tunnel: ["FilePathCreation>>EventPath\nExcelFolderCreation" ("State(s) in Front (\"\")") "Wait"] -> w1398
              frame False {
                n490 = Bundle By Name(cluster=w1407, "ExcelData.CreateNewExcel.CreateNewEventsExcel"=TRUE ("ExcelData.CreateNewExcel.CreateNewFailExcel")) -> (w1405:T9)
              }
              frame True {
              }
            }
          }
          frame True {
            # "IoT Enabled"
          }
        }
        n491 = call <vilib>:"Add State(s) to Queue__JKI_lib_State_Machine.vi"("State(s) in Front (\"\")"=w1389, "State(s) in (\"\")"=w1396) -> ("States Out"=w1397:string)  [unwired: 13 in]
      }
      frame "Failure Info" {
        n492 = Unbundle By Name(w1452) -> ("System Info.Software Features.IoT Enable"=w1451:bool)
        n493 = case shown="False" w1451 {
          tunnel: w1452 -> [w1471 w1522]
          tunnel: [w1470 w1521] -> w1446
          frame False {
            # "IoT Disabled"
            n494 = in-place {
              w1497 = 1 ("Fail Counter(For Event Details)")
              # "Setting the counter indicates that the event triggered was failure Info"
              n495 = in-place-cluster #4(w1471) -> ("IDs.BatchID"=w1490:string, "Failure Details.Fail Time Stamp"=w1500:u64, "Part Info.Part Name"=w1491:string, "Part Info.Operator Name"=w1489:string, "Failure Details.Fail Date"=w1476:string, "Failure Details.Fail Time"=w1475:string, "Part Info.Measurement Enable/Disable Array"=w1485:bool[], "Failure Details.SpecificationPFArray"=w1483:dbl[], "ExcelData.RecordsInExcelCounter.FailRecordsCounter"=w1472:u32, "IndexCounter.FailureDetailsIndexCounter"=w1479:i32, "Details2D.FailureDetails(2D)"=w1488:string[][], "Failure Details.Fail Reason"=w1474:string)  [unwired: 3 out]
              n496 = Number To Decimal String(number=w1500) -> (decimal integer string=w1501:string)  [unwired: 1 in]
              n497 = Concatenate Strings(w1490, "_" ("string"), w1501) -> (w1498:string)
              n498 = Replace Array Subset(array=w1488, new element #1=w1491, index (row) #1=w1479, index (col) #1=0 ("disabled index (col)"), new element #2=w1490, index (row) #2=w1479, index (col) #2=1 ("disabled index (col)"), new element #3=w1489, index (row) #3=w1479, index (col) #3=2 ("disabled index (col)"), new element #4=w1476, index (row) #4=w1479, index (col) #4=3 ("disabled index (col)"), new element #5=w1475, index (row) #5=w1479, index (col) #5=4 ("disabled index (col)")) -> (w1487:string[][])
              n499 = for {
                shift-right: [w1508] -> w1482
                shift-left: w1487 -> [w1512]
                tunnel: w1479 -> [w1511]
                shift-right: [w1510] -> w1477
                shift-left: 5 ("disabled index (col)") -> [w1509]
                tunnel: w1485 -> [w1507] mode=indexing
                shift-right: [w1504] -> _
                shift-left: 0 ("disabled index (col)") -> [w1506]
                tunnel: w1483 -> [w1505]
                n500 = case shown="True" w1507 {
                  tunnel: w1506 -> [w1514 w1519]
                  tunnel: w1505 -> [_ w1520]
                  tunnel: [w1514 w1518] -> w1504
                  tunnel: ["Disabled" w1515] -> w1503
                  frame False {
                  }
                  frame True {
                    n501 = Index Array(array=w1520, index=w1519) -> (element=w1517:dbl)
                    n502 = Increment(x=w1519) -> (x+1=w1518:i32)
                    n503 = Number To Fractional String(number=w1517, precision (6)=3 ("disabled index (col)")) -> (F-format string=w1515:string)  [unwired: 2 in]
                  }
                }
                n504 = Increment(x=w1509) -> (x+1=w1510:i32)
                n505 = Replace Array Subset(array=w1512, new element=w1503, index (row)=w1511, index (col)=w1509) -> (w1508:string[][])
              }
              n506 = Increment(x=w1472) -> (x+1=w1473:u32)
              n507 = Increment(x=w1477) -> (x+1=w1478:i32)
              n508 = Increment(x=w1479) -> (x+1=w1499:i32)
              n509 = Replace Array Subset(array=w1482, new element #1="Fail" ("new element/subarray"), index (row) #1=w1479, index (col) #1=w1477, new element #2=w1474, index (row) #2=w1479, index (col) #2=w1478) -> (w1480:string[][])
              n510 = in-place-cluster #4("SaveFailedImageCounter"=w1497, "Fail Counter(For Event Details)"=w1497, "IDs.FailID"=w1498, "IDs.BatchID"=w1490, "Failure Details.Fail Time Stamp"=w1500, "Part Info.Part Name"=w1491, "Part Info.Operator Name"=w1489, "Failure Details.Fail Date"=w1476, "Failure Details.Fail Time"=w1475, "Part Info.Measurement Enable/Disable Array"=w1485, "Failure Details.SpecificationPFArray"=w1483, "ExcelData.RecordsInExcelCounter.FailRecordsCounter"=w1473, "IndexCounter.FailureDetailsIndexCounter"=w1499, "Details2D.FailureDetails(2D)"=w1480, "Failure Details.Fail Reason"=w1474) -> (w1470:T9)
            }
          }
          frame True {
            # "IoT Enabled"
            n511 = in-place {
              w1523 = 1 ("Fail Counter(For Event Details)")
              # "Setting the counter indicates that the event triggered was failure Info"
              n512 = in-place-cluster #5(w1522) -> ("IDs.BatchID"=w1527:string, "Failure Details.Fail Time Stamp"=w1534:u64, "Part Info.Part Name"=w1526:string, "Part Info.Measurement Names Array"=w1525:string[], "Failure Details.SpecificationPFArray"=w1524:dbl[], "Failure Details.ControlPFArray"=w1533:bool[], "Details2D.FailureDetails(2D)"=w1531:string[][], "IndexCounter.FailureDetailsIndexCounter"=w1530:i32)  [unwired: 3 out]
              n513 = Number To Decimal String(number=w1534) -> (decimal integer string=w1535:string)  [unwired: 1 in]
              n514 = Concatenate Strings(w1527, "_" ("string"), w1535) -> (w1528:string)
              n515 = for {
                shift-right: [w1545] -> w1529
                shift-left: w1530 -> [w1544]
                shift-right: [w1543] -> w1532
                shift-left: w1531 -> [w1546]
                tunnel: w1533 -> [w1542] mode=indexing
                tunnel: w1528 -> [w1541]
                tunnel: w1527 -> [w1540]
                tunnel: w1526 -> [w1539]
                tunnel: w1525 -> [w1538] mode=indexing
                tunnel: w1524 -> [w1537] mode=indexing
                n516 = case shown="False" w1542 {
                  tunnel: w1546 -> [w1547 w1564]
                  tunnel: [w1548 w1563] -> w1545
                  tunnel: w1544 -> [w1548 w1558]
                  tunnel: [w1547 w1554] -> w1543
                  tunnel: w1541 -> [_ w1553]
                  tunnel: w1540 -> [_ w1552]
                  tunnel: w1539 -> [_ w1551]
                  tunnel: w1538 -> [_ w1550]
                  tunnel: w1537 -> [_ w1549]
                  frame True {
                  }
                  frame False {
                    n517 = Number To Fractional String(number=w1549, precision (6)=i16 4) -> (F-format string=w1555:string)  [unwired: 2 in]
                    n518 = Replace Array Subset(array=w1564, new element #1=w1553, index (row) #1=w1558, index (col) #1=0 ("disabled index (col)"), new element #2=w1552, index (row) #2=w1558, index (col) #2=1 ("disabled index (col)"), new element #3=w1551, index (row) #3=w1558, index (col) #3=2 ("disabled index (col)"), new element #4=w1550, index (row) #4=w1558, index (col) #4=3 ("disabled index (col)"), new element #5=w1555, index (row) #5=w1558, index (col) #5=4 ("disabled index (col)")) -> (w1554:string[][])
                    n519 = Increment(x=w1558) -> (x+1=w1563:i32)
                  }
                }
              }
              n520 = in-place-cluster #5("SaveFailedImageCounter"=w1523, "Fail Counter(For Event Details)"=w1523, "IDs.FailID"=w1528, "IDs.BatchID"=w1527, "Failure Details.Fail Time Stamp"=w1534, "Part Info.Part Name"=w1526, "Part Info.Measurement Names Array"=w1525, "Failure Details.SpecificationPFArray"=w1524, "Failure Details.ControlPFArray"=w1533, "Details2D.FailureDetails(2D)"=w1532, "IndexCounter.FailureDetailsIndexCounter"=w1529) -> (w1521:T9)
            }
          }
        }
        n521 = Unbundle By Name(w1446) -> ("System Info.Software Features.IoT Enable"=w1450:bool, "ExcelData.RecordsInExcelCounter.FailRecordsCounter"=w1448:u32)
        n522 = case shown="False" w1450 {
          tunnel: [w1456 "Wait"] -> w1449
          tunnel: w1448 -> [w1460 _]
          tunnel: [w1458 w1468] -> w1447
          tunnel: w1446 -> [w1457 w1468]
          frame False {
            # "IoT Disabled"
            n523 = Less?(x=w1460, y=u32 10001) -> (x < y?=w1459:bool)
            n524 = case shown="False" w1459 {
              tunnel: [w1463 w1467] -> w1458
              tunnel: w1457 -> [w1465 w1467]
              tunnel: ["ExcelFolderCreation" "Wait"] -> w1456
              frame False {
                n525 = Bundle By Name(cluster=w1465, "ExcelData.CreateNewExcel.CreateNewFailExcel"=TRUE) -> (w1463:T9)
              }
              frame True {
              }
            }
          }
          frame True {
            # "IoT Enabled"
          }
        }
        n526 = call <vilib>:"Add State(s) to Queue__JKI_lib_State_Machine.vi"("State(s) in Front (\"\")"=w1449, "State(s) in (\"\")"=w1454) -> ("States Out"=w1455:string)  [unwired: 13 in]
      }
      frame "MeasurementInfo" {
        n527 = in-place {
          n528 = in-place-cluster #6(w1570) -> ("IDs.BatchID"=w1595:string, "Part Info.Part Name"=w1594:string, "Part Info.Measurement Names Array"=w1593:string[], "Part Info.Spec Values Array"=w1592:T13, "StatisticalInfo"=w1591:string[][], "ExcelData.RecordsInExcelCounter.StatisticalRecordsCounter"=w1590:u32, "Details2D.MeasurementDetails(2D)"=w1599:string[][], "IndexCounter.MeasurementDetailsIndexCounter"=w1598:i32, "System Info.Software Features.IoT Enable"=w1588:bool)
          n529 = Transpose 2D Array(2D array=w1591) -> (transposed array=w1600:string[][])
          n530 = for {
            tunnel: w1595 -> [w1609]
            tunnel: w1594 -> [w1608]
            tunnel: w1593 -> [w1607] mode=indexing
            tunnel: w1592 -> [w1606] mode=indexing
            tunnel: w1600 -> [w1602] mode=indexing
            shift-right: [w1611] -> w1597
            shift-left: w1599 -> [w1612]
            shift-right: [w1610] -> w1596
            shift-left: w1598 -> [w1605]
            shift-right: [w1603] -> w1589
            shift-left: w1590 -> [w1604]
            tunnel: w1588 -> [w1601]
            n531 = case shown="False" w1601 {
              tunnel: w1612 -> [w1616 w1675]
              tunnel: [w1614 w1674] -> w1611
              tunnel: [w1613 w1673] -> w1610
              tunnel: w1609 -> [w1619 w1672]
              tunnel: w1608 -> [w1620 w1671]
              tunnel: w1607 -> [w1621 w1670]
              tunnel: w1606 -> [w1622 w1669]
              tunnel: w1605 -> [w1618 w1668]
              tunnel: w1604 -> [w1617 w1667]
              tunnel: [w1615 w1666] -> w1603
              tunnel: w1602 -> [w1623 w1663]
              frame False {
                w1653 = i16 4 ("precision (6)")
                # "IoT Disable"
                n532 = Unbundle By Name(w1622) -> ("LSL"=w1654:dbl, "USL"=w1652:dbl, "Nominal Value"=w1651:dbl, "LCL"=w1650:dbl, "UCL"=w1649:dbl)
                n533 = Increment(x=w1617) -> (x+1=w1615:u32)
                n534 = Number To Fractional String(number=w1654, precision (6)=w1653) -> (F-format string=w1648:string)  [unwired: 2 in]
                n535 = Number To Fractional String(number=w1652, precision (6)=w1653) -> (F-format string=w1647:string)  [unwired: 2 in]
                n536 = Number To Fractional String(number=w1651, precision (6)=w1653) -> (F-format string=w1639:string)  [unwired: 2 in]
                n537 = Number To Fractional String(number=w1650, precision (6)=w1653) -> (F-format string=w1646:string)  [unwired: 2 in]
                n538 = Index Array(array=w1623, index=0) -> (element=w1633:string)
                n539 = Index Array(array=w1623, index=1) -> (element=w1631:string)
                n540 = Index Array(array=w1623, index=2) -> (element=w1629:string)
                n541 = Index Array(array=w1623, index=3) -> (element=w1625:string)
                n542 = Index Array(array=w1623, index=4) -> (element=w1624:string)
                n543 = Number To Fractional String(number=w1649, precision (6)=w1653) -> (F-format string=w1645:string)  [unwired: 2 in]
                n544 = Replace Array Subset(array=w1616, new element #1=w1619, index (row) #1=w1618, index (col) #1=0 ("disabled index (col)"), new element #2=w1620, index (row) #2=w1618, index (col) #2=1 ("disabled index (col)"), new element #3=w1621, index (row) #3=w1618, index (col) #3=2 ("disabled index (col)"), new element #4=w1648, index (row) #4=w1618, index (col) #4=3 ("disabled index (col)"), new element #5=w1647, index (row) #5=w1618, index (col) #5=4 ("disabled index (col)"), new element #6=w1639, index (row) #6=w1618, index (col) #6=5 ("disabled index (col)"), new element #7=w1646, index (row) #7=w1618, index (col) #7=6 ("disabled index (col)"), new element #8=w1645, index (row) #8=w1618, index (col) #8=7 ("disabled index (col)"), new element #9=w1633, index (row) #9=w1618, index (col) #9=8 ("disabled index (col)"), new element #10=w1631, index (row) #10=w1618, index (col) #10=9 ("disabled index (col)"), new element #11=w1629, index (row) #11=w1618, index (col) #11=10 ("disabled index (col)"), new element #12=w1625, index (row) #12=w1618, index (col) #12=11 ("disabled index (col)"), new element #13=w1624, index (row) #13=w1618, index (col) #13=12 ("disabled index (col)")) -> (w1614:string[][])
                n545 = Increment(x=w1618) -> (x+1=w1613:i32)
              }
              frame True {
                # "IoT Enable"
                n546 = Index Array(array=w1663, index=3) -> (element=w1662:string)
                n547 = Index Array(array=w1663, index=4) -> (element=w1661:string)
                n548 = case shown="\"+Inf\", \"-Inf\", \"Inf\"" w1662 {
                  tunnel: [FALSE TRUE] -> w1660
                  frame Default {
                  }
                  frame "+Inf", "-Inf", "Inf" {
                  }
                }
                n549 = case shown="\"+Inf\", \"-Inf\", \"Inf\"" w1661 {
                  tunnel: [FALSE TRUE] -> w1659
                  frame Default {
                  }
                  frame "+Inf", "-Inf", "Inf" {
                  }
                }
                n550 = Or(x=w1660, y=w1659) -> (x .or. y?=w1658:bool)
                n551 = case shown="False" w1658 {
                  tunnel: w1675 -> [w1724 w1726]
                  tunnel: [w1723 w1726] -> w1674
                  tunnel: [w1722 w1725] -> w1673
                  tunnel: w1672 -> [w1720 _]
                  tunnel: w1671 -> [w1718 _]
                  tunnel: w1670 -> [w1716 _]
                  tunnel: w1669 -> [w1715 _]
                  tunnel: w1668 -> [w1686 w1725]
                  tunnel: w1667 -> [w1684 w1727]
                  tunnel: [w1683 w1727] -> w1666
                  tunnel: w1663 -> [w1682 _]
                  frame False {
                    w1713 = i16 4 ("precision (6)")
                    # "If both Cpk and Cp are Decimal numbers."
                    n552 = Unbundle By Name(w1715) -> ("LSL"=w1714:dbl, "USL"=w1712:dbl, "Nominal Value"=w1711:dbl, "LCL"=w1710:dbl, "UCL"=w1709:dbl)
                    n553 = Increment(x=w1684) -> (x+1=w1683:u32)
                    n554 = Number To Fractional String(number=w1714, precision (6)=w1713) -> (F-format string=w1708:string)  [unwired: 2 in]
                    n555 = Number To Fractional String(number=w1712, precision (6)=w1713) -> (F-format string=w1707:string)  [unwired: 2 in]
                    n556 = Number To Fractional String(number=w1711, precision (6)=w1713) -> (F-format string=w1699:string)  [unwired: 2 in]
                    n557 = Number To Fractional String(number=w1710, precision (6)=w1713) -> (F-format string=w1706:string)  [unwired: 2 in]
                    n558 = Index Array(array=w1682, index=0) -> (element=w1693:string)
                    n559 = Index Array(array=w1682, index=1) -> (element=w1691:string)
                    n560 = Index Array(array=w1682, index=2) -> (element=w1689:string)
                    n561 = Index Array(array=w1682, index=3) -> (element=w1681:string)
                    n562 = Index Array(array=w1682, index=4) -> (element=w1680:string)
                    n563 = Number To Fractional String(number=w1709, precision (6)=w1713) -> (F-format string=w1705:string)  [unwired: 2 in]
                    n564 = Replace Array Subset(array=w1724, new element #1=w1720, index (row) #1=w1686, index (col) #1=0 ("disabled index (col)"), new element #2=w1718, index (row) #2=w1686, index (col) #2=1 ("disabled index (col)"), new element #3=w1716, index (row) #3=w1686, index (col) #3=2 ("disabled index (col)"), new element #4=w1708, index (row) #4=w1686, index (col) #4=3 ("disabled index (col)"), new element #5=w1707, index (row) #5=w1686, index (col) #5=4 ("disabled index (col)"), new element #6=w1699, index (row) #6=w1686, index (col) #6=5 ("disabled index (col)"), new element #7=w1706, index (row) #7=w1686, index (col) #7=6 ("disabled index (col)"), new element #8=w1705, index (row) #8=w1686, index (col) #8=7 ("disabled index (col)"), new element #9=w1693, index (row) #9=w1686, index (col) #9=8 ("disabled index (col)"), new element #10=w1691, index (row) #10=w1686, index (col) #10=9 ("disabled index (col)"), new element #11=w1689, index (row) #11=w1686, index (col) #11=10 ("disabled index (col)"), new element #12=w1681, index (row) #12=w1686, index (col) #12=11 ("disabled index (col)"), new element #13=w1680, index (row) #13=w1686, index (col) #13=12 ("disabled index (col)")) -> (w1723:string[][])
                    n565 = Increment(x=w1686) -> (x+1=w1722:i32)
                  }
                  frame True {
                    # "If either Cp or Cpk or both are -Inf/+Inf/Inf"
                  }
                }
              }
            }
          }
          n566 = in-place-cluster #6("IDs.BatchID"=w1595, "Part Info.Part Name"=w1594, "Part Info.Measurement Names Array"=w1593, "Part Info.Spec Values Array"=w1592, "StatisticalInfo"=w1591, "ExcelData.RecordsInExcelCounter.StatisticalRecordsCounter"=w1589, "Details2D.MeasurementDetails(2D)"=w1597, "IndexCounter.MeasurementDetailsIndexCounter"=w1596, "System Info.Software Features.IoT Enable"=w1588) -> (w1566:T9)
        }
        n567 = Unbundle By Name(w1566) -> ("System Info.Software Features.IoT Enable"=w1569:bool, "ExcelData.RecordsInExcelCounter.StatisticalRecordsCounter"=w1568:u32)
        n568 = case shown="False" w1569 {
          tunnel: [w1574 "Wait"] -> w1567
          tunnel: w1568 -> [w1578 _]
          tunnel: [w1576 w1586] -> w1565
          tunnel: w1566 -> [w1575 w1586]
          frame False {
            # "IoT Disabled"
            n569 = Less?(x=w1578, y=u32 10001) -> (x < y?=w1577:bool)
            n570 = case shown="True" w1577 {
              tunnel: [w1581 w1585] -> w1576
              tunnel: w1575 -> [w1583 w1585]
              tunnel: ["ExcelFolderCreation" "Wait"] -> w1574
              frame False {
                n571 = Bundle By Name(cluster=w1583, "ExcelData.CreateNewExcel.CreateNewStatisticalExcel"=TRUE ("ExcelData.CreateNewExcel.CreateNewFailExcel")) -> (w1581:T9)
              }
              frame True {
              }
            }
          }
          frame True {
            # "IoT Enabled"
          }
        }
        n572 = call <vilib>:"Add State(s) to Queue__JKI_lib_State_Machine.vi"("State(s) in Front (\"\")"=w1567, "State(s) in (\"\")"=w1572) -> ("States Out"=w1573:string)  [unwired: 13 in]
      }
      frame "ShiftStatisticalInfo" {
        # "File Open problem won't be coming as every time we are writing\nto a new Excel file.\n\nDuring Exit SM won't be sending Shift End data.So no need to check\nthere is data or not during exit (For sending Save Ack to SM)."
        n573 = Unbundle By Name(w1755) -> ("ShiftSPCExcelPath"=w1741:path)
        n574 = Unbundle By Name(w1754) -> ("Shift Statistical Info.Shift End Date"=w1746:string, "Shift Statistical Info.Shift Name"=w1745:string, "Shift Statistical Info.Shift Timing"=w1729:string, "Shift Statistical Info.Statistical Shift Data"=w1747:T14)
        n575 = Search and Replace String(replace all?=TRUE ("replace all? (F)"), input string=w1729, search string=":", replace string="." ("replace string (\"\")")) -> (result string=w1730:string)  [unwired: 4 in, 3 out]
        n576 = call <vilib>:"Space Constant.vi"() -> ("String"=w1733:string)
        n577 = Concatenate Strings("Shift SPC Data" ("string"), w1733, w1746, w1733, w1745, w1733, "(" ("string"), w1730, ").csv" ("string")) -> (w1750:string)
        n578 = call <vilib>:"Check if File or Folder Exists.vi"("error in (no error)"=w1734, "path"=w1741) -> ("error out"=w1744:errorcluster, "file or folder exists?"=w1742:bool, "dup path"=w1743:path)  [unwired: 7 in]
        n579 = case shown="False" w1742 {
          tunnel: w1743 -> [w1758 w1763]
          tunnel: [w1759 w1762] -> w1736
          tunnel: w1744 -> [w1759 w1761]
          tunnel: [w1758 w1760] -> w1740
          frame True {
          }
          frame False {
            n580 = Create Folder(path (use dialog)=w1763, error in=w1761) -> (created path=w1760:path, error out=w1762:errorcluster)  [unwired: 1 in, 1 out]
          }
        }
        n581 = Build Path(base path=w1740, name or relative path=w1750) -> (appended path=w1738:path)
        n582 = call "Write Shift Statistical Data To Excel.vi"("Shift Timing"=w1729, "Shift Name"=w1745, "Shift End Date"=w1746, "Statistical Shift Data"=w1747) -> ("Array"=w1739:string[][])  [unwired: 7 in]
        n583 = call-poly <vilib>:"Write Delimited Spreadsheet.vi"("file path (dialog if empty)"=w1738, "2D data"=w1739, "append to file? (new file:F)"=TRUE ("append to file? (F)"), "error in (no error)"=w1736, "delimiter (\\t)"="," ("delimiter (\\t)")) -> ("error out"=w1737:errorcluster)  [unwired: 9 in, 1 out]
        n584 = call <vilib>:"Clear Errors.vi"("error in (no error)"=w1737) -> ("error out"=w1735:errorcluster)  [unwired: 5 in, 1 out]
        n585 = call <vilib>:"Add State(s) to Queue__JKI_lib_State_Machine.vi"("State(s) in (\"\")"=w1756) -> ("States Out"=w1757:string)  [unwired: 14 in]
      }
      frame "BatchInfo" {
        n586 = in-place {
          n587 = in-place-cluster #7(w1769) -> ("IDs.BatchID"=w1799:string, "Part Info.Part Name"=w1798:string, "IDs.Stamping McID"=w1797:string, "IDs.Inspection McID"=w1796:string, "Part Info.Operator Name"=w1794:string, "Part Info.ReelCount"=w1793:u64, "BatchInfo.BatchPassCount"=w1792:u64, "BatchInfo.BatchFailCount"=w1791:u64, "ExcelData.RecordsInExcelCounter.ReelRecordsCounter"=w1787:u32, "IndexCounter.BatchDetailsIndexCounter"=w1800:i32, "Details2D.BatchDetails(2D)"=w1790:string[][])
          n588 = Number To Decimal String(number=w1793) -> (decimal integer string=w1807:string)  [unwired: 1 in]
          n589 = Number To Decimal String(number=w1792) -> (decimal integer string=w1804:string)  [unwired: 1 in]
          n590 = Number To Decimal String(number=w1791) -> (decimal integer string=w1803:string)  [unwired: 1 in]
          n591 = Increment(x=w1787) -> (x+1=w1788:u32)
          n592 = Replace Array Subset(array=w1790, new element #1=w1799, index (row) #1=w1800, index (col) #1=0 ("disabled index (col)"), new element #2=w1798, index (row) #2=w1800, index (col) #2=1 ("disabled index (col)"), new element #3=w1797, index (row) #3=w1800, index (col) #3=2 ("disabled index (col)"), new element #4=w1796, index (row) #4=w1800, index (col) #4=3 ("BatchDetailsIndexCounter"), new element #5=w1794, index (row) #5=w1800, index (col) #5=4 ("disabled index (col)"), new element #6=w1807, index (row) #6=w1800, index (col) #6=5 ("disabled index (col)"), new element #7=w1804, index (row) #7=w1800, index (col) #7=6 ("disabled index (col)"), new element #8=w1803, index (row) #8=w1800, index (col) #8=7 ("disabled index (col)")) -> (w1789:string[][])
          n593 = Increment(x=w1800) -> (x+1=w1801:i32)
          n594 = in-place-cluster #7("IDs.BatchID"=w1799, "Part Info.Part Name"=w1798, "IDs.Stamping McID"=w1797, "IDs.Inspection McID"=w1796, "Part Info.Operator Name"=w1794, "Part Info.ReelCount"=w1793, "BatchInfo.BatchPassCount"=w1792, "BatchInfo.BatchFailCount"=w1791, "ExcelData.RecordsInExcelCounter.ReelRecordsCounter"=w1788, "IndexCounter.BatchDetailsIndexCounter"=w1801, "Details2D.BatchDetails(2D)"=w1789) -> (w1766:T9)
        }
        n595 = Unbundle By Name(w1766) -> ("System Info.Software Features.IoT Enable"=w1767:bool, "ExcelData.RecordsInExcelCounter.ReelRecordsCounter"=w1768:u32)
        n596 = case shown="False" w1767 {
          tunnel: [w1773 "Wait"] -> w1764
          tunnel: w1768 -> [w1777 _]
          tunnel: [w1775 w1785] -> w1765
          tunnel: w1766 -> [w1774 w1785]
          frame False {
            # "IoT Disabled"
            n597 = Less?(x=w1777, y=u32 10001) -> (x < y?=w1776:bool)
            n598 = case shown="False" w1776 {
              tunnel: [w1780 w1784] -> w1775
              tunnel: w1774 -> [w1782 w1784]
              tunnel: ["ExcelFolderCreation" "Wait"] -> w1773
              frame False {
                n599 = Bundle By Name(cluster=w1782, "ExcelData.CreateNewExcel.CreateNewReelExcel"=TRUE ("ExcelData.CreateNewExcel.CreateNewFailExcel")) -> (w1780:T9)
              }
              frame True {
              }
            }
          }
          frame True {
            # "IoT Enabled"
          }
        }
        n600 = call <vilib>:"Add State(s) to Queue__JKI_lib_State_Machine.vi"("State(s) in Front (\"\")"=w1764, "State(s) in (\"\")"=w1771) -> ("States Out"=w1772:string)  [unwired: 13 in]
      }
      frame "ActionBasedOnStateMessage" {
        n601 = Unbundle By Name(w1814) -> ("SaveAck"=w1816:cluster{"Loop1":bool, "Loop2":bool}, "CurrentStateMessage"=w1830:string, "System Info.Software Features.IoT Enable"=w1829:bool, "IndexCounter.EventDetailsIndexCounter"=w1824:i32, "SetCounter.EventDetailsSetCounter"=w1823:i32, "IndexCounter.FailureDetailsIndexCounter"=w1822:i32, "SetCounter.FailureDetailsSetCounter"=w1821:i32, "IndexCounter.BatchDetailsIndexCounter"=w1820:i32, "SetCounter.BatchDetailsSetCounter"=w1819:i32, "IndexCounter.MeasurementDetailsIndexCounter"=w1818:i32, "SetCounter.MeasurementDetailsSetCounter"=w1817:i32, "System Info.Software Features.Datalogging Features.Measurement Data"=w1812:bool)
        n602 = Not Equal?(x=w1824, y=0) -> (x != y?=w1846:bool)
        n603 = Greater?(x=w1824, y=w1823) -> (0:w1845:bool)
        n604 = Not Equal?(x=w1822, y=0) -> (x != y?=w1843:bool)
        n605 = Greater?(x=w1822, y=w1821) -> (0:w1844:bool)
        n606 = Not Equal?(x=w1820, y=0) -> (x != y?=w1839:bool)
        n607 = Greater?(x=w1820, y=w1819) -> (0:w1838:bool)
        n608 = Not Equal?(x=w1818, y=0) -> (x != y?=w1837:bool)
        n609 = Greater?(x=w1818, y=w1817) -> (0:w1836:bool)
        n610 = Compound Arithmetic op=AND(w1846, w1845) -> (w1835:bool)
        n611 = Compound Arithmetic op=AND(w1843, w1844) -> (w1834:bool)
        n612 = Compound Arithmetic op=AND(w1839, w1838) -> (w1833:bool)
        n613 = Compound Arithmetic op=AND(w1837, w1836) -> (w1832:bool)
        n614 = Compound Arithmetic op=OR(w1835, w1834, w1833, w1832) -> (w1831:bool)
        n615 = case shown="False" w1831 {
          tunnel: [w1857 "SaveToDrive"] -> w1826
          tunnel: w1830 -> [w1858 _]
          tunnel: w1827 -> [w1856 w1902]
          tunnel: w1828 -> [w1855 _]
          tunnel: w1829 -> [w1854 _]
          tunnel: w1816 -> [w1853 _]
          tunnel: w1814 -> [w1852 w1903]
          tunnel: [w1851 w1902] -> w1815
          tunnel: [w1850 w1903] -> w1813
          tunnel: w1812 -> [w1849 _]
          frame False {
            n616 = case shown="\"Save\"" w1858 {
              tunnel: ["Wait" w1891 "Wait"] -> w1857
              tunnel: w1856 -> [w1865 w1890 w1900]
              tunnel: w1855 -> [w1864 _ _]
              tunnel: w1854 -> [_ w1892 _]
              tunnel: w1853 -> [w1863 _ _]
              tunnel: w1852 -> [w1862 w1888 w1899]
              tunnel: [w1861 w1887 w1900] -> w1851
              tunnel: [w1860 w1889 w1899] -> w1850
              tunnel: w1849 -> [w1859 _ _]
              frame "Save" {
                n617 = case shown="True" w1859 {
                  tunnel: w1865 -> [w1870 w1874]
                  tunnel: w1864 -> [w1868 w1872]
                  tunnel: w1863 -> [_ _]
                  tunnel: w1862 -> [w1867 w1876]
                  tunnel: [w1869 w1873] -> w1861
                  tunnel: [w1867 w1875] -> w1860
                  frame False {
                    # "Writting Measurement Data is Disabled."
                    n618 = call "Output_DL.vi"("Private Data"=w1868, "error in (no error)"=w1870, "State"="SaveACK") -> ("error out"=w1869:errorcluster)  [unwired: 8 in]
                  }
                  frame True {
                    # "Writting Measurement Data is Enabled."
                    n619 = Unbundle By Name(w1876) -> ("SaveAck.Loop2"=w1877:bool)
                    n620 = case shown="False" w1877 {
                      tunnel: w1874 -> [w1878 w1885]
                      tunnel: [w1880 w1883] -> w1875
                      tunnel: w1872 -> [_ w1882]
                      tunnel: w1876 -> [w1881 w1883]
                      tunnel: [w1878 w1884] -> w1873
                      frame False {
                        n621 = Bundle By Name(cluster=w1881, "SaveAck.Loop1"=TRUE ("SaveAck")) -> (w1880:T9)
                      }
                      frame True {
                        n622 = call "Output_DL.vi"("Private Data"=w1882, "error in (no error)"=w1885, "State"="SaveACK") -> ("error out"=w1884:errorcluster)  [unwired: 8 in]
                      }
                    }
                  }
                }
              }
              frame "Post" {
                n623 = case shown="False" w1892 {
                  tunnel: ["Wait" "PushToCreator"] -> w1891
                  tunnel: [w1894 w1897] -> w1887
                  tunnel: w1890 -> [w1894 w1897]
                  tunnel: [w1893 w1896] -> w1889
                  tunnel: w1888 -> [w1893 w1896]
                  frame False {
                  }
                  frame True {
                  }
                }
              }
              frame Default {
              }
            }
          }
          frame True {
          }
        }
        n624 = call <vilib>:"Add State(s) to Queue__JKI_lib_State_Machine.vi"("State(s) in Front (\"\")"=w1826, "State(s) in (\"\")"=w1825) -> ("States Out"=w1848:string)  [unwired: 13 in]
      }
      frame "SaveToDrive" {
        n625 = call "SaveToDrive.vi"("error in"=w1909, "DataLogger IN"=w1905, "Cluster IN"=w1906) -> ("error out"=w1908:errorcluster, "Cluster OUT"=w1907:T9)  [unwired: 7 in]
        n626 = call <vilib>:"Add State(s) to Queue__JKI_lib_State_Machine.vi"("State(s) in Front (\"\")"="Wait" ("State(s) in Front (\"\")"), "State(s) in (\"\")"=w1911) -> ("States Out"=w1912:string)  [unwired: 13 in]
      }
      frame "PushToCreator" {
        n627 = Unbundle By Name(w1928) -> ("Gtron DataBase Path"=w1937:path, "ActionBasedOnStateMessage"=w1922:refnum<user-event>)
        n628 = Unbundle By Name(w1924) -> ("IoTDetailsCounter"=w1925:bool)
        n629 = case shown="True" w1925 {
          tunnel: w1937 -> [_ w1955]
          tunnel: w1936 -> [w1948 w1954]
          tunnel: [w1948 w1953] -> w1934
          tunnel: [w1947 w1950] -> w1926
          tunnel: [w1947 w1949] -> w1921
          frame False {
            w1947 = FALSE
          }
          frame True {
            n630 = call "POST IoT Config Details.vi"("GTron in"=w1955, "error in"=w1954) -> ("IsEmpty"=w1949:bool, "error out"=w1953:errorcluster)  [unwired: 6 in]
            n631 = Select(t=TRUE, s=w1949, f=FALSE) -> (s? t:f=w1950:bool)
          }
        }
        n632 = call "UpdateSequence.vi"("error in"=w1936, "Cluster IN"=w1924, "DataLogger in"=w1928) -> ("error out"=w1935:errorcluster, "UpdateComplete"=w1920:bool, "Cluster OUT"=w1927:T9)  [unwired: 6 in]
        n633 = call "POST Batch Details.vi"("GTron in"=w1937, "error in"=w1936) -> ("IsEmpty"=w1915:bool, "error out"=w1933:errorcluster)  [unwired: 12 in]
        n634 = call "POST Event Details.vi"("error in"=w1936, "GTron in"=w1937) -> ("error out"=w1932:errorcluster, "IsEmpty"=w1916:bool)  [unwired: 8 in]
        n635 = call "POST Failure Details.vi"("GTron in"=w1937, "error in"=w1936) -> ("IsEmpty"=w1917:bool, "error out"=w1931:errorcluster)  [unwired: 5 in]
        n636 = call "POST Measurement Details.vi"("GTron in"=w1937, "error in"=w1936) -> ("IsEmpty"=w1918:bool, "error out"=w1930:errorcluster)  [unwired: 6 in]
        n637 = Compound Arithmetic op=OR(w1920, w1921, w1915, w1916, w1917, w1918) -> (w1919:bool)
        n638 = Merge Errors(w1935, w1934, w1933, w1932, w1931, w1930) -> (w1913:errorcluster)
        n639 = Bundle By Name(cluster=w1927, "IoTDetailsCounter"=w1926) -> (w1923:T9)
        n640 = call <vilib>:"Clear Errors.vi"("error in (no error)"=w1913) -> ("error out"=w1914:errorcluster)  [unwired: 5 in, 1 out]
        n641 = case shown="True" w1919 {
          tunnel: w1914 -> [w1941 w1946]
          tunnel: [w1941 w1945] -> w1929
          tunnel: w1922 -> [_ w1943]
          frame False {
            # "No records available for adding or update"
          }
          frame True {
            n642 = Wait (ms)(milliseconds to wait=u32 300) -> ()  [unwired: 1 out]
            n643 = Generate User Event(user event=w1943, event data cluster="" ("event data"), error in=w1946) -> (error out=w1945:errorcluster)  [unwired: 1 in, 1 out]
          }
        }
        n644 = call <vilib>:"Add State(s) to Queue__JKI_lib_State_Machine.vi"("State(s) in Front (\"\")"="Wait" ("State(s) in Front (\"\")"), "State(s) in (\"\")"=w1939) -> ("States Out"=w1940:string)  [unwired: 13 in]
      }
    }
  }
  n645 = Merge Errors(w16, w14) -> (→"error out":errorcluster)
